vi "TLB Native Dynamic Events ver 0.18.vi"() -> ()   [LabVIEW 2018]
uses:
  Labview Training Phase 2/Enum Controls/States for Action Engine.ctl
  TLB Type Definitions/State Type Definitions, for 0.26g versions and later 2.ctl
  TLB Type Definitions/Intruction Type Definitions.ctl
  TLB Type Definitions/Encoder cluster.ctl
  TLB Type Definitions/PING CLUSTER.ctl
  <vilib>/Studica/Studica Toolkit/NavX/NavX.lvlib
  <vilib>/Studica/Studica Toolkit/Background/DIO Channel.ctl
  Underlying VI's/NavX VI/navX type def.ctl
  <vilib>/Studica/Studica Toolkit/Background/I2C Channel.ctl
  TLB Type Definitions/Vision cluster.ctl
  <vilib>/NI_Real-Time Target Support.lvlib
  TLB Type Definitions/Stepper cluster.ctl
  Experimental VI's/Archived VI's/MOTOR CONTROL NO PID Type Def.ctl
  Underlying VI's/I2C Master VI/I2C MASTER Type Def.ctl
  Underlying VI's/I2C Master VI/I2C_MASTER_WRITE_NEW Type Def.ctl
  <vilib>/userdefined/High Color/IMAQdx.ctl
  Underlying VI's/I2C Master VI/Arduino_Interfacing.ctl
  TLB Type Definitions/Yaw Cluster.ctl
  TLB Type Definitions/Time cluster.ctl
  TLB Type Definitions/Y Stepper cluster.ctl
  Underlying VI's/Modified webcam FGV/Webcam AE.ctl
  Underlying VI's/Elasped Timer/Elapsed timer control.ctl
  Underlying VI's/Motor Control VI with PID/MOTOR CONTROL WITH PID AE DATA MODE TYPE DEF.ctl
  Underlying VI's/Motor Control VI with PID/MOTOR CONTROL WITH PID AE DIRECTION TYPE DEF.ctl
  TLB Type Definitions/IR Sensor Type Def.ctl
  <vilib>/myRIO/Common/Instrument Driver Framework/myRIO v1.0/AI/typedefs/AI Channels Enum.ctl
  <vilib>/myRIO/Common/Instrument Driver Framework/myRIO v1.0/AI/typedefs/AI Channels List.ctl
  TLB Type Definitions/Motor Speed Cluster.ctl
  <vilib>/Utility/RT CPU Load.ctl
panel:
  out "x-y":dbl
  out "Left IR Sensor":dbl
  out "Obstacle detected":bool
  out "Speed & distance":T1
  out "Object Center Coordinates":cluster{"x":sgl, "y":sgl}
  out "Object detection cluster":T2
  out "Time up flag":bool
  out "Task selection":u8
  in  "Object recognition mode":enum16{"Ball", "Soap", "Gel", "Pipe", "None"}(ring)
  out "NavX Readings":T3
  out "Arduino Data":T4
  out "CPU loads":T5[](array[typedef]) {"ISR (%)" format="%#.2f"; "Idle (%)" format="%#.2f"; "Background (%)" format="%#.2f"; "Normal (%)" format="%#.2f"; "Above Normal (%)" format="%#.2f"; "High (%)" format="%#.2g"; "Timed Structures (%)" format="%#.2g"; "Time Critical (%)" format="%#.2g"; "Total (%)" format="%#.2g"}
  out "TASK ENABLE":bool
  out "Rising Edge":bool
  in  "Green LED":bool
  out "I2C Error":errorcluster
  out "State Logic":T6=enum."Startup"
  out "elements":T7[](array[typedef])
  in  "STOP TASK":bool
  in  "OK Button":bool
  in  "STOP":bool
  out "error out":errorcluster
  out "Action Queue Items":i32
  out "State Logic Queue Items":i32
  out "Action Queues items":string[](array[string])=["Hardware reset", "Software reset", ""]
  out "Action State":string
  # "System Health Status Update"
  # "VISION"
  # "TLB FRAMEWORK STATUS"
  # "Test Programme written by Calvin Loke    Dated: 28 Aug 2019\nTest Programme revised by Dr Alex See   Dated 30 Aug 2019\n\nRevision date: 20/03/2020\nProgramme version:   TLB Native Dynamic Events ver 0.14a"
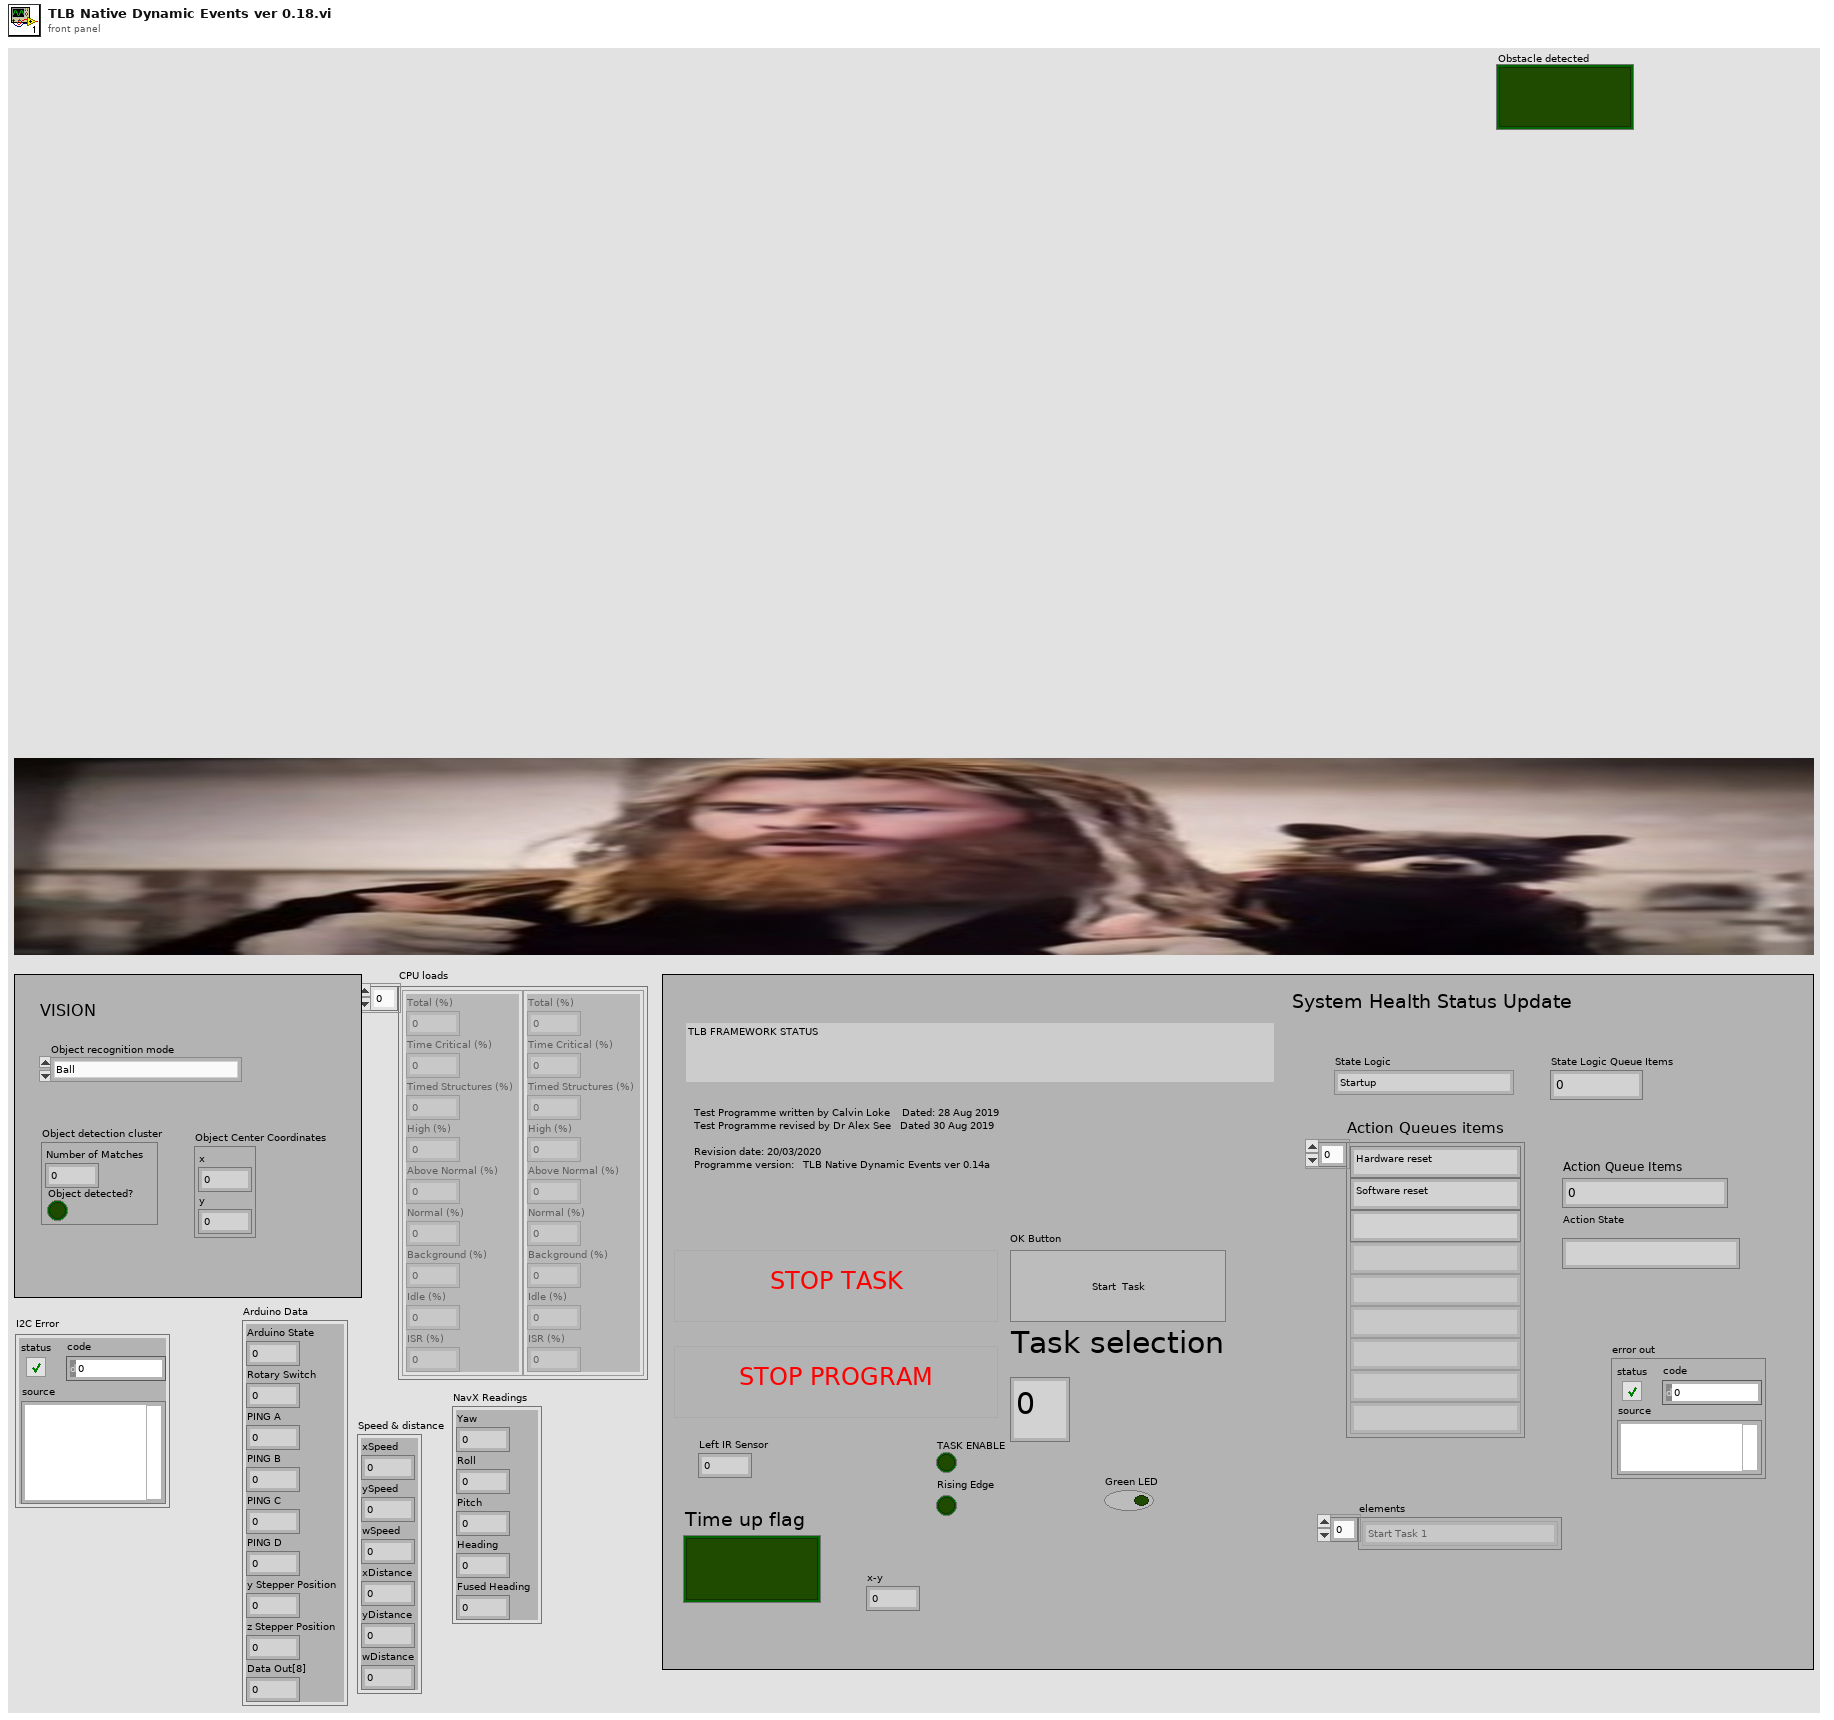
[diagram p1: front panel]
types:
  T1 = cluster{"xSpeed":dbl, "ySpeed":dbl, "wSpeed":dbl, "xDistance":dbl, "yDistance":dbl, "wDistance":dbl}
  T2 = cluster{"Number of Matches":i32, "Object detected?":bool}
  T3 = cluster{"Yaw":dbl, "Roll":dbl, "Pitch":dbl, "Heading":dbl, "Fused Heading":dbl}
  T4 = cluster{"Arduino State":u8, "Rotary Switch":u8, "PING A":u8, "PING B":u8, "PING C":u8, "PING D":u8, "y Stepper Position":u8, "z Stepper Position":u8, "Data Out[8]":u8}
  T5 = typedef "NI_Real-Time Target Support.lvlib/RT CPU Load.ctl" = cluster{"Total (%)":dbl, "Time Critical (%)":dbl, "Timed Structures (%)":dbl, "High (%)":dbl, "Above Normal (%)":dbl, "Normal (%)":dbl, "Background (%)":dbl, "Idle (%)":dbl, "ISR (%)":dbl}
  T6 = typedef "State Type Definitions, for 0.26g versions and later 2.ctl" = enum16{"None", "Startup", "Move to Angle", "True Stop", "Idle", "Shutdown", "Task 1A", "Task 1B", "Task 2:Raise Arm", "Task 2:Sensor Mode", "Task 2:Reverse Mode", "Task 3", "Task 4_A", "Task 4_B", "Task 4_C", "Task 4_D", "Task 5A", "Task 5B", "Task 5C", "Task 5D", "Task 5E: POSITION ARM", "Task 5F: ARM GRAB HEIGHT", "Task 5G: CLOSE CLAW", "Task 5H: RAISE ARM", "Task 6_A", "Task 6_B", "Task 7", "Task 8A: RAISE ARM", "Task 8B: MOVE TO BOX", "Task 8C: CAM BURST", "Task 8D: PROCESS IMAGE", "Task 8E: ROBOT ADJUST", "Task 8F: CAM BURST 2", "Task 8G: PROCESS IMAGE 2", "Task 8H: ARM ADJUST", "Task 8I: ARM GRAB HEIGHT", "Task 8J: CLOSE CLAW", "Task 8K: RAISE MY SWORD", "Task 9A: Raise Arm", "Task 9B: Rotate to Angle", "Task 9C: Detect Box", "Task 9D: MOVE FORWARD", "Task 9E: MOVE LEFT", "Task 9F: SCAN BOX", "Task 9G: MOVE RIGHT", "Task 9H: SCAN BOX 2", "Task 9I: ROTATE 90 CW", "Task 9J: FORWARD", "Task 9K: MOVE RIGHT", "Task 9L: SCAN BOX 3", "Task 9M: MOVE RIGHT", "Task 9N: SCAN BOX 4", "PENIS", "PENIS 2", "PENIS 3", "Task 9R: PROCESS COLOUR", "Task A1: Task 9 Open cam", "Task A2: Task 9 Move Arm", "Task A3: Task 9 Set Timer", "Task A4: Tasl 9 Capture images", "Task A5: Task 9 Close camera", "Task A6: Process Colour", "Task A7: Dispose Camera Buffer"}
  T7 = typedef "Intruction Type Definitions.ctl" = enum16{"None", "Start Task 1", "Start Task 2", "Start Task 3", "Start Task 4", "Start Task 5", "Start Task 6", "Start Task 7", "Start Task 8 - BALL", "Start Task 8 - Gel", "Start Task 8 - Pipe", "Start Task 8 - Soap", "Start Task 9", "Start Task A", "Start Task B", "Exit"}
  T8 = typedef "Motor Speed Cluster.ctl" = cluster{"ySpeed":dbl, "xSpeed":dbl, "wSpeed":dbl}
  T9 = typedef "IR Sensor Type Def.ctl" = cluster{"Left IR Sensor":dbl, "Arm IR Sensor":dbl, "Bottom IR Sensor":dbl}
  T10 = typedef "Y Stepper cluster.ctl" = cluster{"yStepper desired":u8}
  T11 = typedef "Time cluster.ctl" = cluster{"Time up flag":bool, "SET TIME TO CHECK":dbl}
  T12 = typedef "Yaw Cluster.ctl" = cluster{"Yaw":dbl, "Compass":dbl}
  T13 = typedef "Stepper cluster.ctl" = cluster{"y Stepper Position":u8, "z Stepper Position":u8}
  T14 = typedef "DIO Channel.ctl" = enum16{"Not Connected", "A/DIO1", "A/DIO2", "A/DIO3", "A/DIO4", "A/DIO5", "A/DIO6", "A/DIO7", "A/DIO13", "B/DIO1", "B/DIO2", "B/DIO3", "B/DIO4", "B/DIO5", "B/DIO6", "B/DIO7", "B/DIO13", "C/DIO0", "C/DIO1", "C/DIO2", "C/DIO3", "C/DIO4", "C/DIO5", "C/DIO6", "C/DIO7"}
  T15 = typedef "Vision cluster.ctl" = cluster{"Recognized Object":bool, "Object X coordinate":dbl, "Object Y coordinate":dbl}
  T16 = typedef "PING CLUSTER.ctl" = cluster{"PING_A":u8, "PING_B":u8, "PING_C":u8, "PING_D":u8}
  T17 = typedef "Encoder cluster.ctl" = cluster{"xDistance":dbl, "yDistance":dbl, "wDistance":dbl}
  T18 = cluster{"DIO Channel":T14, "FPGA VI Reference Out":refnum<k20>}
  T19 = typedef "navX type def.ctl" = enum16{"Get i2C reference", "Read Values", "Zero Yaw"}
  T20 = typedef "Arduino_Interfacing.ctl" = enum16{"Initialize", "Write to Arduino", "Read From Arduino"}
  T21 = typedef "I2C Channel.ctl" = enum16{"Not Connected", "A", "B"}
  T22 = typedef "States for Action Engine.ctl" = enum16{"Initialize", "Write", "Read"}
  T23 = cluster{"I2C Ref Out":cluster{"I2C Channel":T21, "FPGA VI Reference Out":refnum<k20>}, "Connected":bool, "Slave Address (7-bit)":u8, "Registry":u8[]}
  T24 = typedef "IMAQ Image.ctl" = refnum<image>
  T25 = typedef "Intruction Type Definitions.ctl" = enum16{"None", "Start Task 1", "Start Task 2", "Start Task 3", "Start Task 4", "Start Task 5", "Start Task 6", "Start Task 7", "Start Task 8", "Start Task 9", "Start Task A", "Start Task B", "Exit"}
  T26 = typedef "State Type Definitions.ctl" = enum16{"None", "Startup", "Move to Angle", "True Stop", "Idle", "Shutdown", "Task 1", "Task 2:Raise Arm", "Task 2:Sensor Mode", "Task 2:Reverse Mode", "Task 3", "Task 4_A", "Task 4_B", "Task 4_C", "Task 4_D", "Task 5A: ARM CAM HEIGHT", "Task 5B: MOVE TO BOX", "Task 5C: CAM BURST", "Task 5D: PROCESS IMAGE", "Task 5E: POSITION ARM", "Task 5F: ARM GRAB HEIGHT", "Task 5G: CLOSE CLAW", "Task 5H: RAISE ARM", "Task 6_A", "Task 6_B", "Task 7", "Task 8A: RAISE ARM", "Task 8B: MOVE TO BOX", "Task 8C: CAM BURST", "Task 8D: PROCESS IMAGE", "Task 8E: ROBOT ADJUST", "Task 8F: CAM BURST 2", "Task 8G: PROCESS IMAGE 2", "Task 8H: ARM ADJUST", "Task 8I: ARM GRAB HEIGHT", "Task 8J: CLOSE CLAW", "Task 8K: RAISE MY SWORD", "Task 9A: Raise Arm", "Task 9B: Rotate to Angle", "Task 9C: Rotation alignmnet", "Task B"}
  T27 = typedef "MOTOR CONTROL WITH PID AE DIRECTION TYPE DEF.ctl" = enum16{"y-axis movement", "x-axis movement", "rotation", "stop", "reset encoders"}
  T28 = typedef "MOTOR CONTROL WITH PID AE DATA MODE TYPE DEF.ctl" = enum16{"Init AE", "Write to AE", "Read from AE"}
  T29 = typedef "Elapsed timer control.ctl" = enum16{"Start", "Pause", "Initialize"}
  T30 = typedef "I2C_MASTER_WRITE_NEW Type Def.ctl" = enum16{"Ultrasonic sensors", "Stepper origin", "zStepper 13.3k", "zStepper 13k", "zStepper 12k", "zStepper 11k", "zStepper 10k", "zStepper 9k", "zStepper 8k", "zStepper 7k", "zStepper 6k", "zStepper 5k", "zStepper 4k", "zStepper 3k", "zStepper 2k", "zStepper 1k", "zStepper 900", "zStepper 800", "zStepper 700", "zStepper 600", "zStepper 500", "zStepper 400", "zStepper 300", "zStepper 200", "zStepper 100", "zStepper 0", "yStepper control", "Open Claw", "Close Claw", "Soft Reset"}
  T31 = typedef "Webcam AE.ctl" = enum16{"Initialize Camera", "Open Camera", "Continuous Acquisition", "Close Camera", "Retrieve Image", "Dispose Camera Image Buffer"}
  T32 = typedef "IMAQdx.ctl" = refnum<k21>
  T33 = typedef "Webcam AE.ctl" = enum16{"Initialize Camera", "Open Camera", "Continuous Acquisition", "Close Camera", "Retrieve Image", "Dispose Image Buffers"}
  T34 = typedef "MOTOR CONTROL NO PID Type Def.ctl" = enum16{"Init", "Front Back", "Left Right", "Rotate", "Stop", "Latch"}
  T35 = typedef "AI Channels List.ctl" = T36[]
  T36 = typedef "AI Channels Enum.ctl" = enum16{"Not Connected", "AudioIn/Left", "AudioIn/Right", "C/AI0", "C/AI1", "A/AI0", "A/AI1", "A/AI2", "A/AI3", "A/AI4", "A/AI5", "A/AI6", "A/AI7", "B/AI0", "B/AI1", "B/AI2", "B/AI3", "B/AI4", "B/AI5", "B/AI6", "B/AI7", "AI/AI0", "AI/AI1", "AI/AI2", "AI/AI3", "A/AI0 (DIFF)", "A/AI1 (DIFF)", "A/AI2 (DIFF)", "A/AI3 (DIFF)", "B/AI0 (DIFF)", "B/AI1 (DIFF)", "B/AI2 (DIFF)", "B/AI3 (DIFF)"}
  T37 = typedef "I2C MASTER Type Def.ctl" = enum16{"Last State", "Mode 0", "Mode 1", "Mode 2", "Mode 3", "Mode 4", "Mode 5", "Mode 6", "Mode 7", "Mode 8", "Mode 9", "Mode 10"}
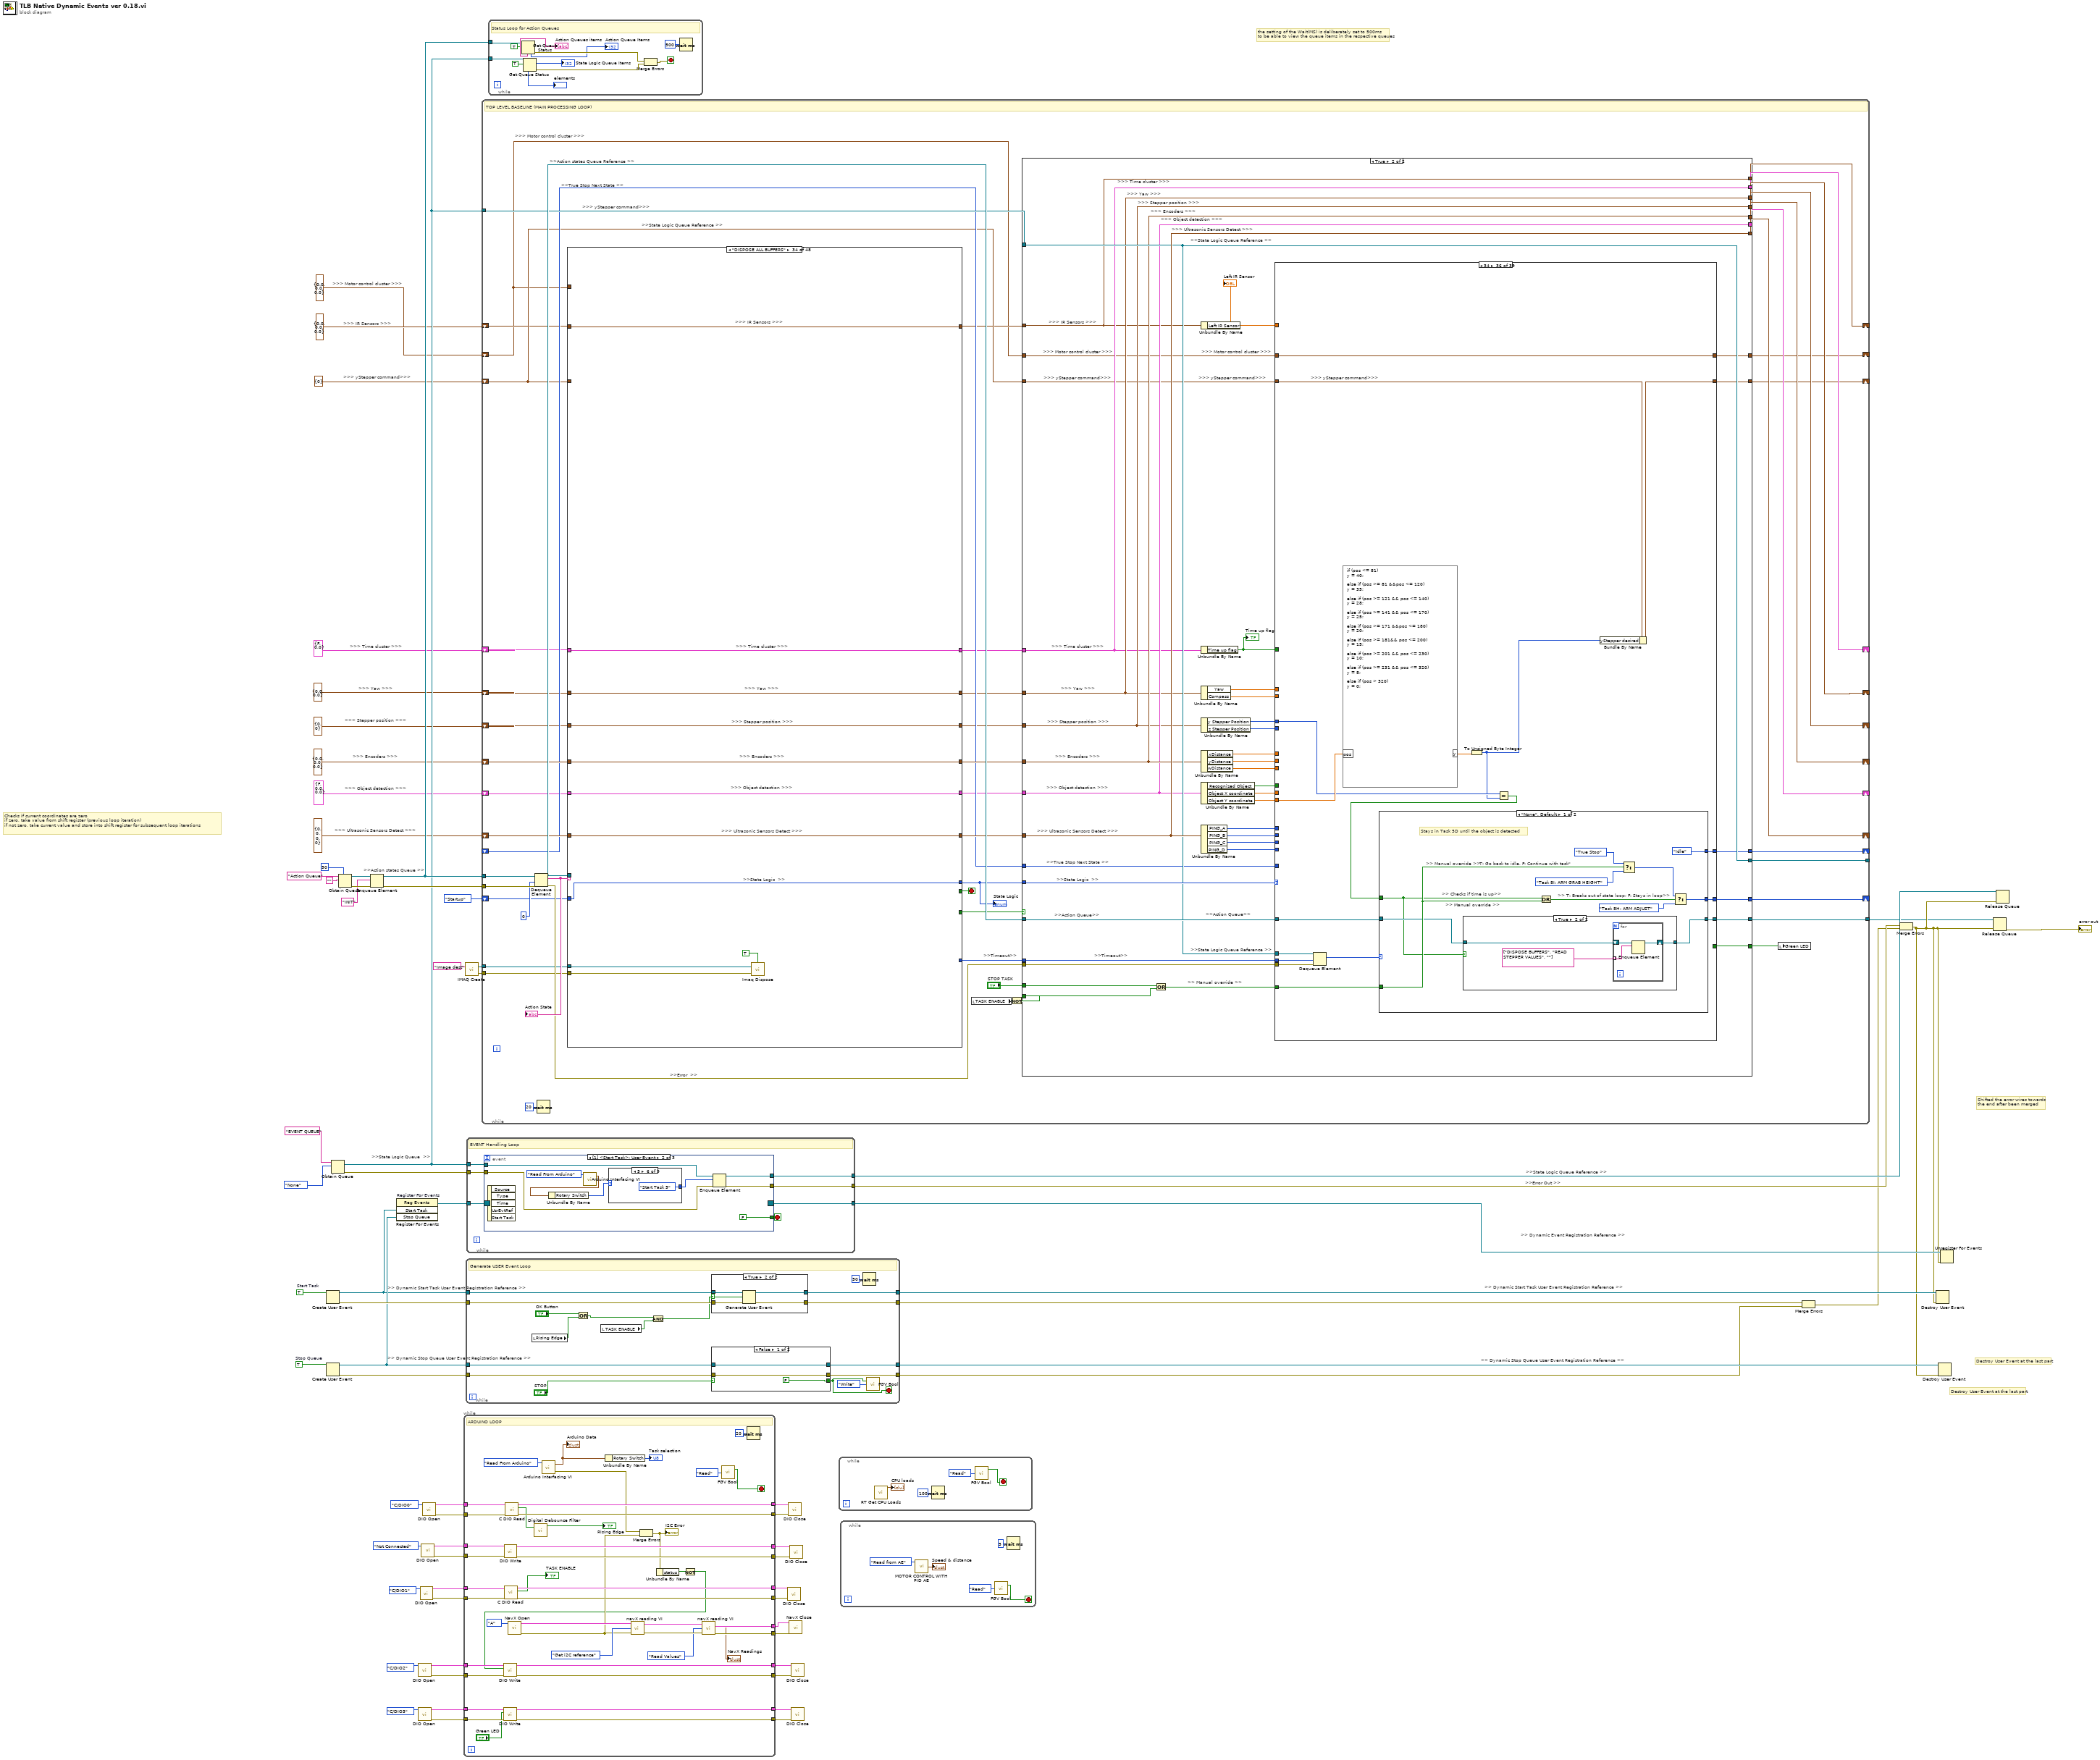
[diagram p0: block diagram]
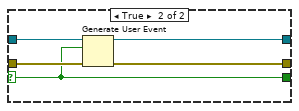
[diagram p2: hidden frame]
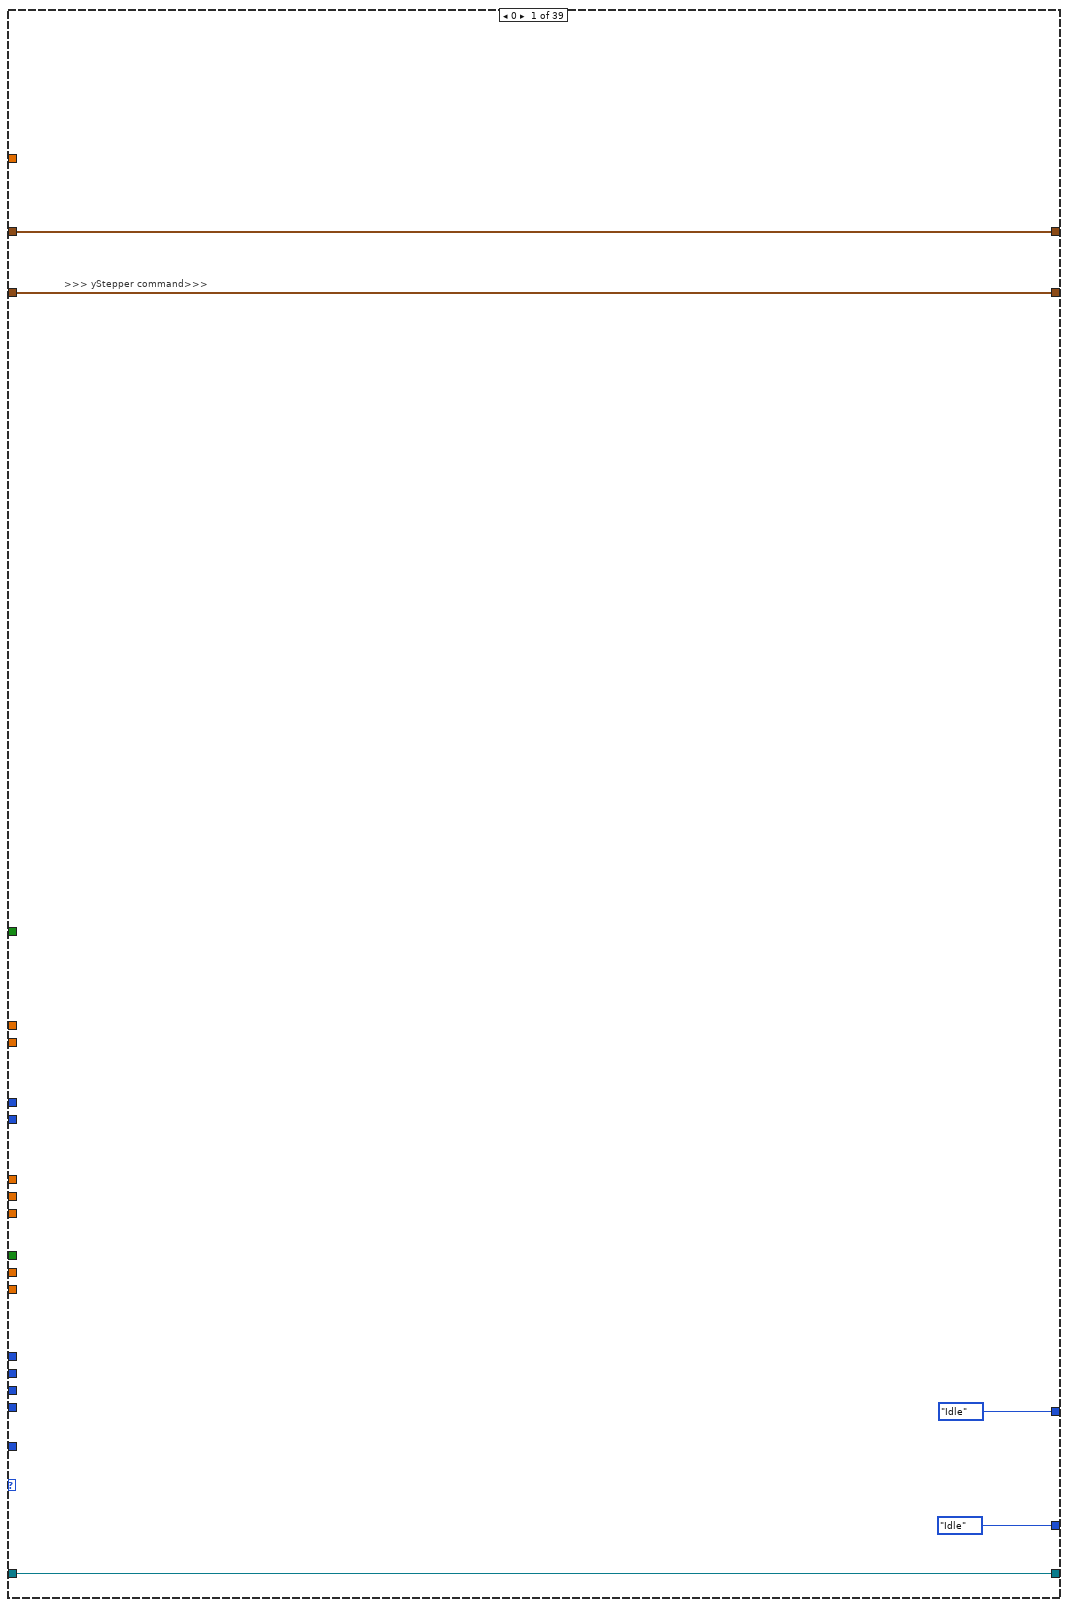
[diagram p5: hidden frame]
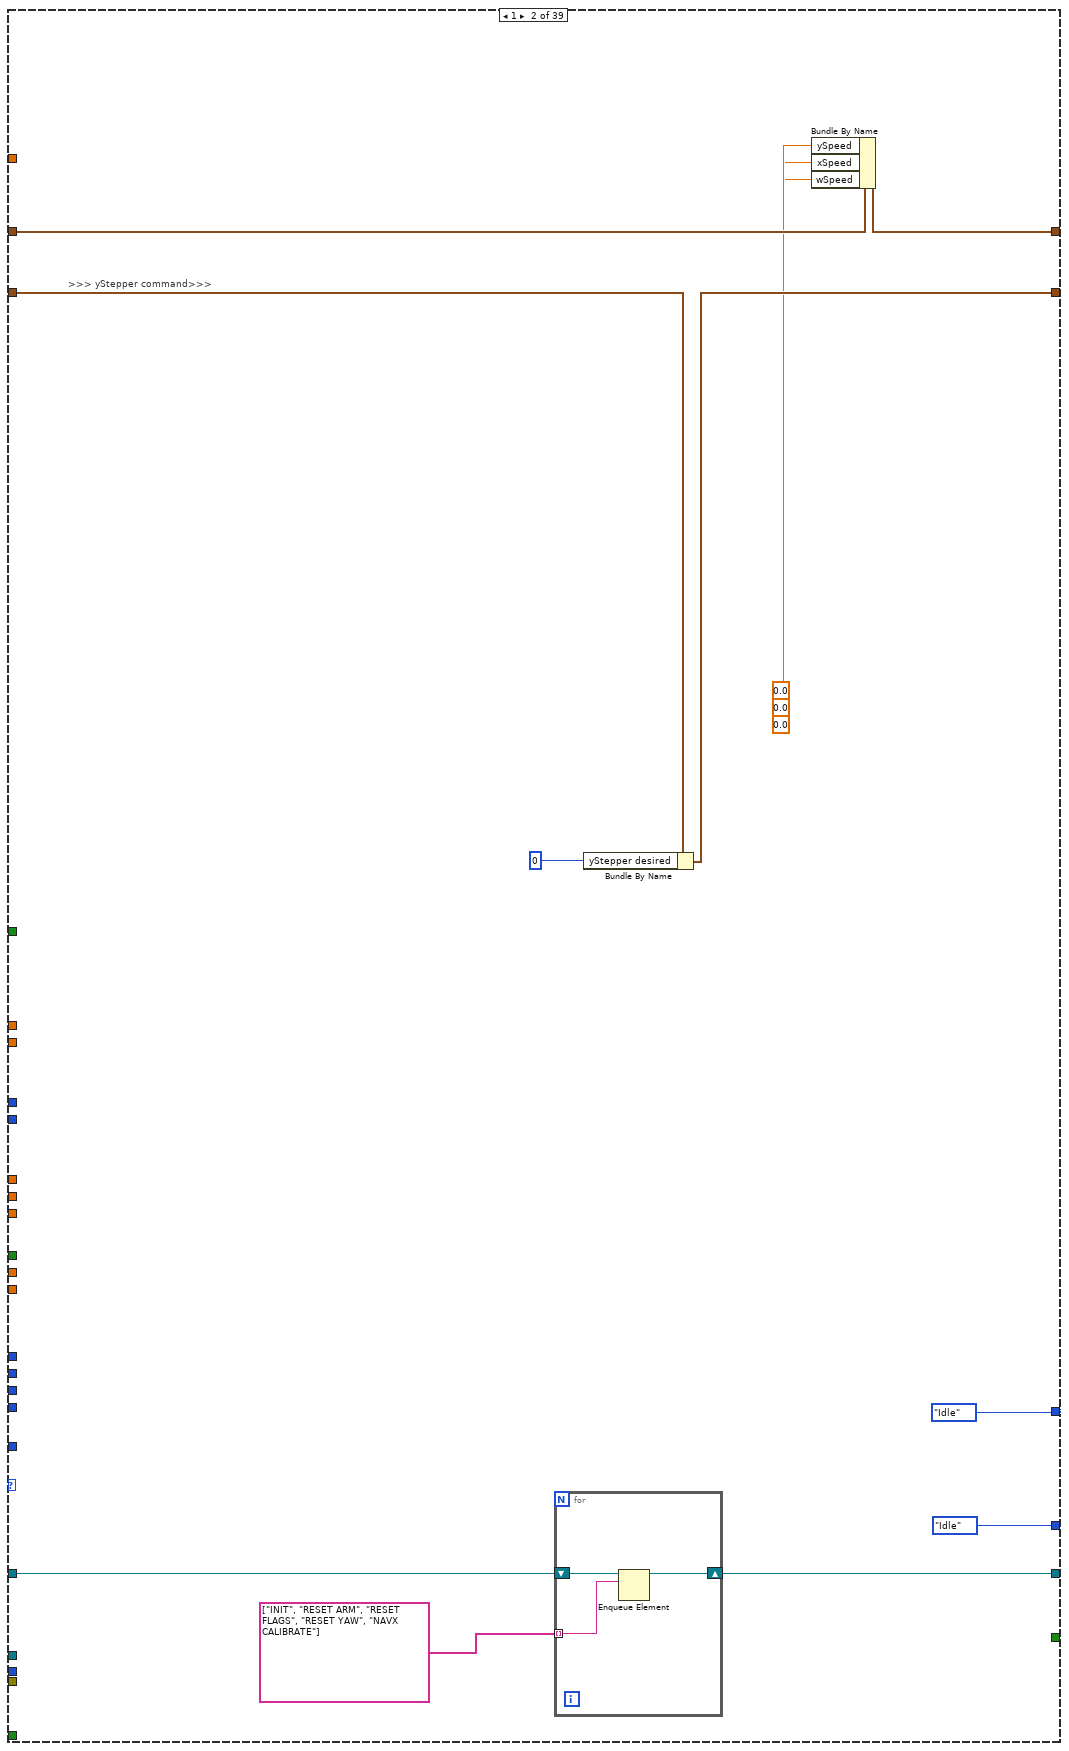
[diagram p6: hidden frame]
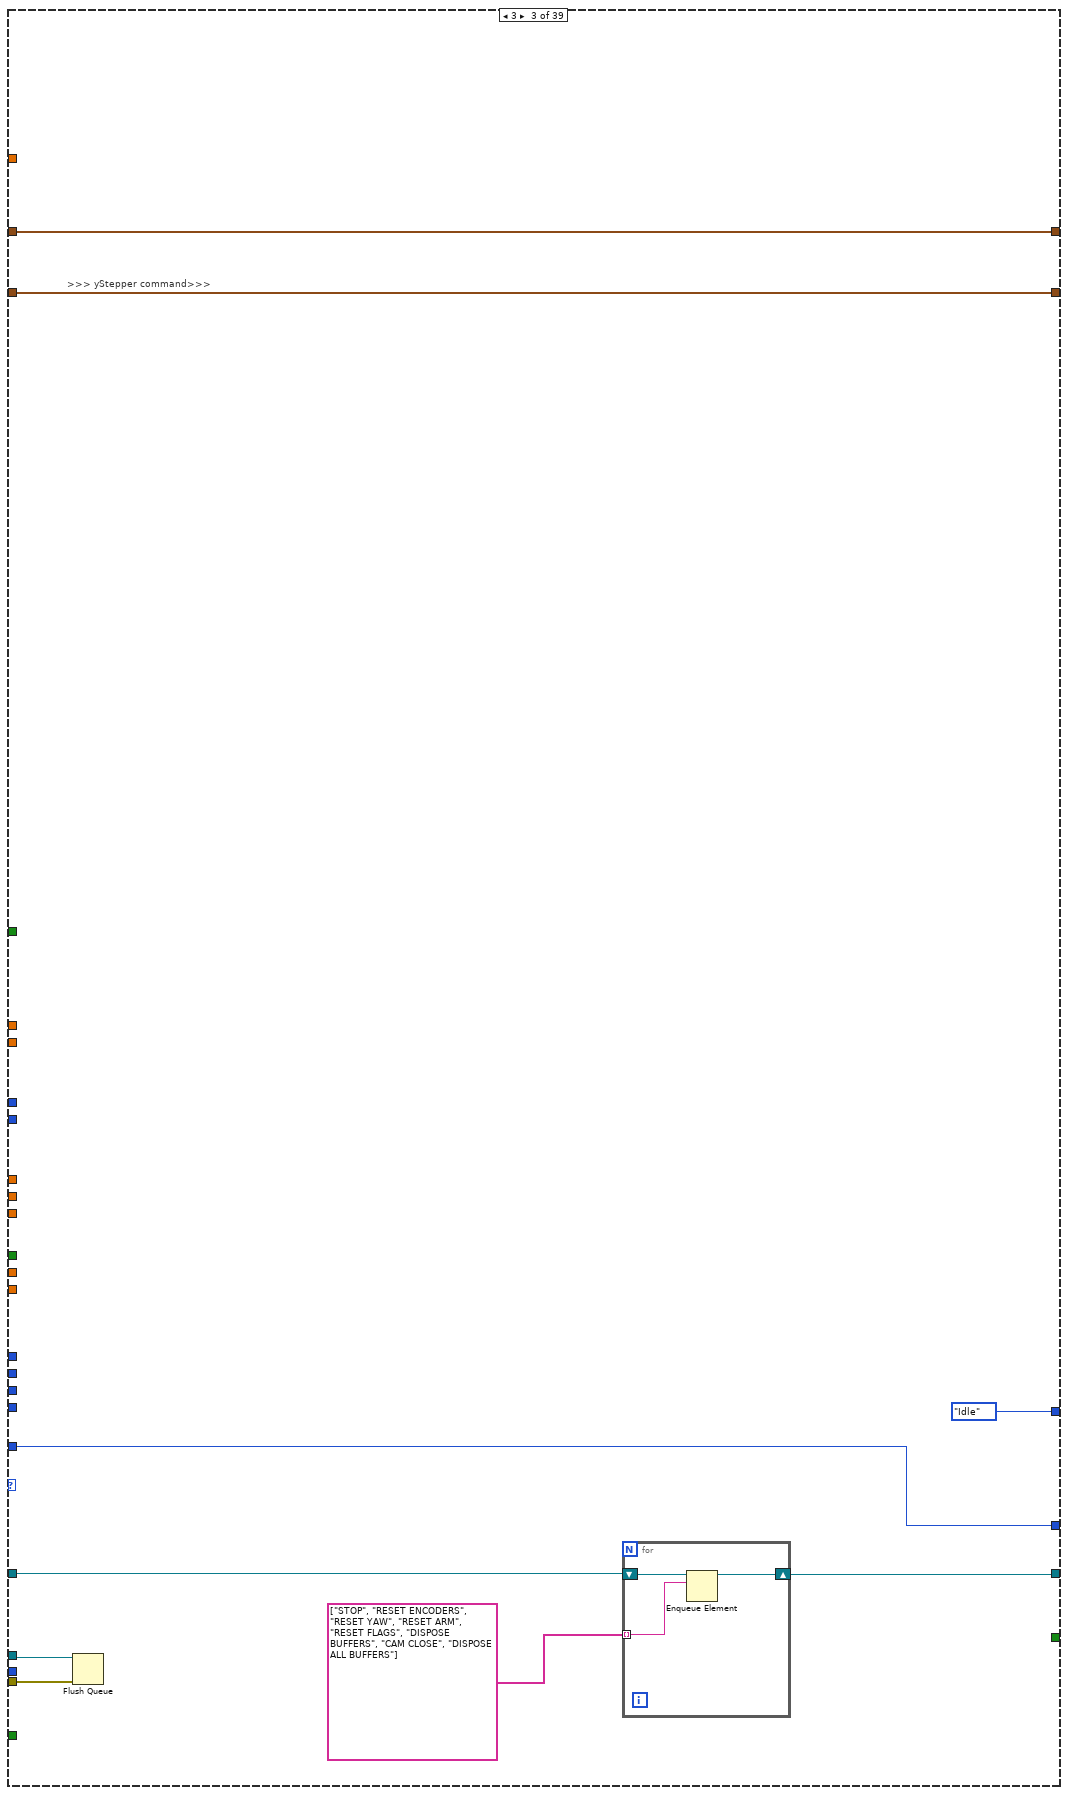
[diagram p7: hidden frame]
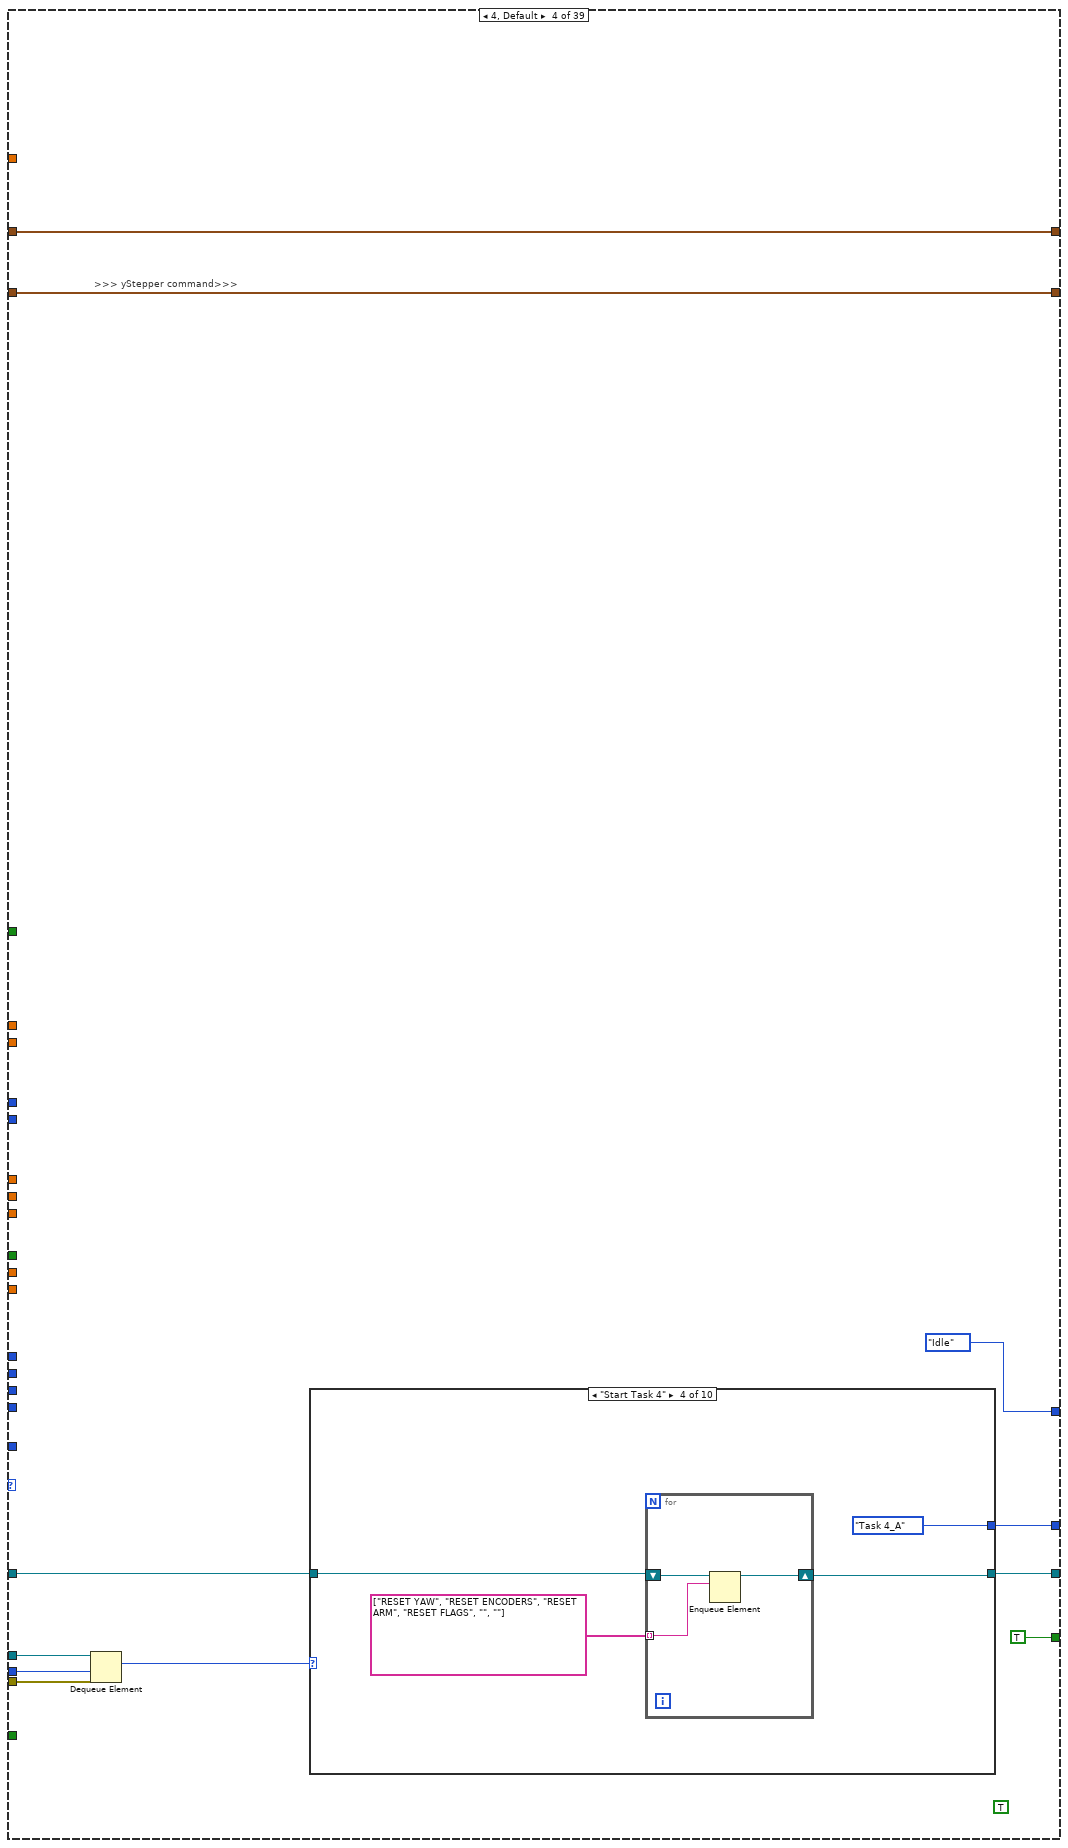
[diagram p8: hidden frame]
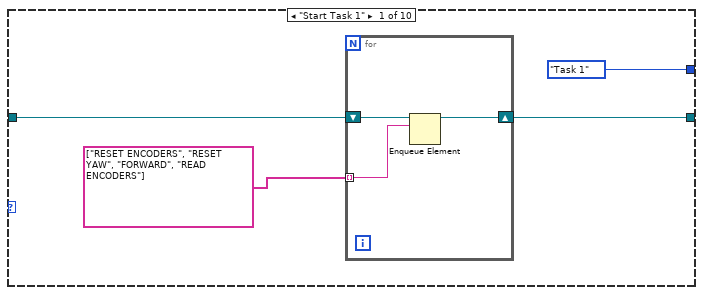
[diagram p9: hidden frame]
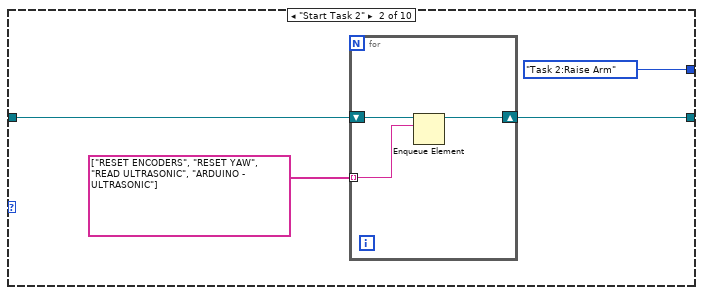
[diagram p10: hidden frame]
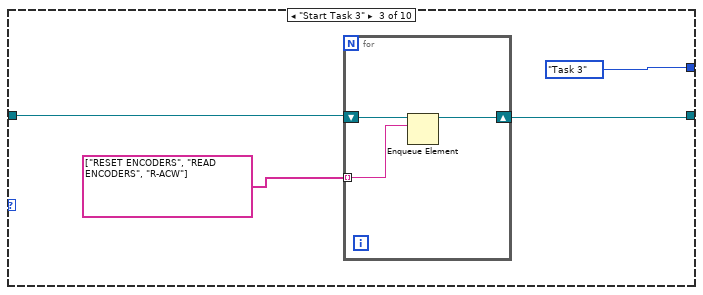
[diagram p11: hidden frame]
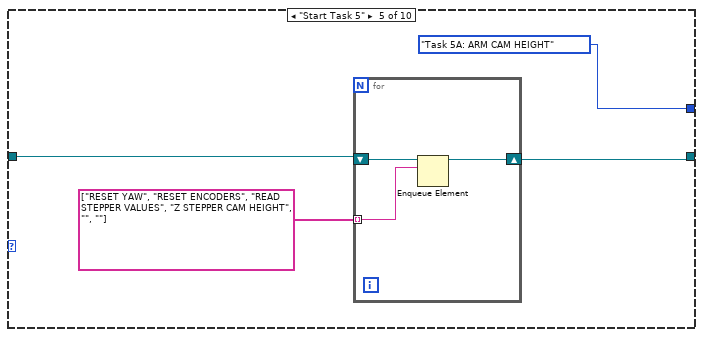
[diagram p12: hidden frame]
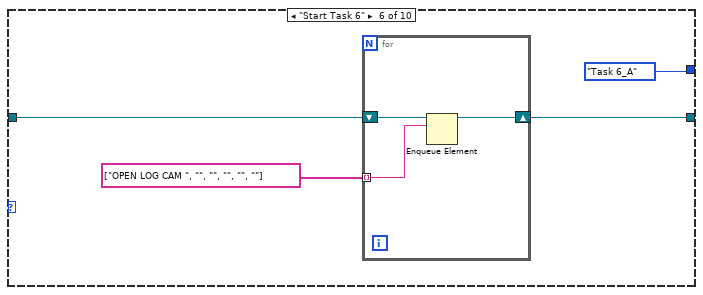
[diagram p13: hidden frame]
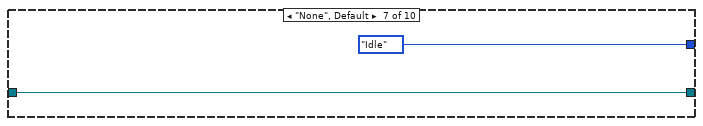
[diagram p14: hidden frame]
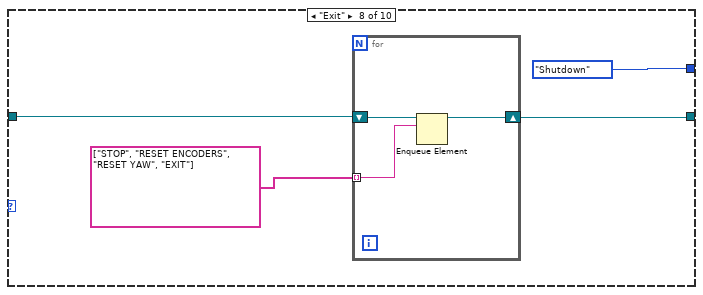
[diagram p15: hidden frame]
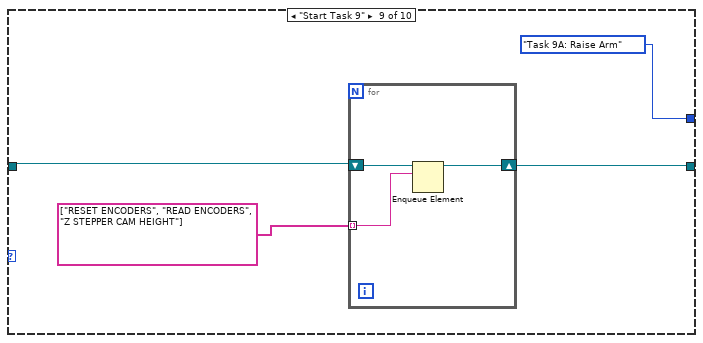
[diagram p16: hidden frame]
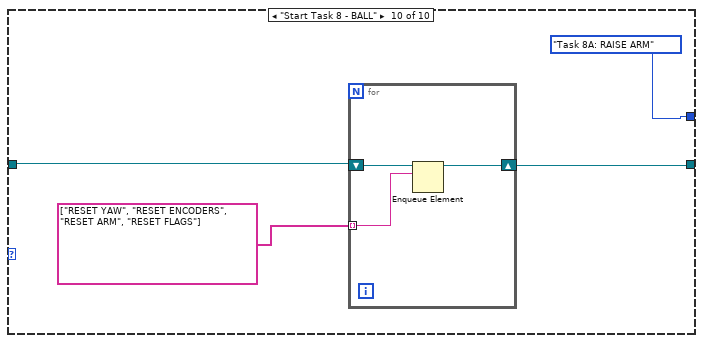
[diagram p17: hidden frame]
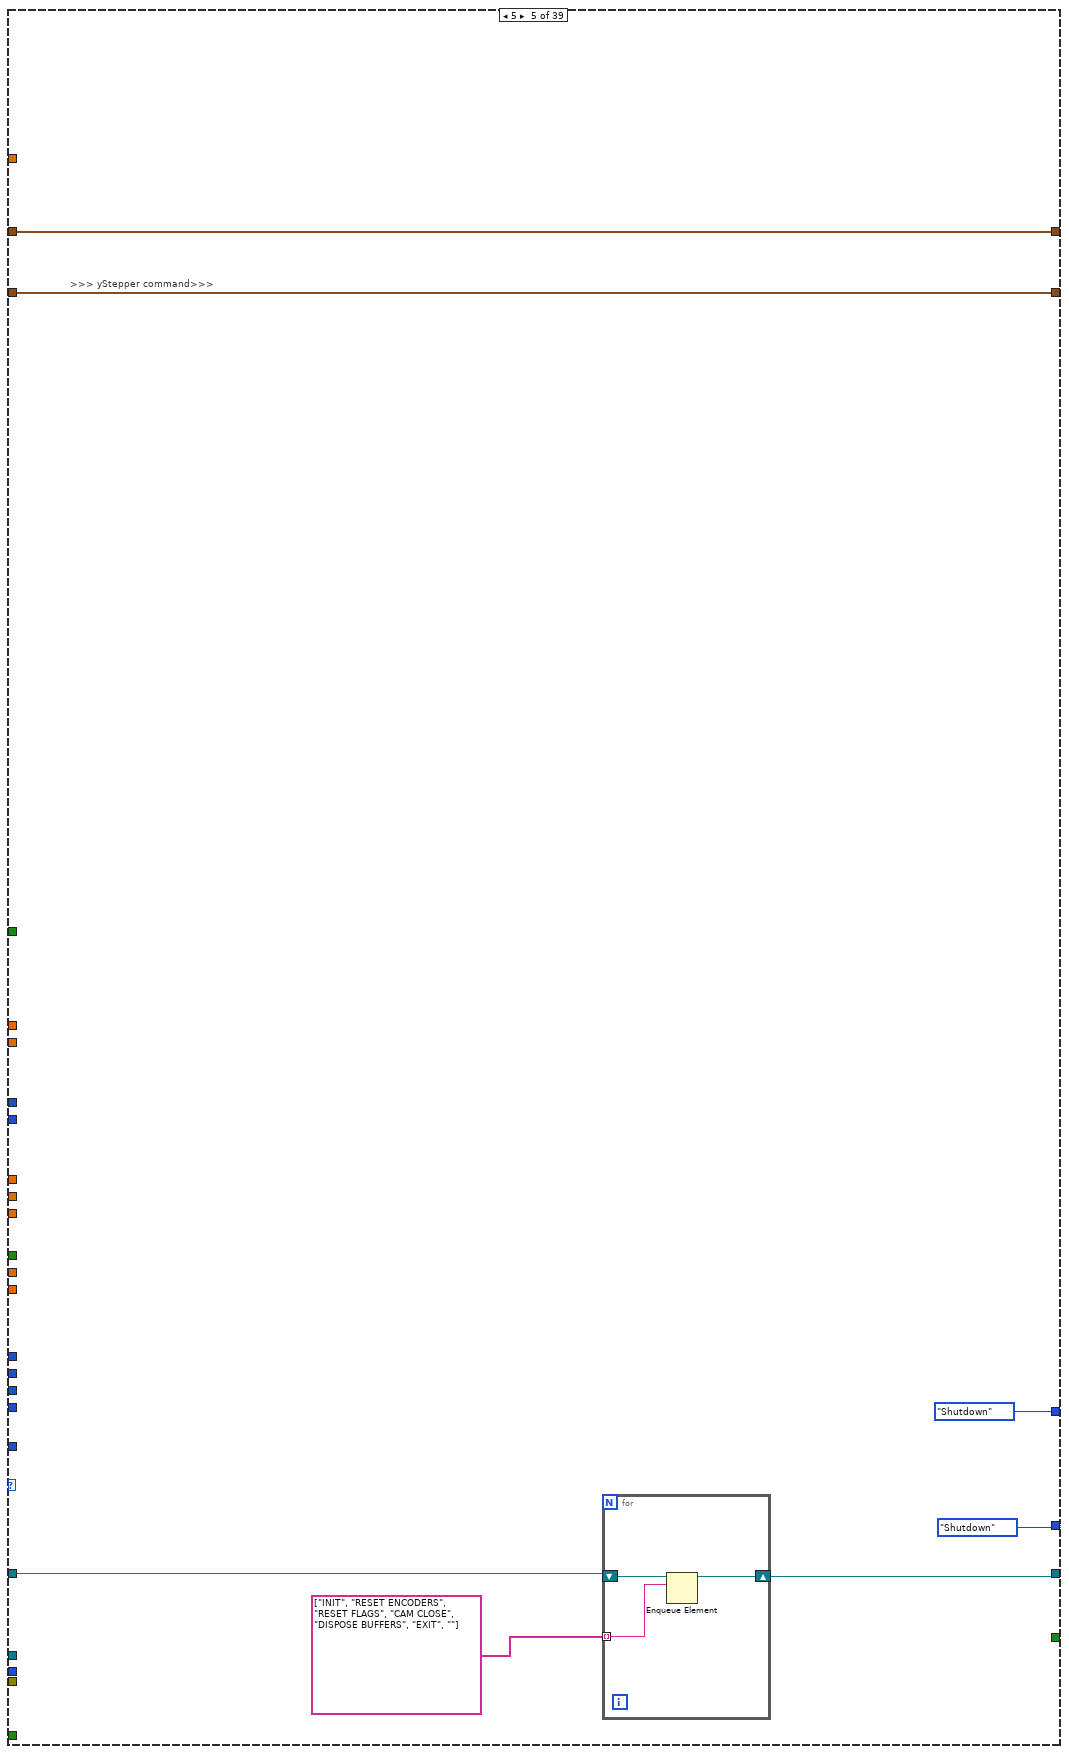
[diagram p18: hidden frame]
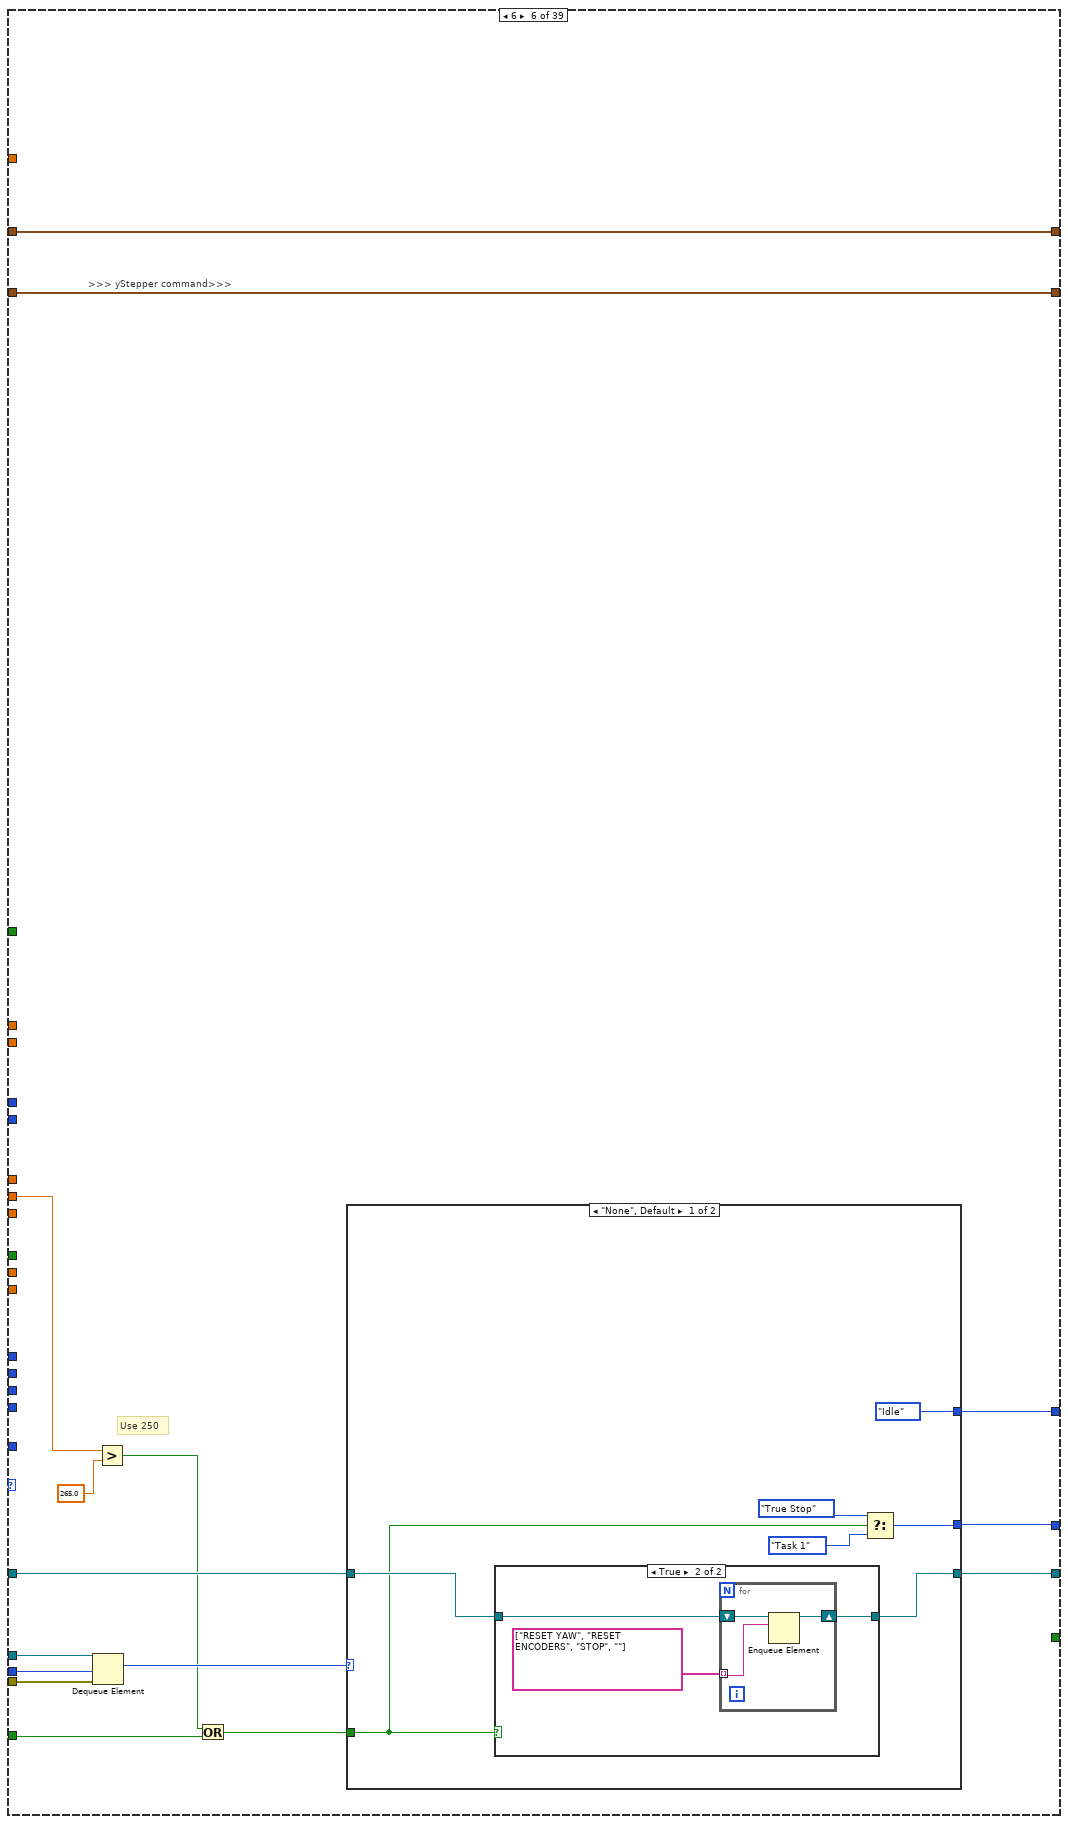
[diagram p19: hidden frame]
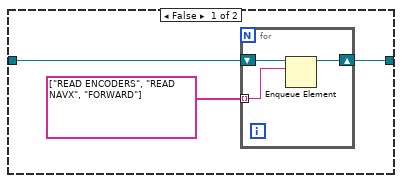
[diagram p20: hidden frame]
diagram:
  w70 = TRUE  # Stop Queue
  w69 = TRUE  # Start Task
  # ">>> Motor control cluster >>>"
  # ">>> IR Sensors >>>"
  # "Checks if current coordinates are zero\nif zero, take value from shift register (previous loop iteration)\nif not zero, take current value and store into shift register for subsequent loop iterations"
  # ">>> yStepper command>>>"
  # ">>> Time cluster >>>"
  # ">>> Yaw >>>"
  # ">>> Stepper position >>>"
  # ">>> Encoders >>>"
  # ">>> Object detection >>>"
  # ">>> Ultrasonic Sensors Detect >>>"
  # "the setting of the Wait(MS) is deliberately set to 500ms\nto be able to view the queue items in the respective queues"
  # ">>Error Out >>"
  # ">> Dynamic Stop Queue User Event Registration Reference >>"
  # ">> Dynamic Start Task User Event Registration Reference >>"
  # ">> Dynamic Stop Queue User Event Registration Reference >>"
  # ">> Dynamic Start Task User Event Registration Reference >>"
  # ">> Dynamic Event Registration Reference >>"
  # ">>Action states Queue >>"
  # ">>State Logic Queue  >>"
  # ">>State Logic Queue Reference >>"
  # "Destroy User Event at the last part"
  # "Destroy User Event at the last part"
  # "Shifted the error wires towards\nthe end after been merged"
  n1 = Create User Event(user event datatype=w69) -> (user event=w61:refnum<user-event>, error out=w66:errorcluster)  [unwired: 1 in]
  n2 = Create User Event(user event datatype=w70) -> (user event=w62:refnum<user-event>, error out=w65:errorcluster)  [unwired: 1 in]
  n3 = Obtain Queue(name (unnamed)="EVENT QUEUE", element data type=Intruction_Type_Definitions."None" ("Enum")) -> (queue out=w47:refnum<queue>, error out=w53:errorcluster)  [unwired: 3 in, 1 out]
  n4 = Obtain Queue(max queue size (-1, unlimited)=50, name (unnamed)="Action Queue", element data type="") -> (queue out=w56:refnum<queue>, error out=w52:errorcluster)  [unwired: 2 in, 1 out]
  n5 = Enqueue Element(queue=w56, element="INIT", error in (no error)=w52) -> (queue out=w48:refnum<queue>, error out=w51:errorcluster)  [unwired: 1 in, 1 out]
  n6 = register-events "Register For Events"(w61, w62) -> (reference out=w60:refnum<event-registration>)  [unwired: 2 in, 1 out]
  n7 = call <vilib>:"DIO Open.vi"("DIO Channel"=DIO_Channel."C/DIO2") -> ("error out"=w17:errorcluster, "DIO Info Out"=w18:T18)  [unwired: 9 in]
  n8 = call <vilib>:"DIO Open.vi"("DIO Channel"=DIO_Channel."C/DIO3") -> ("error out"=w12:errorcluster, "DIO Info Out"=w13:T18)  [unwired: 9 in]
  n9 = call <vilib>:"DIO Open.vi"("DIO Channel"=DIO_Channel."C/DIO1") -> ("error out"=w25:errorcluster, "DIO Info Out"=w26:T18)  [unwired: 9 in]
  n10 = call <vilib>:"DIO Open.vi"("DIO Channel"=DIO_Channel."Not Connected") -> ("error out"=w30:errorcluster, "DIO Info Out"=w32:T18)  [unwired: 9 in]
  n11 = call <vilib>:"DIO Open.vi"("DIO Channel"=DIO_Channel."C/DIO0") -> ("error out"=w35:errorcluster, "DIO Info Out"=w38:T18)  [unwired: 9 in]
  n12 = while {
    tunnel: w38 -> [w111]
    tunnel: [w110] -> w36
    tunnel: w35 -> [w109]
    tunnel: [w108] -> w34
    tunnel: w32 -> [w105]
    tunnel: [w104] -> w31
    tunnel: w30 -> [w103]
    tunnel: [w102] -> w29
    tunnel: [w101] -> w27
    tunnel: w26 -> [w100]
    tunnel: w25 -> [w99]
    tunnel: [w98] -> w24
    tunnel: w18 -> [w92]
    tunnel: w17 -> [w91]
    tunnel: [w90] -> w16
    tunnel: [w89] -> w15
    tunnel: w13 -> [w88]
    tunnel: w12 -> [w87]
    tunnel: [w86] -> w11
    tunnel: [w85] -> w10
    tunnel: [w79] -> w7
    tunnel: [w78] -> w8
    stop <- w113 stop-if-true
    # "ARDUINO LOOP"
    n13 = call <vilib>:"DIO Write.vi"("error in (no error)"=w87, "Input"="Green LED", "DIO Info In"=w88) -> ("error out"=w85:errorcluster, "DIO Info Out"=w86:T18)  [unwired: 7 in]
    n14 = call <vilib>:"DIO Write.vi"("error in (no error)"=w103, "DIO Info In"=w105) -> ("error out"=w102:errorcluster, "DIO Info Out"=w104:T18)  [unwired: 8 in]
    n15 = call <vilib>:"C DIO Read.vi"("error in (no error)"=w99, "DIO Info In in"=w100) -> ("error out"=w98:errorcluster, "IN"=→"TASK ENABLE":bool, "DIO Info In out"=w101:T18)  [unwired: 7 in]
    n16 = call <vilib>:"C DIO Read.vi"("error in (no error)"=w109, "DIO Info In in"=w111) -> ("error out"=w108:errorcluster, "IN"=w107:bool, "DIO Info In out"=w110:T18)  [unwired: 7 in]
    n17 = call <vilib>:"NavX Open.vi"("I2C Channel"=I2C_Channel."A") -> ("error out"=w94:errorcluster, "NavX Info"=w96:T23)  [unwired: 9 in]
    n18 = call "Digital Debounce Filter.vi"("Boolean input"=w107) -> ("Rising Edge"=→"Rising Edge":bool)  [unwired: 1 in, 2 out]
    n19 = call "Arduino Interfacing VI.vi"("AE Mode"=Arduino_Interfacing."Read From Arduino") -> ("error out"=w82:errorcluster, "Arduino Data"=w75:T4)  [unwired: 3 in]
    "Arduino Data" <- w75
    n20 = Unbundle By Name(w75) -> ("Rotary Switch"=→"Task selection":u8)
    n21 = call "navX reading VI.vi"("NavX Info In"=w96, "Mode"=navX_type_def."Get i2C reference", "error in (no error)"=w94) -> ("NavX Info Out"=w81:T23, "Error Out"=w80:errorcluster)  [unwired: 2 out]
    n22 = Merge Errors(w82, w94) -> (w73:errorcluster)
    "I2C Error" <- w73
    n23 = Unbundle By Name(w73) -> ("status"=w72:bool)
    n24 = Not(x=w72) -> (.not. x?=w71:bool)
    n25 = call <vilib>:"DIO Write.vi"("error in (no error)"=w91, "Input"=w71, "DIO Info In"=w92) -> ("error out"=w89:errorcluster, "DIO Info Out"=w90:T18)  [unwired: 7 in]
    n26 = call "navX reading VI.vi"("NavX Info In"=w81, "Mode"=navX_type_def."Read Values", "error in (no error)"=w80) -> ("NavX Info Out"=w79:T23, "NavX Readings"=→"NavX Readings":T3, "Error Out"=w78:errorcluster)  [unwired: 1 out]
    n27 = call "FGV Bool.vi"("Init/Read/Write State"=States_for_Action_Engine."Read") -> ("Output node"=w113:bool)  [unwired: 2 in, 1 out]
    n28 = Wait (ms)(milliseconds to wait=u32 20) -> ()  [unwired: 1 out]
  }
  n29 = call "IMAQ Create"("Image Name"="Image dest") -> ("New Image"=w22:T24, "error out"=w21:errorcluster)  [unwired: 4 in]
  n30 = while {
    tunnel: w61 -> [w131]
    tunnel: w62 -> [w130]
    tunnel: [w129] -> w68
    tunnel: [w128] -> w67
    tunnel: w66 -> [w127]
    tunnel: [w126] -> w64
    tunnel: w65 -> [w125]
    tunnel: [w124] -> w63
    stop <- w122 stop-if-true
    # "Generate USER Event Loop"
    n31 = local read "Rising Edge"() -> (w119:bool)
    n32 = Or(x="OK Button", y=w119) -> (x .or. y?=w118:bool)
    n33 = local read "TASK ENABLE"() -> (w117:bool)
    n34 = And(x=w118, y=w117) -> (x .and. y?=w116:bool)
    n35 = case shown="True" w116 {
      selector: w116 -> [_ w142]
      tunnel: w131 -> [w141 w146]
      tunnel: [w141 w145] -> w128
      tunnel: w127 -> [w140 w144]
      tunnel: [w140 w143] -> w126
      frame False {
      }
      frame True {
        n36 = Generate User Event(user event=w146, event data cluster=w142, error in=w144) -> (user event out=w145:refnum<user-event>, error out=w143:errorcluster)  [unwired: 1 in]
      }
    }
    n37 = case shown="False" "STOP" {
      selector: "STOP" -> [_ w135]
      tunnel: w130 -> [w134 w139]
      tunnel: [w134 w138] -> w129
      tunnel: w125 -> [w133 w137]
      tunnel: [w133 w136] -> w124
      tunnel: [FALSE w135] -> w122
      frame False {
      }
      frame True {
        n38 = Generate User Event(user event=w139, event data cluster=w135, error in=w137) -> (user event out=w138:refnum<user-event>, error out=w136:errorcluster)  [unwired: 1 in]
      }
    }
    n39 = Wait (ms)(milliseconds to wait=u32 50) -> ()  [unwired: 1 out]
    n40 = call "FGV Bool.vi"("Init/Read/Write State"=States_for_Action_Engine."Write", "Input Node"=w122) -> ()  [unwired: 1 in, 2 out]
  }
  n41 = while {
    tunnel: w60 -> [w153]
    tunnel: [w152] -> w59
    tunnel: w47 -> [w150]
    tunnel: [w149] -> w58
    tunnel: w53 -> [w148]
    tunnel: [w147] -> w50
    stop <- w151 stop-if-true
    # "EVENT Handling Loop"
    n42 = event shown="[1] <Start Task>: User Event" {
      selector: w153 -> [_ _ _]
      dyn-events: [_ _ _] -> w152
      timeout: _ -> [_ _ _]
      tunnel: [FALSE FALSE w183] -> w151
      tunnel: w150 -> [w158 w167 w181]
      tunnel: [w157 w166 w182] -> w149
      tunnel: w148 -> [w156 w165 w180]
      tunnel: [w155 w164 w179] -> w147
      event Timeout {
        n43 = event-data() -> ()  [unwired: 1 in, 3 out]
        n44 = Enqueue Element(queue=w158, element=Intruction_Type_Definitions."None" ("Enum"), error in (no error)=w156) -> (queue out=w157:refnum<queue>, error out=w155:errorcluster)  [unwired: 1 in, 1 out]
      }
      event User Event {
        n45 = event-data() -> ()  [unwired: 1 in, 5 out]
        n46 = call "Arduino Interfacing VI.vi"("AE Mode"=Arduino_Interfacing."Read From Arduino") -> ("Arduino Data"=w161:T4)  [unwired: 3 in, 1 out]
        n47 = Unbundle By Name(w161) -> ("Rotary Switch"=w160:u8)
        n48 = case shown="5" w160 {
          tunnel: [Intruction_Type_Definitions."None" ("Enum") Intruction_Type_Definitions."Start Task 1" ("Enum") Intruction_Type_Definitions."Start Task 2" ("Enum") Intruction_Type_Definitions."Start Task 3" ("Enum") Intruction_Type_Definitions."Start Task 4" ("Enum") Intruction_Type_Definitions."Start Task 5" ("Enum") Intruction_Type_Definitions."Start Task 6" ("Enum") Intruction_Type_Definitions."Start Task 8" ("Enum") Intruction_Type_Definitions."Start Task 9" ("Enum")] -> w163
          frame 0, Default {
          }
          frame 1 {
          }
          frame 2 {
          }
          frame 3 {
          }
          frame 4 {
          }
          frame 5 {
          }
          frame 6 {
          }
          frame 8 {
          }
          frame 9 {
          }
        }
        n49 = Enqueue Element(queue=w167, element=w163, error in (no error)=w165) -> (queue out=w166:refnum<queue>, error out=w164:errorcluster)  [unwired: 1 in, 1 out]
      }
      event User Event {
        n50 = event-data() -> ("Stop Queue"=w183:bool)  [unwired: 1 in, 4 out]
        n51 = Enqueue Element At Opposite End(queue=w181, element=Intruction_Type_Definitions."Exit" ("Enum"), error in (no error)=w180) -> (queue out=w182:refnum<queue>, error out=w179:errorcluster)  [unwired: 1 in, 1 out]
      }
    }
  }
  n52 = while {
    tunnel: w47 -> [w220]
    tunnel: w48 -> [w232]
    tunnel: w51 -> [w230]
    tunnel: [w229] -> _
    tunnel: [w228] -> w41
    shift-right: [w221] -> _
    shift-left: T16 {"PING_A"=0, "PING_B"=0, "PING_C"=0, "PING_D"=0} -> [w223]
    shift-right: [w214] -> _
    shift-left: State_Type_Definitions,_for_0.26g_versions_and_later_2."Startup" ("Enum") -> [w217]
    shift-right: [w210] -> _
    shift-left: T17 {"xDistance"=0.0, "yDistance"=0.0, "wDistance"=0.0} -> [w212]
    shift-right: [w207] -> _
    shift-left: _ -> [w206]
    tunnel: w22 -> [w205]
    tunnel: w21 -> [w204]
    shift-right: [w201] -> _
    shift-left: T15 {"Recognized Object"=FALSE, "Object X coordinate"=0.0, "Object Y coordinate"=0.0} -> [w203]
    shift-right: [w198] -> _
    shift-left: T13 {"y Stepper Position"=0, "z Stepper Position"=0} -> [w200]
    shift-right: [w195] -> _
    shift-left: T12 {"Yaw"=0.0, "Compass"=0.0} -> [w197]
    shift-right: [w192] -> _
    shift-left: T11 {"Time up flag"=FALSE, "SET TIME TO CHECK"=0.0} -> [w194]
    shift-right: [w190] -> _
    shift-left: T10 {"yStepper desired"=0} -> [w191]
    shift-right: [w186] -> _
    shift-left: T9 {"Left IR Sensor"=0.0, "Arm IR Sensor"=0.0, "Bottom IR Sensor"=0.0} -> [w188]
    shift-right: [w184] -> _
    shift-left: T8 {"ySpeed"=0.0, "xSpeed"=0.0, "wSpeed"=0.0} -> [w185]
    stop <- w219 stop-if-true
    # ">>> Motor control cluster >>>"
    # ">>> yStepper command>>>"
    # ">>True Stop Next State >>"
    # ">>Error  >>"
    # ">>Timeout>>"
    # ">>Action states Queue Reference >>"
    # ">>State Logic Queue Reference >>"
    # "TOP LEVEL BASELINE (MAIN PROCESSING LOOP)"
    n53 = Dequeue Element(queue=w232, timeout in ms (-1)=0, error in (no error)=w230) -> (queue out=w224:refnum<queue>, element=w231:string, error out=w225:errorcluster)  [unwired: 1 out]
    "Action State" <- w231
    n54 = Wait (ms)(milliseconds to wait=u32 20) -> ()  [unwired: 1 out]
    n55 = case shown="\"DISPOSE ALL BUFFERS\"" w231 {
      tunnel: [_ _ _ _ _ _ _ _ _ _ _ _ _ _ _ _ _ _ _ 0 w2149 _ _ _ _ _ _ _ _ _ _ _ _ _ _ _ _ _ _ _ _ _ _ _ _ _ _ _] -> w227
      tunnel: w224 -> [_ _ _ _ _ _ _ _ _ _ _ _ _ _ _ _ _ _ _ _ _ _ _ _ _ _ _ _ _ _ _ _ _ _ _ _ _ _ _ _ _ _ _ _ _ _ _ _]
      tunnel: w223 -> [w1907 w1916 w1928 w1939 w1956 w1967 w1978 w1990 w2003 w2015 w2026 w2033 w2048 w2062 w2074 w2082 w2094 w2119 w2129 w2140 w2150 w2159 w2169 w2199 w2210 w2218 w2227 w2240 w2253 w2263 w2272 w2289 w2298 w2313 w2320 w2330 w2340 w2350 w2357 w2369 w2385 w2391 w2403 w2415 w2427 w2439 w2451 w2462]
      tunnel: [w1907 w1916 w1928 w1939 w1956 w1967 w1978 w1990 w2003 w2015 w2026 w2033 w2048 w2063 w2074 w2082 w2094 w2120 w2129 w2140 w2150 w2159 w2169 w2198 w2210 w2218 w2227 w2240 w2253 w2263 w2272 w2289 w2298 w2313 w2320 w2330 w2340 w2350 w2357 w2369 w2385 w2391 w2403 w2415 w2427 w2439 w2451 w2462] -> w222
      tunnel: [TRUE TRUE _ _ _ _ _ _ _ _ _ _ _ _ _ _ _ _ _ _ _ _ _ _ _ _ _ _ _ _ _ _ _ _ _ _ _ _ _ _ _ _ _ _ _ _ _ _] -> w219
      tunnel: w217 -> [w1905 w1914 w1927 w1938 w1955 w1966 w1977 w1989 w2002 w2014 w2025 w2032 w2047 w2061 w2073 w2080 w2093 w2118 w2128 w2137 w2147 w2158 w2168 w2197 w2209 w2217 w2226 w2239 w2252 w2262 w2271 w2288 w2297 w2304 w2319 w2329 w2339 w2349 w2356 w2368 w2384 w2390 w2402 w2414 w2426 w2438 w2450 w2461]
      tunnel: [_ _ _ _ _ _ _ _ _ _ _ _ _ _ _ _ _ _ _ _ TRUE _ _ _ _ _ _ _ _ _ _ _ _ _ _ _ _ _ _ _ _ _ _ _ _ _ _ _] -> w216
      tunnel: [w1905 w1914 w1927 w1938 w1955 w1966 w1977 w1989 w2002 w2014 w2025 w2032 w2047 w2061 w2073 w2080 w2093 w2118 w2128 w2137 w2147 w2158 w2168 w2197 w2209 w2217 w2226 w2239 w2252 w2262 w2271 w2288 w2297 w2304 w2319 w2329 w2339 w2349 w2356 w2368 w2384 w2390 w2402 w2414 w2426 w2438 w2450 w2461] -> w215
      tunnel: w212 -> [w1904 w1913 w1926 w1941 w1954 w1965 w1976 w1988 w2001 w2013 w2024 w2034 w2046 w2060 w2075 w2084 w2095 w2117 w2130 w2136 w2146 w2160 w2170 w2187 w2208 w2220 w2228 w2241 w2254 w2264 w2273 w2290 w2300 w2311 w2322 w2332 w2342 w2352 w2359 w2371 w2387 w2393 w2405 w2417 w2429 w2441 w2453 w2464]
      tunnel: [w1904 w1913 w1926 w1941 w1954 w1965 w1976 w1988 w2001 w2013 w2024 w2034 w2045 w2060 w2075 w2084 w2095 w2116 w2130 w2136 w2146 w2160 w2170 w2186 w2208 w2220 w2228 w2241 w2254 w2264 w2273 w2290 w2300 w2311 w2322 w2332 w2342 w2352 w2359 w2371 w2387 w2393 w2405 w2417 w2429 w2441 w2453 w2464] -> w211
      tunnel: w205 -> [w1899 _ _ _ _ _ _ _ _ _ _ _ _ _ _ _ _ _ _ _ _ _ _ _ _ _ _ _ _ _ _ w2284 _ w2307 _ _ _ _ _ _ _ _ _ _ _ _ _ _]
      tunnel: w204 -> [_ _ _ _ _ _ _ _ _ _ _ _ _ _ _ _ _ _ _ _ _ _ _ _ _ _ _ _ _ w2256 _ w2286 w2296 w2306 _ _ _ _ _ _ _ _ _ _ _ _ _ _]
      tunnel: w203 -> [w1903 w1912 w1925 w1940 w1953 w1964 w1975 w1987 w2000 w2012 w2022 w2031 w2044 w2059 w2068 w2083 w2092 w2108 w2127 w2135 w2145 w2157 w2167 w2192 w2206 w2219 w2225 w2238 w2251 w2258 w2270 w2281 w2299 w2312 w2321 w2331 w2341 w2351 w2358 w2370 w2386 w2392 w2404 w2416 w2428 w2440 w2452 w2463]
      tunnel: [w1903 w1912 w1925 w1940 w1953 w1964 w1975 w1987 w2000 w2012 w2022 w2031 w2044 w2059 w2068 w2083 w2092 w2107 w2127 w2135 w2145 w2157 w2167 w2191 w2206 w2219 w2225 w2238 w2251 w2258 w2270 w2280 w2299 w2312 w2321 w2331 w2341 w2351 w2358 w2370 w2386 w2392 w2404 w2416 w2428 w2440 w2452 w2463] -> w202
      tunnel: w200 -> [w1902 w1911 w1924 w1942 w1952 w1963 w1974 w1986 w1999 w2011 w2021 w2030 w2043 w2058 w2076 w2085 w2091 w2113 w2126 w2134 w2144 w2156 w2166 w2182 w2205 w2216 w2224 w2237 w2250 w2261 w2269 w2291 w2301 w2310 w2318 w2328 w2338 w2348 w2360 w2372 w2383 w2394 w2406 w2418 w2430 w2442 w2454 w2465]
      tunnel: [w1902 w1911 w1924 w1942 w1952 w1963 w1974 w1986 w1999 w2011 w2021 w2030 w2043 w2058 w2076 w2085 w2091 w2112 w2126 w2134 w2144 w2156 w2166 w2181 w2205 w2216 w2224 w2237 w2250 w2261 w2269 w2291 w2301 w2310 w2318 w2328 w2338 w2348 w2360 w2372 w2382 w2394 w2406 w2418 w2430 w2442 w2454 w2465] -> w199
      tunnel: w197 -> [w1901 w1910 w1922 w1943 w1950 w1961 w1973 w1984 w1997 w2009 w2020 w2029 w2042 w2051 w2071 w2086 w2090 w2103 w2125 w2133 w2143 w2155 w2165 w2178 w2204 w2213 w2223 w2236 w2249 w2260 w2268 w2292 w2302 w2309 w2317 w2325 w2335 w2345 w2361 w2373 w2377 w2395 w2407 w2419 w2431 w2443 w2455 w2466]
      tunnel: [w1901 w1910 w1922 w1943 w1950 w1961 w1973 w1984 w1997 w2009 w2020 w2029 w2042 w2051 w2070 w2086 w2090 w2102 w2125 w2133 w2143 w2155 w2165 w2177 w2204 w2213 w2223 w2236 w2249 w2260 w2268 w2292 w2302 w2309 w2317 w2325 w2335 w2345 w2361 w2373 w2377 w2395 w2407 w2419 w2431 w2443 w2455 w2466] -> w196
      tunnel: w194 -> [w1898 w1909 w1923 w1944 w1951 w1962 w1972 w1985 w1998 w2010 w2019 w2028 w2041 w2050 w2067 w2087 w2089 w2099 w2122 w2132 w2142 w2154 w2164 w2175 w2202 w2212 w2222 w2235 w2248 w2259 w2267 w2293 w2303 w2308 w2316 w2324 w2334 w2344 w2362 w2374 w2376 w2389 w2401 w2413 w2425 w2437 w2449 w2460]
      tunnel: [w1898 w1909 w1923 w1944 w1951 w1962 w1972 w1985 w1998 w2010 w2019 w2028 w2041 w2050 w2067 w2087 w2089 w2099 w2122 w2132 w2142 w2154 w2164 w2174 w2202 w2212 w2222 w2235 w2248 w2259 w2267 w2293 w2303 w2308 w2316 w2324 w2334 w2344 w2362 w2374 w2376 w2389 w2399 w2411 w2423 w2435 w2447 w2459] -> w193
      tunnel: w191 -> [_ _ _ _ _ _ _ _ _ _ _ _ _ _ _ _ _ _ _ _ _ _ _ _ _ _ _ _ _ _ _ _ _ _ _ _ _ _ _ w2365 _ _ _ _ _ _ _ _]
      tunnel: [w1897 w1908 w1917 w1934 w1945 w1957 w1968 w1979 w1993 w2004 w2016 w2027 w2035 w2049 w2064 w2078 w2088 w2096 w2121 w2131 w2141 w2153 w2161 w2171 w2201 w2211 w2221 w2229 w2242 w2255 w2265 w2274 w2294 w2314 w2315 w2323 w2333 w2343 w2353 w2363 w2375 w2388 w2396 w2408 w2420 w2432 w2444 w2456] -> w187
      tunnel: w188 -> [w1897 w1908 w1917 w1934 w1945 w1957 w1968 w1979 w1993 w2004 w2016 w2027 w2035 w2049 w2064 w2079 w2088 w2096 w2121 w2131 w2141 w2153 w2161 w2171 w2201 w2211 w2221 w2229 w2242 w2255 w2265 w2274 w2294 w2314 w2315 w2323 w2333 w2343 w2353 w2363 w2375 w2388 w2396 w2408 w2420 w2432 w2444 w2456]
      tunnel: w185 -> [_ _ _ _ _ _ _ _ w1992 _ _ _ _ _ _ _ _ _ _ _ _ _ _ _ _ _ _ _ _ _ _ _ _ _ _ _ _ _ _ _ _ _ _ _ _ _ _ _]
      frame "Exit" {
        # ">>State Logic  >>"
        # ">>> Time cluster >>>"
        # ">>> Yaw >>>"
        # ">>> Stepper position >>>"
        # ">>> Encoders >>>"
        # ">>> Object detection >>>"
        # ">>> Ultrasonic Sensors Detect >>>"
        n56 = call "Imaq Dispose"("All Images? (No)"=TRUE, "Image"=w1899) -> ()  [unwired: 4 in, 1 out]
      }
      frame "----Movement States----" {
        # ">>State Logic  >>"
        # ">>> Time cluster >>>"
        # ">>> Yaw >>>"
        # ">>> Stepper position >>>"
        # ">>> Encoders >>>"
        # ">>> Object detection >>>"
        # ">>> Ultrasonic Sensors Detect >>>"
      }
      frame "FORWARD" {
        # ">>State Logic  >>"
        # ">>> Time cluster >>>"
        # ">>> Yaw >>>"
        # ">>> Stepper position >>>"
        # ">>> Encoders >>>"
        # ">>> Object detection >>>"
        # ">>> Ultrasonic Sensors Detect >>>"
        n57 = Unbundle By Name(w1922) -> ("Yaw"=w1918:dbl)
        n58 = call "MOTOR CONTROL WITH PID AE.vi"("Yaw"=w1918, "Speed"=50.0, "Direction"=MOTOR_CONTROL_WITH_PID_AE_DIRECTION_TYPE_DEF."y-axis movement", "AE Mode"=MOTOR_CONTROL_WITH_PID_AE_DATA_MODE_TYPE_DEF."Write to AE") -> ()  [unwired: 1 out]
      }
      frame "FORWARD - IR ASSIST" {
        # ">>State Logic  >>"
        # ">>> Time cluster >>>"
        # ">>> Yaw >>>"
        # ">>> Stepper position >>>"
        # ">>> Encoders >>>"
        # ">>> Object detection >>>"
        # ">>> Ultrasonic Sensors Detect >>>"
        n59 = Unbundle By Name(w1934) -> ("Left IR Sensor"=w1933:dbl)
        n60 = Subtract(x=w1933, y=15.0) -> (x-y=w1931:dbl)
        n61 = Multiply(x=w1931, y=0.5) -> (x*y=w1929:dbl)
        n62 = call "MOTOR CONTROL WITH PID AE.vi"("Yaw"=w1929, "Speed"=30.0, "Direction"=MOTOR_CONTROL_WITH_PID_AE_DIRECTION_TYPE_DEF."y-axis movement", "AE Mode"=MOTOR_CONTROL_WITH_PID_AE_DATA_MODE_TYPE_DEF."Write to AE") -> ()  [unwired: 1 out]
      }
      frame "LEFT" {
        # ">>State Logic  >>"
        # ">>> Time cluster >>>"
        # ">>> Yaw >>>"
        # ">>> Stepper position >>>"
        # ">>> Encoders >>>"
        # ">>> Object detection >>>"
        # ">>> Ultrasonic Sensors Detect >>>"
        n63 = Unbundle By Name(w1950) -> ("Yaw"=w1947:dbl)
        n64 = call "MOTOR CONTROL WITH PID AE.vi"("Yaw"=w1947, "Speed"=-25.0, "Direction"=MOTOR_CONTROL_WITH_PID_AE_DIRECTION_TYPE_DEF."x-axis movement", "AE Mode"=MOTOR_CONTROL_WITH_PID_AE_DATA_MODE_TYPE_DEF."Write to AE") -> ()  [unwired: 1 out]
      }
      frame "R-ACW" {
        # ">>> IR Sensors >>>"
        # ">>> Time cluster >>>"
        # ">>> Yaw >>>"
        # ">>> Stepper position >>>"
        # ">>> Encoders >>>"
        # ">>> Object detection >>>"
        # ">>> Ultrasonic Sensors Detect >>>"
        n65 = call "MOTOR CONTROL WITH PID AE.vi"("Speed"=-10.0, "Direction"=MOTOR_CONTROL_WITH_PID_AE_DIRECTION_TYPE_DEF."rotation", "AE Mode"=MOTOR_CONTROL_WITH_PID_AE_DATA_MODE_TYPE_DEF."Write to AE") -> ()  [unwired: 1 in, 1 out]
      }
      frame "R-CW" {
        (unwired) -0.2 ("Speed")
        # ">>> Time cluster >>>"
        # ">>> Yaw >>>"
        # ">>> Stepper position >>>"
        # ">>> Encoders >>>"
        # ">>> Object detection >>>"
        # ">>> Ultrasonic Sensors Detect >>>"
        n66 = call "MOTOR CONTROL WITH PID AE.vi"("Speed"=10.0, "Direction"=MOTOR_CONTROL_WITH_PID_AE_DIRECTION_TYPE_DEF."rotation", "AE Mode"=MOTOR_CONTROL_WITH_PID_AE_DATA_MODE_TYPE_DEF."Write to AE") -> ()  [unwired: 1 in, 1 out]
      }
      frame "RIGHT" {
        # ">>> Time cluster >>>"
        # ">>> Yaw >>>"
        # ">>> Stepper position >>>"
        # ">>> Encoders >>>"
        # ">>> Object detection >>>"
        # ">>> Ultrasonic Sensors Detect >>>"
        n67 = Unbundle By Name(w1984) -> ("Yaw"=w1980:dbl)
        n68 = call "MOTOR CONTROL WITH PID AE.vi"("Yaw"=w1980, "Speed"=50.0, "Direction"=MOTOR_CONTROL_WITH_PID_AE_DIRECTION_TYPE_DEF."x-axis movement", "AE Mode"=MOTOR_CONTROL_WITH_PID_AE_DATA_MODE_TYPE_DEF."Write to AE") -> ()  [unwired: 1 out]
      }
      frame "X AXIS - SLOW" {
        # ">>> IR Sensors >>>"
        # ">>> Time cluster >>>"
        # ">>> Yaw >>>"
        # ">>> Stepper position >>>"
        # ">>> Encoders >>>"
        # ">>> Object detection >>>"
        # ">>> Ultrasonic Sensors Detect >>>"
        n69 = Unbundle By Name(w1992) -> ("xSpeed"=w1991:dbl)
        n70 = Unbundle By Name(w1997) -> ("Yaw"=w1994:dbl)
        n71 = call "MOTOR CONTROL WITH PID AE.vi"("Yaw"=w1994, "Speed"=w1991, "Direction"=MOTOR_CONTROL_WITH_PID_AE_DIRECTION_TYPE_DEF."x-axis movement", "AE Mode"=MOTOR_CONTROL_WITH_PID_AE_DATA_MODE_TYPE_DEF."Write to AE") -> ()  [unwired: 1 out]
      }
      frame "REVERSE" {
        # ">>> Time cluster >>>"
        # ">>> Yaw >>>"
        # ">>> Stepper position >>>"
        # ">>> Encoders >>>"
        # ">>> Object detection >>>"
        # ">>> Ultrasonic Sensors Detect >>>"
        n72 = Unbundle By Name(w2009) -> ("Yaw"=w2005:dbl)
        n73 = call "MOTOR CONTROL WITH PID AE.vi"("Yaw"=w2005, "Speed"=-50.0, "Direction"=MOTOR_CONTROL_WITH_PID_AE_DIRECTION_TYPE_DEF."y-axis movement", "AE Mode"=MOTOR_CONTROL_WITH_PID_AE_DATA_MODE_TYPE_DEF."Write to AE") -> ()  [unwired: 1 out]
      }
      frame "STOP" {
        n74 = Wait (ms)(milliseconds to wait=u32 100) -> ()  [unwired: 1 out]
        n75 = call "MOTOR CONTROL WITH PID AE.vi"("Direction"=MOTOR_CONTROL_WITH_PID_AE_DIRECTION_TYPE_DEF."stop", "AE Mode"=MOTOR_CONTROL_WITH_PID_AE_DATA_MODE_TYPE_DEF."Write to AE") -> ()  [unwired: 2 in, 1 out]
      }
      frame "----SENSOR READING---- " {
      }
      frame "READ ENCODERS" {
        # ">>> Time cluster >>>"
        # ">>> Yaw >>>"
        # ">>> Stepper position >>>"
        # ">>> Object detection >>>"
        # ">>> Current encoder distance >>>"
        # ">>> Ultrasonic Sensors Detect >>>"
        n76 = call "MOTOR CONTROL WITH PID AE.vi"("AE Mode"=MOTOR_CONTROL_WITH_PID_AE_DATA_MODE_TYPE_DEF."Read from AE") -> ("Speed & distance"=w2039:T1)  [unwired: 3 in]
        n77 = Unbundle By Name(w2039) -> ("xDistance"=w2038:dbl, "yDistance"=w2037:dbl, "wDistance"=w2036:dbl)
        n78 = Bundle By Name(cluster=w2046, "xDistance"=w2038, "yDistance"=w2037, "wDistance"=w2036) -> (w2045:T17)
      }
      frame "READ ULTRASONIC" {
        (unwired) navX_type_def."Read Values" ("Mode")
        (unwired) MOTOR_CONTROL_NO_PID_Type_Def."Latch" ("Direction")
        # ">>State Logic  >>"
        # ">>> Time cluster >>>"
        # ">>> Ultrasonic Sensors Detect >>>"
        # ">>> Object detection >>>"
        # ">>> Encoders >>>"
        # ">>> Stepper position >>>"
        # ">>> Yaw >>>"
        n79 = call "Arduino Interfacing VI.vi"("AE Mode"=Arduino_Interfacing."Read From Arduino") -> ("Arduino Data"=w2056:T4)  [unwired: 3 in, 1 out]
        n80 = Unbundle By Name(w2056) -> ("PING A"=w2055:u8, "PING B"=w2054:u8, "PING C"=w2053:u8, "PING D"=w2052:u8)
        n81 = Bundle By Name(cluster=w2062, "PING_A"=w2055, "PING_B"=w2054, "PING_C"=w2053, "PING_D"=w2052) -> (w2063:T16)
      }
      frame "READ NAVX" {
        # ">>> Time cluster >>>"
        # ">>> Yaw >>>"
        # ">>> Ultrasonic Sensors Detect >>>"
        # ">>> Object detection >>>"
        # ">>> Encoders >>>"
        # ">>> Stepper position >>>"
        n82 = call "navX reading VI.vi"("Mode"=navX_type_def."Read Values") -> ("NavX Readings"=w2066:T3)  [unwired: 2 in, 3 out]
        n83 = Unbundle By Name(w2066) -> ("Heading"=w2065:dbl)
        n84 = Unbundle By Name(w2066) -> ("Yaw"=w2069:dbl)
        n85 = Bundle By Name(cluster=w2071, "Yaw"=w2069, "Compass"=w2065) -> (w2070:T12)
      }
      frame "READ IR" {
        w2081 = T35 [enum."A/AI0"] items=["Not Connected", "AudioIn/Left", "AudioIn/Right", "C/AI0", "C/AI1", "A/AI0", "A/AI1", "A/AI2", "A/AI3", "A/AI4", "A/AI5", "A/AI6", "A/AI7", "B/AI0", "B/AI1", "B/AI2", "B/AI3", "B/AI4", "B/AI5", "B/AI6", "B/AI7", "AI/AI0", "AI/AI1", "AI/AI2", "AI/AI3", "A/AI0 (DIFF)", "A/AI1 (DIFF)", "A/AI2 (DIFF)", "A/AI3 (DIFF)", "B/AI0 (DIFF)", "B/AI1 (DIFF)", "B/AI2 (DIFF)", "B/AI3 (DIFF)"] ("AI Channel")
        # ">>State Logic  >>"
        # ">>> Time cluster >>>"
        # ">>> Ultrasonic Sensors Detect >>>"
        # ">>> Object detection >>>"
        # ">>> Encoders >>>"
        # ">>> Stepper position >>>"
        # ">>> Yaw >>>"
        n86 = call <vilib>:"Sharp IR.vi"("AI Channel"=w2081) -> ("Sharp IR Distance"=w2077:dbl)  [unwired: 8 in, 2 out]
        n87 = Bundle By Name(cluster=w2079, "Left IR Sensor"=w2077) -> (w2078:T9)
      }
      frame "----SYSTEM MODES----" {
        (unwired) I2C_MASTER_Type_Def."Last State" ("Arduino Mode")
        # ">>> Object detection >>>"
        # ">>> Yaw >>>"
        # ">>> Ultrasonic Sensors Detect >>>"
        # ">>> Encoders >>>"
        # ">>> Stepper position >>>"
      }
      frame "INIT" {
        w2114 = u8 0
        w2115 = 0.0
        # ">>> Time cluster >>>"
        # ">>> Object detection >>>"
        # ">>> Yaw >>>"
        # ">>> Ultrasonic Sensors Detect >>>"
        # ">>> Encoders >>>"
        # ">>> Stepper position >>>"
        # ">>State Logic  >>"
        n88 = call "Arduino Interfacing VI.vi"("AE Mode"=Arduino_Interfacing."Initialize") -> ()  [unwired: 3 in, 2 out]
        n89 = call "FGV Bool.vi"("Init/Read/Write State"=States_for_Action_Engine."Initialize") -> ()  [unwired: 2 in, 2 out]
        n90 = call "Elasped Timer.vi"("Action"=Elapsed_timer_control."Initialize") -> ()  [unwired: 7 in, 4 out]
        n91 = call "MOTOR CONTROL WITH PID AE.vi"("AE Mode"=MOTOR_CONTROL_WITH_PID_AE_DATA_MODE_TYPE_DEF."Init AE") -> ()  [unwired: 3 in, 1 out]
        n92 = Bundle By Name(cluster=w2108, "Recognized Object"=FALSE, "Object X coordinate"=0.0, "Object Y coordinate"=0.0) -> (w2107:T15)
        n93 = Bundle By Name(cluster=w2113, "y Stepper Position"=u8 0, "z Stepper Position"=u8 0) -> (w2112:T13)
        n94 = Bundle By Name(cluster=w2117, "xDistance"=w2115, "yDistance"=w2115, "wDistance"=w2115) -> (w2116:T17)
        n95 = Bundle By Name(cluster=w2119, "PING_A"=w2114, "PING_B"=w2114, "PING_C"=w2114, "PING_D"=w2114) -> (w2120:T16)
        n96 = Bundle By Name(cluster=w2103, "Yaw"=0.0) -> (w2102:T12)
      }
      frame "ARDUINO - ULTRASONIC" {
        # ">>> Object detection >>>"
        # ">>> Yaw >>>"
        # ">>> Ultrasonic Sensors Detect >>>"
        # ">>> Encoders >>>"
        # ">>> Stepper position >>>"
        # ">>State Logic  >>"
        n97 = call "Arduino Interfacing VI.vi"("Data to Write"=I2C_MASTER_WRITE_NEW_Type_Def."Ultrasonic sensors", "AE Mode"=Arduino_Interfacing."Write to Arduino") -> ()  [unwired: 2 in, 2 out]
      }
      frame "NAVX CALIBRATE" {
        # ">>> Object detection >>>"
        # ">>> Yaw >>>"
        # ">>> Ultrasonic Sensors Detect >>>"
        # ">>> Encoders >>>"
        # ">>> Stepper position >>>"
        # ">>State Logic  >>"
        # "Adds a 15 second delay to the startup process \nfor the NavX to calibrate"
        n98 = Wait (ms)(milliseconds to wait=u32 1000) -> ()  [unwired: 1 out]
      }
      frame "NO ACTION", Default {
        (unwired) u8 0 ("y Stepper value")
        (unwired) TRUE ("Latch")
        (unwired) navX_type_def."Read Values" ("Mode")
        (unwired) MOTOR_CONTROL_NO_PID_Type_Def."Latch" ("Direction")
        # ">>> Object detection >>>"
        # ">>> Yaw >>>"
        # ">>> Ultrasonic Sensors Detect >>>"
        # ">>> Encoders >>>"
        # ">>> Stepper position >>>"
        # ">>State Logic  >>"
        n99 = case shown="4" w2147 {
          tunnel: [0 100] -> w2149
          frame 1, Default {
          }
          frame 4 {
          }
        }
      }
      frame "----RESET CASES----" {
        (unwired) I2C_MASTER_Type_Def."Last State" ("Arduino Mode")
        # ">>> Object detection >>>"
        # ">>> Yaw >>>"
        # ">>> Ultrasonic Sensors Detect >>>"
        # ">>> Encoders >>>"
        # ">>> Stepper position >>>"
        # ">>State Logic  >>"
      }
      frame "RESET ENCODERS" {
        # ">>> Object detection >>>"
        # ">>> Yaw >>>"
        # ">>> Ultrasonic Sensors Detect >>>"
        # ">>> Encoders >>>"
        # ">>> Stepper position >>>"
        # ">>State Logic  >>"
        n100 = call "MOTOR CONTROL WITH PID AE.vi"("Direction"=MOTOR_CONTROL_WITH_PID_AE_DIRECTION_TYPE_DEF."reset encoders", "AE Mode"=MOTOR_CONTROL_WITH_PID_AE_DATA_MODE_TYPE_DEF."Write to AE") -> ()  [unwired: 2 in, 1 out]
      }
      frame "RESET FLAGS" {
        (unwired) I2C_MASTER_Type_Def."Last State" ("Arduino Mode")
        # "Resets any software variables\nand/or non-critical states"
        n101 = Wait (ms)(milliseconds to wait=u32 20) -> ()  [unwired: 1 out]
        n102 = Bundle By Name(cluster=w2175, "Time up flag"=FALSE, "SET TIME TO CHECK"=0.0) -> (w2174:T11)
        n103 = Bundle By Name(cluster=w2192, "Recognized Object"=FALSE, "Object X coordinate"=0.0, "Object Y coordinate"=0.0) -> (w2191:T15)
        n104 = Bundle By Name(cluster=w2182, "y Stepper Position"=u8 0, "z Stepper Position"=u8 0) -> (w2181:T13)
        n105 = Bundle By Name(cluster=w2187, "xDistance"=0.0, "yDistance"=0.0, "wDistance"=0.0) -> (w2186:T17)
        n106 = Bundle By Name(cluster=w2199, "PING_A"=u8 0, "PING_B"=u8 0, "PING_C"=u8 0, "PING_D"=u8 0) -> (w2198:T16)
        n107 = Bundle By Name(cluster=w2178, "Yaw"=0.0) -> (w2177:T12)
      }
      frame "RESET YAW" {
        n108 = Wait (ms)(milliseconds to wait=u32 100) -> ()  [unwired: 1 out]
        n109 = call "navX reading VI.vi"("Mode"=navX_type_def."Zero Yaw") -> ()  [unwired: 2 in, 4 out]
      }
      frame "RESET ARM" {
        n110 = call "Arduino Interfacing VI.vi"("Data to Write"=I2C_MASTER_WRITE_NEW_Type_Def."Soft Reset", "AE Mode"=Arduino_Interfacing."Write to Arduino") -> ()  [unwired: 2 in, 2 out]
      }
      frame "--------CAM STATES-------" {
      }
      frame "OPEN LOG CAM" {
        n111 = call "Webcam AE.vi"("Session In"=T32 "cam0", "Camera states"=Webcam_AE."Initialize Camera") -> ("error out"=w2232:errorcluster, "Session Out"=w2231:T32)  [unwired: 1 in, 1 out]
        n112 = call "Webcam AE.vi"("error in (no error)"=w2232, "Session In"=w2231, "Camera states"=Webcam_AE."Open Camera") -> ()  [unwired: 3 out]
      }
      frame "OPEN LIFE CAM" {
        n113 = call "Webcam AE.vi"("Session In"=T32 "cam1", "Camera states"=Webcam_AE."Initialize Camera") -> ("error out"=w2245:errorcluster, "Session Out"=w2244:T32)  [unwired: 1 in, 1 out]
        n114 = call "Webcam AE.vi"("error in (no error)"=w2245, "Session In"=w2244, "Camera states"=Webcam_AE."Open Camera") -> ()  [unwired: 3 out]
      }
      frame "CAM ACQ" {
        # ">>State Logic  >>"
        # ">>> Time cluster >>>"
        # ">>> Yaw >>>"
        # ">>> Stepper position >>>"
        # ">>> Encoders >>>"
        # ">>> Object detection >>>"
        # ">>> Ultrasonic Sensors Detect >>>"
        n115 = call "Webcam AE.vi"("error in (no error)"=w2256, "Camera states"=Webcam_AE."Continuous Acquisition") -> ()  [unwired: 1 in, 3 out]
      }
      frame "CAM CLOSE" {
        # ">>State Logic  >>"
        # ">>> Time cluster >>>"
        # ">>> Yaw >>>"
        # ">>> Stepper position >>>"
        # ">>> Encoders >>>"
        # ">>> Object detection >>>"
        # ">>> Ultrasonic Sensors Detect >>>"
        n116 = call "Webcam AE.vi"("Camera states"=Webcam_AE."Close Camera") -> ()  [unwired: 2 in, 3 out]
      }
      frame "PROCESS IMAGE" {
        # ">>State Logic  >>"
        # ">>> Time cluster >>>"
        # ">>> Yaw >>>"
        # ">>> Stepper position >>>"
        # ">>> Encoders >>>"
        # ">>> Object detection >>>"
        # ">>> Ultrasonic Sensors Detect >>>"
        n117 = call "Webcam AE.vi"("error in (no error)"=w2286, "Camera states"=Webcam_AE."Retrieve Image") -> ("error out"=w2282:errorcluster, "Image Out"=w2285:T24)  [unwired: 1 in, 1 out]
        n118 = call "Object Detection SubVI.vi"("Error In"=w2282, "Mode"="Object recognition mode", "Image Dest"=w2284, "Image in"=w2285) -> ("Object Center Coordinates"=w2279:cluster{"x":sgl, "y":sgl}, "Object detection cluster"=w2275:T2)  [unwired: 2 out]
        "Object detection cluster" <- w2275
        "Object Center Coordinates" <- w2279
        n119 = Unbundle By Name(w2275) -> ("Object detected?"=w2276:bool)
        n120 = Unbundle By Name(w2279) -> ("x"=w2278:sgl, "y"=w2277:sgl)
        n121 = Bundle By Name(cluster=w2281, "Recognized Object"=w2276, "Object X coordinate"=w2278, "Object Y coordinate"=w2277) -> (w2280:T15)
      }
      frame "DISPOSE BUFFERS" {
        # ">>State Logic  >>"
        # ">>> Time cluster >>>"
        # ">>> Yaw >>>"
        # ">>> Stepper position >>>"
        # ">>> Encoders >>>"
        # ">>> Object detection >>>"
        # ">>> Ultrasonic Sensors Detect >>>"
        n122 = call "Webcam AE.vi"("error in (no error)"=w2296, "Camera states"=Webcam_AE."Dispose Image Buffers") -> ()  [unwired: 1 in, 3 out]
      }
      frame "DISPOSE ALL BUFFERS" {
        # ">>State Logic  >>"
        # ">>> IR Sensors >>>"
        # ">>> Time cluster >>>"
        # ">>> Object detection >>>"
        # ">>> Yaw >>>"
        # ">>> Ultrasonic Sensors Detect >>>"
        # ">>> Encoders >>>"
        # ">>> Stepper position >>>"
        n123 = call "Imaq Dispose"("All Images? (No)"=TRUE, "Image"=w2307, "error in (no error)"=w2306) -> ()  [unwired: 3 in, 1 out]
      }
      frame "-----ARM ACTIONS-----" {
      }
      frame "CLOSE CLAW" {
        n124 = call "Arduino Interfacing VI.vi"("Data to Write"=I2C_MASTER_WRITE_NEW_Type_Def."Close Claw", "AE Mode"=Arduino_Interfacing."Write to Arduino") -> ()  [unwired: 2 in, 2 out]
      }
      frame "OPEN CLAW" {
        n125 = call "Arduino Interfacing VI.vi"("Data to Write"=I2C_MASTER_WRITE_NEW_Type_Def."Open Claw", "AE Mode"=Arduino_Interfacing."Write to Arduino") -> ()  [unwired: 2 in, 2 out]
      }
      frame "Z STEPPER CAM HEIGHT" {
        n126 = call "Arduino Interfacing VI.vi"("Data to Write"=I2C_MASTER_WRITE_NEW_Type_Def."zStepper 6k", "AE Mode"=Arduino_Interfacing."Write to Arduino") -> ()  [unwired: 2 in, 2 out]
      }
      frame "Z STEPPER GRAB HEIGHT" {
        # ">>State Logic  >>"
        # ">>> Time cluster >>>"
        # ">>> Yaw >>>"
        # ">>> Stepper position >>>"
        # ">>> Encoders >>>"
        # ">>> Object detection >>>"
        # ">>> Ultrasonic Sensors Detect >>>"
        n127 = call "Arduino Interfacing VI.vi"("Data to Write"=I2C_MASTER_WRITE_NEW_Type_Def."zStepper 100", "AE Mode"=Arduino_Interfacing."Write to Arduino") -> ()  [unwired: 2 in, 2 out]
      }
      frame "Y STEPPER CONTROL" {
        # ">>State Logic  >>"
        # ">>> yStepper command>>>"
        # ">>> Time cluster >>>"
        # ">>> Yaw >>>"
        # ">>> Stepper position >>>"
        # ">>> Encoders >>>"
        # ">>> Object detection >>>"
        # ">>> Ultrasonic Sensors Detect >>>"
        n128 = Unbundle By Name(w2365) -> ("yStepper desired"=w2364:u8)
        n129 = call "Arduino Interfacing VI.vi"("y Stepper value"=w2364, "Data to Write"=I2C_MASTER_WRITE_NEW_Type_Def."yStepper control", "AE Mode"=Arduino_Interfacing."Write to Arduino") -> ()  [unwired: 1 in, 2 out]
      }
      frame "READ STEPPER VALUES" {
        # ">>State Logic  >>"
        # ">>> Time cluster >>>"
        # ">>> Yaw >>>"
        # ">>> Stepper position >>>"
        # ">>> Encoders >>>"
        # ">>> Object detection >>>"
        # ">>> Ultrasonic Sensors Detect >>>"
        n130 = call "Arduino Interfacing VI.vi"("AE Mode"=Arduino_Interfacing."Read From Arduino") -> ("Arduino Data"=w2380:T4)  [unwired: 3 in, 1 out]
        n131 = Unbundle By Name(w2380) -> ("y Stepper Position"=w2379:u8, "z Stepper Position"=w2378:u8)
        n132 = Bundle By Name(cluster=w2383, "y Stepper Position"=w2379, "z Stepper Position"=w2378) -> (w2382:T13)
      }
      frame " -----TIMING-----" {
        # ">>State Logic  >>"
        # ">>> Time cluster >>>"
        # ">>> Yaw >>>"
        # ">>> Stepper position >>>"
        # ">>> Encoders >>>"
        # ">>> Object detection >>>"
        # ">>> Ultrasonic Sensors Detect >>>"
      }
      frame "SET TIMER 1" {
        # ">>State Logic  >>"
        # ">>> Time cluster >>>"
        # ">>> Yaw >>>"
        # ">>> Stepper position >>>"
        # ">>> Encoders >>>"
        # ">>> Object detection >>>"
        # ">>> Ultrasonic Sensors Detect >>>"
        n133 = call "Elasped Timer.vi"("Time Setting"=1.0, "Action"=Elapsed_timer_control."Initialize") -> ()  [unwired: 6 in, 4 out]
        n134 = Bundle By Name(cluster=w2401, "Time up flag"=FALSE) -> (w2399:T11)
      }
      frame "SET TIMER 2" {
        # ">>State Logic  >>"
        # ">>> Time cluster >>>"
        # ">>> Yaw >>>"
        # ">>> Stepper position >>>"
        # ">>> Encoders >>>"
        # ">>> Object detection >>>"
        # ">>> Ultrasonic Sensors Detect >>>"
        n135 = call "Elasped Timer.vi"("Time Setting"=2.0, "Action"=Elapsed_timer_control."Initialize") -> ()  [unwired: 6 in, 4 out]
        n136 = Bundle By Name(cluster=w2413, "Time up flag"=FALSE) -> (w2411:T11)
      }
      frame "SET TIMER 3" {
        # ">>State Logic  >>"
        # ">>> Time cluster >>>"
        # ">>> Yaw >>>"
        # ">>> Stepper position >>>"
        # ">>> Encoders >>>"
        # ">>> Object detection >>>"
        # ">>> Ultrasonic Sensors Detect >>>"
        n137 = call "Elasped Timer.vi"("Time Setting"=3.0, "Action"=Elapsed_timer_control."Initialize") -> ()  [unwired: 6 in, 4 out]
        n138 = Bundle By Name(cluster=w2425, "Time up flag"=FALSE) -> (w2423:T11)
      }
      frame "SET TIMER 4" {
        # ">>State Logic  >>"
        # ">>> Time cluster >>>"
        # ">>> Yaw >>>"
        # ">>> Stepper position >>>"
        # ">>> Encoders >>>"
        # ">>> Object detection >>>"
        # ">>> Ultrasonic Sensors Detect >>>"
        n139 = call "Elasped Timer.vi"("Time Setting"=4.0, "Action"=Elapsed_timer_control."Initialize") -> ()  [unwired: 6 in, 4 out]
        n140 = Bundle By Name(cluster=w2437, "Time up flag"=FALSE) -> (w2435:T11)
      }
      frame "SET TIMER 5" {
        # ">>State Logic  >>"
        # ">>> Time cluster >>>"
        # ">>> Yaw >>>"
        # ">>> Stepper position >>>"
        # ">>> Encoders >>>"
        # ">>> Object detection >>>"
        # ">>> Ultrasonic Sensors Detect >>>"
        n141 = call "Elasped Timer.vi"("Time Setting"=5.0, "Action"=Elapsed_timer_control."Initialize") -> ()  [unwired: 6 in, 4 out]
        n142 = Bundle By Name(cluster=w2449, "Time up flag"=FALSE) -> (w2447:T11)
      }
      frame "START TIMER" {
        # ">>State Logic  >>"
        # ">>> Time cluster >>>"
        # ">>> Yaw >>>"
        # ">>> Stepper position >>>"
        # ">>> Encoders >>>"
        # ">>> Object detection >>>"
        # ">>> Ultrasonic Sensors Detect >>>"
        n143 = call "Elasped Timer.vi"("Action"=Elapsed_timer_control."Start") -> ("Time Out?!"=w2457:bool)  [unwired: 7 in, 3 out]
        n144 = Bundle By Name(cluster=w2460, "Time up flag"=w2457) -> (w2459:T11)
      }
    }
    "State Logic" <- w215
    n145 = local read "TASK ENABLE"() -> (w209:bool)
    n146 = Not(x=w209) -> (.not. x?=w208:bool)
    n147 = case shown="True" w216 {
      tunnel: w220 -> [w245 w280]
      tunnel: w224 -> [w241 w282]
      tunnel: [w245 w280] -> w229
      tunnel: [w241 w283] -> w228
      tunnel: w225 -> [_ w278]
      tunnel: w227 -> [_ w279]
      tunnel: w222 -> [w244 w285]
      tunnel: [w244 w285] -> w221
      tunnel: "STOP TASK" -> [_ w268]
      tunnel: w215 -> [w243 w284]
      tunnel: [w243 w281] -> w214
      tunnel: w211 -> [w242 w274]
      tunnel: [w242 w274] -> w210
      tunnel: w208 -> [_ w269]
      tunnel: [w240 w266] -> w207
      tunnel: w206 -> [w240 w265]
      tunnel: w202 -> [w239 w262]
      tunnel: [w239 w262] -> w201
      tunnel: w199 -> [w238 w258]
      tunnel: [w238 w258] -> w198
      tunnel: w196 -> [w237 w256]
      tunnel: [w237 w256] -> w195
      tunnel: w193 -> [w236 w254]
      tunnel: [w236 w254] -> w192
      tunnel: w191 -> [w235 w253]
      tunnel: [w235 w252] -> w190
      tunnel: [_ w250] -> w189
      tunnel: w187 -> [w234 w248]
      tunnel: [w234 w248] -> w186
      tunnel: w185 -> [w233 w247]
      tunnel: [w233 w246] -> w184
      frame False {
        # ">>> Motor control cluster >>>"
        # ">>> yStepper command>>>"
        # ">>> Motor control cluster >>>"
        # ">>> yStepper command>>>"
        # ">>> Motor control cluster >>>"
        # ">>> IR Sensors >>>"
        # ">>> IR Sensors >>>"
        # ">>> yStepper command>>>"
        # ">>> Time cluster >>>"
        # ">>> Yaw >>>"
        # ">>> Stepper position >>>"
        # ">>> Encoders >>>"
        # ">>> Object detection >>>"
        # ">>> Ultrasonic Sensors Detect >>>"
        # ">>> Time cluster >>>"
        # ">>> Yaw >>>"
        # ">>> Stepper position >>>"
        # ">>> Encoders >>>"
        # ">>> Object detection >>>"
        # ">>> Ultrasonic Sensors Detect >>>"
      }
      frame True {
        # ">>> Motor control cluster >>>"
        # ">>> yStepper command>>>"
        # ">>> IR Sensors >>>"
        # ">>> Motor control cluster >>>"
        # ">>State Logic Queue Reference >>"
        # ">>Timeout>>"
        # ">>> yStepper command>>>"
        # ">>> Time cluster >>>"
        # ">>> Object detection >>>"
        # ">>> Yaw >>>"
        # ">>> Ultrasonic Sensors Detect >>>"
        # ">>> Encoders >>>"
        # ">>> Stepper position >>>"
        # ">>State Logic  >>"
        # ">>True Stop Next State >>"
        # ">>Action Queue>>"
        # ">> Manual override >>"
        # ">>> Time cluster >>>"
        # ">>> Yaw >>>"
        # ">>> Stepper position >>>"
        # ">>> Encoders >>>"
        # ">>> Object detection >>>"
        # ">>> Ultrasonic Sensors Detect >>>"
        # ">>Action Queue>>"
        # ">>State Logic Queue Reference >>"
        n148 = Or(x=w268, y=w269) -> (x .or. y?=w267:bool)
        n149 = Unbundle By Name(w248) -> ("Left IR Sensor"=w249:dbl)
        "Left IR Sensor" <- w249
        n150 = Unbundle By Name(w254) -> ("Time up flag"=w255:bool)
        "Time up flag" <- w255
        n151 = Unbundle By Name(w256) -> ("Yaw"=w257:dbl, "Compass"=w251:dbl)
        n152 = Unbundle By Name(w258) -> ("y Stepper Position"=w260:u8, "z Stepper Position"=w259:u8)
        n153 = Unbundle By Name(w274) -> ("xDistance"=w271:dbl, "yDistance"=w272:dbl, "wDistance"=w273:dbl)
        n154 = Unbundle By Name(w262) -> ("Recognized Object"=w261:bool, "Object X coordinate"=w264:dbl, "Object Y coordinate"=w263:dbl)
        n155 = Unbundle By Name(w285) -> ("PING_A"=w277:u8, "PING_B"=w276:u8, "PING_C"=w275:u8, "PING_D"=w270:u8)
        n156 = case shown="34" w284 {
          tunnel: [w289 w300 w313 w323 w398 w412 w448 w501 w543 w590 w633 w687 w734 w774 w834 w879 w919 w967 w1009 w1061 w1098 w1149 w1192 w1235 w1264 w1271 w1319 w1360 w1411 w1456 w1496 w1544 w1596 w1634 w1682 w1724 w1776 w1813 w1864] -> w283
          tunnel: w282 -> [w289 w303 w314 w326 w400 w413 w457 w499 w547 w591 w639 w680 w737 w781 w824 w882 w925 w966 w1012 w1051 w1104 w1139 w1187 w1226 w1264 w1275 w1326 w1365 w1401 w1459 w1502 w1543 w1595 w1640 w1681 w1727 w1766 w1819 w1854]
          tunnel: [State_Type_Definitions,_for_0.26g_versions_and_later_2."Idle" ("Enum") State_Type_Definitions,_for_0.26g_versions_and_later_2."Idle" ("Enum") w309 w325 State_Type_Definitions,_for_0.26g_versions_and_later_2."Shutdown" ("Enum") w414 w455 w502 w544 w589 w634 w686 w735 w776 w833 w880 w926 w968 w1011 w1060 w1105 w1148 w1193 w1227 State_Type_Definitions,_for_0.26g_versions_and_later_2."Idle" ("Enum") w1272 w1320 w1361 w1410 w1457 w1503 w1545 w1597 w1641 w1683 w1726 w1775 w1820 w1863] -> w281
          tunnel: w280 -> [_ _ w312 w329 _ w419 w451 w498 w548 w598 w638 w684 w738 w780 w831 w877 w924 w964 w1013 w1058 w1103 w1146 w1190 w1234 _ w1279 w1325 w1368 w1408 w1454 w1501 w1541 w1593 w1639 w1679 w1728 w1773 w1818 w1861]
          tunnel: w279 -> [_ _ _ w328 _ w418 w450 w497 w549 w597 w637 w683 w731 w779 w830 w876 w923 w963 w1014 w1057 w1102 w1145 w1189 w1232 _ w1274 w1324 w1367 w1407 w1453 w1500 w1540 w1592 w1638 w1678 w1729 w1772 w1817 w1860]
          tunnel: w278 -> [_ _ w311 w324 _ w417 w449 w496 w550 w596 w636 w682 w730 w778 w832 w878 w922 w962 w1015 w1059 w1101 w1147 w1188 w1233 _ w1278 w1323 w1366 w1409 w1455 w1499 w1539 w1591 w1637 w1677 w1730 w1774 w1816 w1862]
          tunnel: w267 -> [_ _ _ _ _ w411 w456 w495 w551 w593 w632 w685 w736 w782 w825 w883 w920 w965 w1016 w1052 w1099 w1140 w1191 w1230 _ w1277 w1318 w1364 w1402 w1460 w1497 w1542 w1594 w1635 w1680 w1731 w1767 w1814 w1855]
          tunnel: w277 -> [_ _ _ _ _ _ _ _ _ _ _ _ _ _ _ _ _ _ _ _ _ _ _ _ _ _ _ _ _ _ _ _ _ _ _ _ _ _ _]
          tunnel: w276 -> [_ _ _ _ _ _ _ w494 _ _ _ w676 w719 w772 _ w869 _ _ _ _ _ _ _ _ _ _ _ _ _ w1446 _ _ _ _ _ _ _ _ _]
          tunnel: w275 -> [_ _ _ _ _ _ _ w493 _ _ _ w677 w720 w773 _ w870 _ _ _ _ _ _ _ _ _ _ _ _ _ w1447 _ _ _ _ _ _ _ _ _]
          tunnel: w273 -> [_ _ _ _ _ _ _ _ _ w595 _ _ _ _ _ _ _ _ _ _ _ _ _ _ _ _ _ _ _ _ _ _ _ _ _ _ _ _ _]
          tunnel: w272 -> [_ _ _ _ _ w410 _ _ w542 _ _ _ _ w777 _ _ _ _ _ _ _ _ _ _ _ _ _ _ _ _ _ _ _ _ _ _ _ _ _]
          tunnel: w271 -> [_ _ _ _ _ _ _ _ _ _ _ _ w725 _ _ _ _ _ _ _ _ _ _ _ _ _ _ _ _ _ _ _ w1582 _ _ _ _ _ _]
          tunnel: w270 -> [_ _ _ _ _ _ _ _ _ _ _ _ _ _ _ _ _ _ _ _ _ _ _ _ _ _ _ _ _ _ _ _ _ _ _ _ _ _ _]
          tunnel: [State_Type_Definitions,_for_0.26g_versions_and_later_2."Idle" ("Enum") State_Type_Definitions,_for_0.26g_versions_and_later_2."Idle" ("Enum") State_Type_Definitions,_for_0.26g_versions_and_later_2."Idle" ("Enum") State_Type_Definitions,_for_0.26g_versions_and_later_2."Idle" ("Enum") State_Type_Definitions,_for_0.26g_versions_and_later_2."Shutdown" ("Enum") w407 w454 w500 w545 w586 w631 w679 w733 w775 w835 w881 w918 w969 w1010 w1062 w1097 w1150 w1194 w1228 w1266 w1273 w1321 w1363 w1412 w1458 w1495 w1546 w1598 w1633 w1684 w1725 w1777 w1812 w1865] -> w266
          tunnel: w265 -> [_ _ w309 _ _ _ _ _ _ _ _ _ _ _ _ _ _ _ _ _ _ _ _ _ w1266 _ _ _ _ _ _ _ _ _ _ _ _ _ _]
          tunnel: w261 -> [_ _ _ _ _ _ _ _ _ _ _ _ _ _ _ _ _ _ _ _ _ _ _ w1229 _ _ _ _ _ _ _ _ _ _ _ _ _ _ _]
          tunnel: w264 -> [_ _ _ _ _ _ _ _ _ _ _ _ _ _ _ _ _ _ _ _ _ _ _ _ _ _ _ _ _ _ _ _ w1588 _ _ _ _ _ _]
          tunnel: w263 -> [_ _ _ _ _ _ _ _ _ _ _ _ _ _ _ _ _ _ w1005 _ _ _ _ _ _ _ _ _ _ _ _ _ _ _ _ w1720 _ _ _]
          tunnel: w260 -> [_ _ _ _ _ _ _ _ _ _ _ _ _ _ _ _ _ _ w1004 _ _ _ _ _ _ _ _ _ _ _ _ _ _ _ _ w1719 _ _ _]
          tunnel: w259 -> [_ _ _ _ _ _ w453 _ _ _ w629 _ _ _ w828 _ _ _ _ w1055 _ w1143 w1186 _ _ w1276 _ _ w1405 _ _ _ _ _ _ _ w1770 _ w1858]
          tunnel: w257 -> [_ _ _ _ _ _ _ _ _ _ _ _ _ _ _ _ _ _ _ _ _ _ _ _ _ _ _ _ _ _ _ _ _ _ _ _ _ _ _]
          tunnel: w255 -> [_ _ _ _ _ _ _ _ _ _ _ _ _ _ _ _ w916 w959 _ _ w1095 _ _ _ _ _ _ _ _ _ w1493 w1536 _ w1631 w1674 _ _ w1810 _]
          tunnel: w253 -> [w287 w298 w308 w321 w396 w406 w452 w492 w546 w585 w630 w678 w729 w771 w823 w874 w917 w960 w1007 w1050 w1096 w1138 w1183 w1225 w1267 w1270 w1322 w1362 w1400 w1451 w1494 w1537 w1589 w1632 w1675 w1722 w1765 w1811 w1853]
          tunnel: [w287 w297 w308 w321 w396 w406 w452 w492 w546 w585 w630 w678 w729 w771 w823 w874 w917 w960 w1006 w1050 w1096 w1138 w1183 w1225 w1267 w1270 w1322 w1362 w1400 w1451 w1494 w1537 w1589 w1632 w1675 w1721 w1765 w1811 w1853] -> w252
          tunnel: w251 -> [_ _ _ _ _ _ _ _ _ _ _ _ _ _ _ _ _ _ _ _ _ _ _ _ _ _ w1317 _ _ _ _ _ _ _ _ _ _ _ _]
          tunnel: [_ _ _ TRUE _ _ _ _ _ _ _ _ _ _ _ _ _ _ _ _ _ _ _ _ _ _ _ _ _ _ _ _ _ _ _ _ _ _ _] -> w250
          tunnel: w249 -> [_ _ _ _ _ _ _ _ _ _ _ _ _ _ _ _ _ _ _ _ _ _ _ _ _ _ _ _ _ _ _ _ _ _ _ _ _ _ _]
          tunnel: w247 -> [w286 w295 w307 w319 w395 w405 w447 w491 w539 w584 w626 w671 w718 w770 w822 w867 w915 w958 w1001 w1049 w1094 w1137 w1182 w1224 w1268 w1269 w1313 w1359 w1399 w1444 w1492 w1535 w1585 w1630 w1673 w1716 w1764 w1809 w1852]
          tunnel: [w286 w294 w307 w319 w395 w405 w447 w491 w539 w584 w626 w671 w718 w770 w822 w867 w915 w958 w1001 w1049 w1094 w1137 w1182 w1224 w1268 w1269 w1313 w1359 w1399 w1444 w1492 w1535 w1584 w1630 w1673 w1716 w1764 w1809 w1852] -> w246
          frame 0 {
            # ">>> yStepper command>>>"
          }
          frame 1 {
            # ">>> yStepper command>>>"
            n157 = for {
              shift-right: [w306] -> w300
              shift-left: w303 -> [w305]
              tunnel: string[] ["INIT", "RESET ARM", "RESET FLAGS", "RESET YAW", "NAVX CALIBRATE"] -> [w304] mode=indexing
              n158 = Enqueue Element(queue=w305, element=w304) -> (queue out=w306:refnum<queue>)  [unwired: 2 in, 2 out]
            }
            n159 = Bundle By Name(cluster=w298, "yStepper desired"=u8 0) -> (w297:T10)
            n160 = Bundle By Name(cluster=w295, "ySpeed"=0.0, "xSpeed"=0.0, "wSpeed"=0.0) -> (w294:T8)
          }
          frame 3 {
            # ">>> yStepper command>>>"
            n161 = Flush Queue(queue=w312, error in (no error)=w311) -> ()  [unwired: 3 out]
            n162 = for {
              shift-right: [w318] -> w313
              shift-left: w314 -> [w317]
              tunnel: string[] ["STOP", "RESET ENCODERS", "RESET YAW", "RESET ARM", "RESET FLAGS", "DISPOSE BUFFERS", "CAM CLOSE", "DISPOSE ALL BUFFERS"] -> [w316] mode=indexing
              n163 = Enqueue Element(queue=w317, element=w316) -> (queue out=w318:refnum<queue>)  [unwired: 2 in, 2 out]
            }
          }
          frame 4, Default {
            (unwired) TRUE ("Green LED")
            # ">>> yStepper command>>>"
            n164 = Dequeue Element(queue=w329, timeout in ms (-1)=w328, error in (no error)=w324) -> (element=w327:T7)  [unwired: 3 out]
            n165 = case shown="\"Start Task 4\"" w327 {
              tunnel: [w331 w338 w345 w352 w359 w366 w373 w375 w383 w389] -> w323
              tunnel: w326 -> [w332 w339 w346 w353 w360 w367 w373 w376 w382 w390]
              tunnel: [State_Type_Definitions."Task 1" ("Enum") State_Type_Definitions,_for_0.26g_versions_and_later_2."Task 2:Raise Arm" ("Enum") State_Type_Definitions,_for_0.26g_versions_and_later_2."Task 3" ("Enum") State_Type_Definitions,_for_0.26g_versions_and_later_2."Task 4_A" ("Enum") State_Type_Definitions."Task 5A: ARM CAM HEIGHT" ("Enum") State_Type_Definitions,_for_0.26g_versions_and_later_2."Task 6_A" ("Enum") State_Type_Definitions,_for_0.26g_versions_and_later_2."Idle" ("Enum") State_Type_Definitions,_for_0.26g_versions_and_later_2."Shutdown" ("Enum") State_Type_Definitions,_for_0.26g_versions_and_later_2."Task 9A: Raise Arm" ("Enum") State_Type_Definitions,_for_0.26g_versions_and_later_2."Task 8A: RAISE ARM" ("Enum")] -> w325
              frame "Start Task 1" {
                n166 = for {
                  shift-right: [w336] -> w331
                  shift-left: w332 -> [w335]
                  tunnel: string[] ["RESET ENCODERS", "RESET YAW", "FORWARD", "READ ENCODERS"] -> [w334] mode=indexing
                  n167 = Enqueue Element(queue=w335, element=w334) -> (queue out=w336:refnum<queue>)  [unwired: 2 in, 2 out]
                }
              }
              frame "Start Task 2" {
                n168 = for {
                  shift-right: [w343] -> w338
                  shift-left: w339 -> [w342]
                  tunnel: string[] ["RESET ENCODERS", "RESET YAW", "READ ULTRASONIC", "ARDUINO - ULTRASONIC"] -> [w341] mode=indexing
                  n169 = Enqueue Element(queue=w342, element=w341) -> (queue out=w343:refnum<queue>)  [unwired: 2 in, 2 out]
                }
              }
              frame "Start Task 3" {
                n170 = for {
                  shift-right: [w350] -> w345
                  shift-left: w346 -> [w349]
                  tunnel: string[] ["RESET ENCODERS", "READ ENCODERS", "R-ACW"] -> [w348] mode=indexing
                  n171 = Enqueue Element(queue=w349, element=w348) -> (queue out=w350:refnum<queue>)  [unwired: 2 in, 2 out]
                }
              }
              frame "Start Task 4" {
                n172 = for {
                  shift-right: [w357] -> w352
                  shift-left: w353 -> [w356]
                  tunnel: string[] ["RESET YAW", "RESET ENCODERS", "RESET ARM", "RESET FLAGS", "", ""] -> [w355] mode=indexing
                  n173 = Enqueue Element(queue=w356, element=w355) -> (queue out=w357:refnum<queue>)  [unwired: 2 in, 2 out]
                }
              }
              frame "Start Task 5" {
                n174 = for {
                  shift-right: [w364] -> w359
                  shift-left: w360 -> [w363]
                  tunnel: string[] ["RESET YAW", "RESET ENCODERS", "READ STEPPER VALUES", "Z STEPPER CAM HEIGHT", "", ""] -> [w362] mode=indexing
                  n175 = Enqueue Element(queue=w363, element=w362) -> (queue out=w364:refnum<queue>)  [unwired: 2 in, 2 out]
                }
              }
              frame "Start Task 6" {
                n176 = for {
                  shift-right: [w371] -> w366
                  shift-left: w367 -> [w370]
                  tunnel: string[] ["OPEN LOG CAM ", "", "", "", "", ""] -> [w369] mode=indexing
                  n177 = Enqueue Element(queue=w370, element=w369) -> (queue out=w371:refnum<queue>)  [unwired: 2 in, 2 out]
                }
              }
              frame "None", Default {
              }
              frame "Exit" {
                n178 = for {
                  shift-right: [w380] -> w375
                  shift-left: w376 -> [w379]
                  tunnel: string[] ["STOP", "RESET ENCODERS", "RESET YAW", "EXIT"] -> [w378] mode=indexing
                  n179 = Enqueue Element(queue=w379, element=w378) -> (queue out=w380:refnum<queue>)  [unwired: 2 in, 2 out]
                }
              }
              frame "Start Task 9" {
                n180 = for {
                  shift-right: [w387] -> w383
                  shift-left: w382 -> [w386]
                  tunnel: string[] ["RESET ENCODERS", "READ ENCODERS", "Z STEPPER CAM HEIGHT"] -> [w385] mode=indexing
                  n181 = Enqueue Element(queue=w386, element=w385) -> (queue out=w387:refnum<queue>)  [unwired: 2 in, 2 out]
                }
              }
              frame "Start Task 8 - BALL" {
                n182 = for {
                  shift-right: [w394] -> w389
                  shift-left: w390 -> [w393]
                  tunnel: string[] ["RESET YAW", "RESET ENCODERS", "RESET ARM", "RESET FLAGS"] -> [w392] mode=indexing
                  n183 = Enqueue Element(queue=w393, element=w392) -> (queue out=w394:refnum<queue>)  [unwired: 2 in, 2 out]
                }
              }
            }
          }
          frame 5 {
            # ">>> yStepper command>>>"
            n184 = for {
              shift-right: [w404] -> w398
              shift-left: w400 -> [w403]
              tunnel: string[] ["INIT", "RESET ENCODERS", "RESET FLAGS", "CAM CLOSE", "DISPOSE BUFFERS", "EXIT", ""] -> [w402] mode=indexing
              n185 = Enqueue Element(queue=w403, element=w402) -> (queue out=w404:refnum<queue>)  [unwired: 2 in, 2 out]
            }
          }
          frame 6 {
            # ">>> yStepper command>>>"
            # "Use 250"
            n186 = Dequeue Element(queue=w419, timeout in ms (-1)=w418, error in (no error)=w417) -> (element=w416:T7)  [unwired: 3 out]
            n187 = Greater?(x=w410, y=265.0) -> (0:w408:bool)
            n188 = Or(x=w408, y=w411) -> (x .or. y?=w415:bool)
            n189 = case shown="\"None\", Default" w416 {
              tunnel: w415 -> [w422 _]
              tunnel: [w426 State_Type_Definitions,_for_0.26g_versions_and_later_2."True Stop" ("Enum")] -> w414
              tunnel: w413 -> [w423 w441]
              tunnel: [w421 w440] -> w412
              tunnel: [State_Type_Definitions,_for_0.26g_versions_and_later_2."Idle" ("Enum") State_Type_Definitions,_for_0.26g_versions_and_later_2."Shutdown" ("Enum")] -> w407
              frame "None", Default {
                n190 = case shown="True" w422 {
                  tunnel: w423 -> [w429 w435]
                  tunnel: [w428 w433] -> w421
                  frame False {
                    n191 = for {
                      shift-right: [w431] -> w428
                      shift-left: w429 -> [w432]
                      tunnel: string[] ["READ ENCODERS", "READ NAVX", "FORWARD"] ("element") -> [w430] mode=indexing
                      n192 = Enqueue Element(queue=w432, element=w430) -> (queue out=w431:refnum<queue>)  [unwired: 2 in, 2 out]
                    }
                  }
                  frame True {
                    n193 = for {
                      shift-right: [w437] -> w433
                      shift-left: w435 -> [w438]
                      tunnel: string[] ["RESET YAW", "RESET ENCODERS", "STOP", ""] -> [w436] mode=indexing
                      n194 = Enqueue Element(queue=w438, element=w436) -> (queue out=w437:refnum<queue>)  [unwired: 2 in, 2 out]
                    }
                  }
                }
                n195 = Select(t=State_Type_Definitions,_for_0.26g_versions_and_later_2."True Stop" ("Enum"), s=w422, f=State_Type_Definitions."Task 1" ("Enum")) -> (s? t:f=w426:u16)
              }
              frame "Exit" {
                n196 = for {
                  shift-right: [w445] -> w440
                  shift-left: w441 -> [w446]
                  tunnel: string[] ["STOP", "RESET ENCODERS", "RESET YAW", ""] -> [w444] mode=indexing
                  n197 = Enqueue Element(queue=w446, element=w444) -> (queue out=w445:refnum<queue>)  [unwired: 2 in, 2 out]
                }
              }
            }
          }
          frame 8 {
            # ">> Stepper height reeached >>"
            # ">>> yStepper command>>>"
            # ">> Manual override >>"
            n198 = Dequeue Element(queue=w451, timeout in ms (-1)=w450, error in (no error)=w449) -> (element=w460:T7)  [unwired: 3 out]
            n199 = Equal?(x=w453, y=u8 60) -> (x = y?=w458:bool)
            n200 = case shown="\"None\", Default" w460 {
              tunnel: [w471 State_Type_Definitions,_for_0.26g_versions_and_later_2."True Stop" ("Enum")] -> w455
              tunnel: [w469 w486] -> w448
              tunnel: w457 -> [w468 _]
              tunnel: w456 -> [w462 _]
              tunnel: [State_Type_Definitions,_for_0.26g_versions_and_later_2."Idle" ("Enum") State_Type_Definitions,_for_0.26g_versions_and_later_2."Shutdown" ("Enum")] -> w454
              tunnel: w458 -> [w461 _]
              frame "None", Default {
                # ">> WIill proceed to part ii if not manual override >>"
                # ">>If ENABLE or Trigger is set to true>>"
                n201 = Or(x=w461, y=w462) -> (x .or. y?=w463:bool)
                n202 = case shown="True" w461 {
                  tunnel: [w474 w480] -> w469
                  tunnel: w468 -> [w473 w479]
                  frame False {
                    n203 = for {
                      shift-right: [w476] -> w474
                      shift-left: w473 -> [w477]
                      tunnel: string[] ["Z STEPPER CAM HEIGHT", "READ STEPPER VALUES"] ("element") -> [w475] mode=indexing
                      n204 = Enqueue Element(queue=w477, element=w475) -> (queue out=w476:refnum<queue>)  [unwired: 2 in, 2 out]
                    }
                  }
                  frame True {
                    n205 = for {
                      shift-right: [w482] -> w480
                      shift-left: w479 -> [w483]
                      tunnel: string[] ["ARDUINO - ULTRASONIC", "READ ULTRASONIC", "", "", "", ""] -> [w481] mode=indexing
                      n206 = Enqueue Element(queue=w483, element=w481) -> (queue out=w482:refnum<queue>)  [unwired: 2 in, 2 out]
                    }
                  }
                }
                n207 = Select(t=State_Type_Definitions,_for_0.26g_versions_and_later_2."True Stop" ("Enum"), s=w462, f=State_Type_Definitions,_for_0.26g_versions_and_later_2."Task 2:Sensor Mode" ("Enum")) -> (s? t:f=w465:T6)
                n208 = Select(t=w465, s=w463, f=State_Type_Definitions,_for_0.26g_versions_and_later_2."Task 2:Raise Arm" ("Enum")) -> (s? t:f=w471:T6)
              }
              frame "Exit" {
                n209 = for {
                  shift-right: [w489] -> w486
                  shift-left: _ -> [w490]
                  tunnel: string[] ["STOP", "RESET ENCODERS", "RESET YAW", ""] -> [w488] mode=indexing
                  n210 = Enqueue Element(queue=w490, element=w488) -> (queue out=w489:refnum<queue>)  [unwired: 2 in, 2 out]
                }
              }
            }
          }
          frame 9 {
            w506 = u8 20 ("y")
            # ">>> yStepper command>>>"
            # ">>Object detected>>"
            n211 = Dequeue Element(queue=w498, timeout in ms (-1)=w497, error in (no error)=w496) -> (element=w507:T7)  [unwired: 3 out]
            n212 = Less?(x=w494, y=w506) -> (x < y?=w505:bool)
            n213 = Less?(x=w493, y=w506) -> (x < y?=w504:bool)
            n214 = Or(x=w505, y=w504) -> (x .or. y?=w503:bool)
            "Obstacle detected" <- w503
            n215 = case shown="\"None\", Default" w507 {
              tunnel: w503 -> [w510 _]
              tunnel: [w517 State_Type_Definitions,_for_0.26g_versions_and_later_2."True Stop" ("Enum")] -> w502
              tunnel: w495 -> [w509 _]
              tunnel: w499 -> [w516 w533]
              tunnel: [w515 w534] -> w501
              tunnel: [State_Type_Definitions,_for_0.26g_versions_and_later_2."Idle" ("Enum") State_Type_Definitions,_for_0.26g_versions_and_later_2."Shutdown" ("Enum")] -> w500
              frame "None", Default {
                n216 = case shown="True" w510 {
                  tunnel: w516 -> [w520 w527]
                  tunnel: [w521 w526] -> w515
                  frame False {
                    n217 = for {
                      tunnel: string[] ["READ ULTRASONIC", "STOP"] ("element") -> [w522] mode=indexing
                      shift-right: [w524] -> w521
                      shift-left: w520 -> [w523]
                      n218 = Enqueue Element(queue=w523, element=w522) -> (queue out=w524:refnum<queue>)  [unwired: 2 in, 2 out]
                    }
                  }
                  frame True {
                    n219 = for {
                      shift-right: [w529] -> w526
                      shift-left: w527 -> [w530]
                      tunnel: string[] ["RESET ENCODERS", "READ NAVX", "READ ENCODERS"] -> [w528] mode=indexing
                      n220 = Enqueue Element(queue=w530, element=w528) -> (queue out=w529:refnum<queue>)  [unwired: 2 in, 2 out]
                    }
                  }
                }
                n221 = Or(x=w510, y=w509) -> (x .or. y?=w508:bool)
                n222 = Select(t=State_Type_Definitions,_for_0.26g_versions_and_later_2."True Stop" ("Enum"), s=w509, f=State_Type_Definitions,_for_0.26g_versions_and_later_2."Task 2:Reverse Mode" ("Enum")) -> (s? t:f=w511:T6)
                n223 = Select(t=w511, s=w508, f=State_Type_Definitions,_for_0.26g_versions_and_later_2."Task 2:Sensor Mode" ("Enum")) -> (s? t:f=w517:T6)
              }
              frame "Exit" {
                n224 = for {
                  shift-right: [w537] -> w534
                  shift-left: w533 -> [w538]
                  tunnel: string[] ["STOP", "RESET ENCODERS", "RESET YAW", "ARDUINO MODE 0"] -> [w536] mode=indexing
                  n225 = Enqueue Element(queue=w538, element=w536) -> (queue out=w537:refnum<queue>)  [unwired: 2 in, 2 out]
                }
              }
            }
          }
          frame 10 {
            # ">>> yStepper command>>>"
            n226 = Dequeue Element(queue=w548, timeout in ms (-1)=w549, error in (no error)=w550) -> (element=w552:T7)  [unwired: 3 out]
            n227 = Less?(x=w542, y=-50.0) -> (x < y?=w540:bool)
            n228 = case shown="\"None\", Default" w552 {
              tunnel: [w562 State_Type_Definitions,_for_0.26g_versions_and_later_2."True Stop" ("Enum")] -> w544
              tunnel: w551 -> [w555 _]
              tunnel: w547 -> [w561 w578]
              tunnel: [w560 w579] -> w543
              tunnel: [State_Type_Definitions,_for_0.26g_versions_and_later_2."Idle" ("Enum") State_Type_Definitions,_for_0.26g_versions_and_later_2."Shutdown" ("Enum")] -> w545
              tunnel: w540 -> [w553 _]
              frame "None", Default {
                n229 = case shown="False" w553 {
                  tunnel: w561 -> [w565 w572]
                  tunnel: [w566 w571] -> w560
                  frame False {
                    n230 = for {
                      tunnel: string[] ["READ ENCODERS", "REVERSE", "READ NAVX"] ("element") -> [w567] mode=indexing
                      shift-right: [w569] -> w566
                      shift-left: w565 -> [w568]
                      n231 = Enqueue Element(queue=w568, element=w567) -> (queue out=w569:refnum<queue>)  [unwired: 2 in, 2 out]
                    }
                  }
                  frame True {
                    n232 = for {
                      shift-right: [w574] -> w571
                      shift-left: w572 -> [w575]
                      tunnel: string[] ["STOP", "ARDUINO - ULTRASONIC", "READ ULTRASONIC", "RESET ENCODERS"] -> [w573] mode=indexing
                      n233 = Enqueue Element(queue=w575, element=w573) -> (queue out=w574:refnum<queue>)  [unwired: 2 in, 2 out]
                    }
                  }
                }
                n234 = Or(x=w553, y=w555) -> (x .or. y?=w554:bool)
                n235 = Select(t=State_Type_Definitions,_for_0.26g_versions_and_later_2."True Stop" ("Enum"), s=w555, f=State_Type_Definitions,_for_0.26g_versions_and_later_2."Task 2:Sensor Mode" ("Enum")) -> (s? t:f=w556:T6)
                n236 = Select(t=w556, s=w554, f=State_Type_Definitions,_for_0.26g_versions_and_later_2."Task 2:Reverse Mode" ("Enum")) -> (s? t:f=w562:T6)
              }
              frame "Exit" {
                n237 = for {
                  shift-right: [w582] -> w579
                  shift-left: w578 -> [w583]
                  tunnel: string[] ["STOP", "RESET ENCODERS", "RESET YAW", "ARDUINO MODE 0"] -> [w581] mode=indexing
                  n238 = Enqueue Element(queue=w583, element=w581) -> (queue out=w582:refnum<queue>)  [unwired: 2 in, 2 out]
                }
              }
            }
          }
          frame 11 {
            # ">>> yStepper command>>>"
            n239 = Dequeue Element(queue=w598, timeout in ms (-1)=w597, error in (no error)=w596) -> (element=w587:T7)  [unwired: 3 out]
            n240 = Greater?(x=w595, y=160.0) -> (0:w592:bool)
            n241 = Or(x=w592, y=w593) -> (x .or. y?=w588:bool)
            n242 = case shown="\"None\", Default" w587 {
              tunnel: w588 -> [w601 _]
              tunnel: [w605 State_Type_Definitions,_for_0.26g_versions_and_later_2."True Stop" ("Enum")] -> w589
              tunnel: w591 -> [w602 w621]
              tunnel: [w600 w620] -> w590
              tunnel: [State_Type_Definitions,_for_0.26g_versions_and_later_2."Idle" ("Enum") State_Type_Definitions,_for_0.26g_versions_and_later_2."Shutdown" ("Enum")] -> w586
              frame "None", Default {
                n243 = case shown="False" w601 {
                  tunnel: w602 -> [w608 w614]
                  tunnel: [w607 w612] -> w600
                  frame False {
                    n244 = for {
                      shift-right: [w610] -> w607
                      shift-left: w608 -> [w611]
                      tunnel: string[] ["READ ENCODERS", "R-CW"] ("element") -> [w609] mode=indexing
                      n245 = Enqueue Element(queue=w611, element=w609) -> (queue out=w610:refnum<queue>)  [unwired: 2 in, 2 out]
                    }
                  }
                  frame True {
                    n246 = for {
                      shift-right: [w616] -> w612
                      shift-left: w614 -> [w617]
                      tunnel: string[] ["RESET YAW", "RESET ENCODERS", "STOP", "ARDUINO MODE 0"] -> [w615] mode=indexing
                      n247 = Enqueue Element(queue=w617, element=w615) -> (queue out=w616:refnum<queue>)  [unwired: 2 in, 2 out]
                    }
                  }
                }
                n248 = Select(t=State_Type_Definitions,_for_0.26g_versions_and_later_2."True Stop" ("Enum"), s=w601, f=State_Type_Definitions,_for_0.26g_versions_and_later_2."Task 3" ("Enum")) -> (s? t:f=w605:T6)
              }
              frame "Exit" {
                n249 = for {
                  shift-right: [w624] -> w620
                  shift-left: w621 -> [w625]
                  tunnel: string[] ["STOP", "RESET ENCODERS", "RESET YAW", ""] -> [w623] mode=indexing
                  n250 = Enqueue Element(queue=w625, element=w623) -> (queue out=w624:refnum<queue>)  [unwired: 2 in, 2 out]
                }
              }
            }
          }
          frame 12 {
            # ">> Stepper height reeached >>"
            # ">>> yStepper command>>>"
            # ">> Manual override >>"
            n251 = Dequeue Element(queue=w638, timeout in ms (-1)=w637, error in (no error)=w636) -> (element=w635:T7)  [unwired: 3 out]
            n252 = Equal?(x=w629, y=u8 60) -> (x = y?=w627:bool)
            n253 = case shown="\"Exit\"" w635 {
              tunnel: [w650 State_Type_Definitions,_for_0.26g_versions_and_later_2."True Stop" ("Enum")] -> w634
              tunnel: [w648 w666] -> w633
              tunnel: w639 -> [w647 w663]
              tunnel: w632 -> [w641 _]
              tunnel: [State_Type_Definitions,_for_0.26g_versions_and_later_2."Idle" ("Enum") State_Type_Definitions,_for_0.26g_versions_and_later_2."Shutdown" ("Enum")] -> w631
              tunnel: w627 -> [w640 _]
              frame "None", Default {
                # ">> WIill proceed to part ii if not manual override >>"
                # ">>If ENABLE or Trigger is set to true>>"
                n254 = Or(x=w640, y=w641) -> (x .or. y?=w642:bool)
                n255 = case shown="False" w640 {
                  tunnel: [w653 w659] -> w648
                  tunnel: w647 -> [w652 w658]
                  frame False {
                    n256 = for {
                      shift-right: [w655] -> w653
                      shift-left: w652 -> [w656]
                      tunnel: string[] ["Z STEPPER CAM HEIGHT", "READ STEPPER VALUES"] ("element") -> [w654] mode=indexing
                      n257 = Enqueue Element(queue=w656, element=w654) -> (queue out=w655:refnum<queue>)  [unwired: 2 in, 2 out]
                    }
                  }
                  frame True {
                    n258 = for {
                      shift-right: [w661] -> w659
                      shift-left: w658 -> [w662]
                      tunnel: string[] ["ARDUINO - ULTRASONIC", "READ ULTRASONIC", "FORWARD", "", "", ""] -> [w660] mode=indexing
                      n259 = Enqueue Element(queue=w662, element=w660) -> (queue out=w661:refnum<queue>)  [unwired: 2 in, 2 out]
                    }
                  }
                }
                n260 = Select(t=State_Type_Definitions,_for_0.26g_versions_and_later_2."True Stop" ("Enum"), s=w641, f=State_Type_Definitions,_for_0.26g_versions_and_later_2."Task 4_B" ("Enum")) -> (s? t:f=w644:T6)
                n261 = Select(t=w644, s=w642, f=State_Type_Definitions,_for_0.26g_versions_and_later_2."Task 4_A" ("Enum")) -> (s? t:f=w650:T6)
              }
              frame "Exit" {
                n262 = for {
                  shift-right: [w669] -> w666
                  shift-left: w663 -> [w670]
                  tunnel: string[] ["STOP", "RESET ENCODERS", "RESET YAW", ""] -> [w668] mode=indexing
                  n263 = Enqueue Element(queue=w670, element=w668) -> (queue out=w669:refnum<queue>)  [unwired: 2 in, 2 out]
                }
              }
            }
          }
          frame 13 {
            w675 = u8 20
            # ">> Path blocked >>"
            # ">>> yStepper command>>>"
            # ">> Manual override >>"
            n264 = Dequeue Element(queue=w684, timeout in ms (-1)=w683, error in (no error)=w682) -> (element=w681:T7)  [unwired: 3 out]
            n265 = Less?(x=w677, y=w675) -> (x < y?=w672:bool)
            n266 = Less?(x=w676, y=w675) -> (x < y?=w673:bool)
            n267 = And(x=w673, y=w672) -> (x .and. y?=w674:bool)
            n268 = case shown="\"None\", Default" w681 {
              tunnel: [w698 State_Type_Definitions,_for_0.26g_versions_and_later_2."True Stop" ("Enum")] -> w686
              tunnel: [w696 w713] -> w687
              tunnel: w680 -> [w695 _]
              tunnel: w685 -> [w689 _]
              tunnel: [State_Type_Definitions,_for_0.26g_versions_and_later_2."Idle" ("Enum") State_Type_Definitions,_for_0.26g_versions_and_later_2."Shutdown" ("Enum")] -> w679
              tunnel: w674 -> [w688 _]
              frame "None", Default {
                # ">> Manual override forces program to true stop >>"
                # ">>If ENABLE or Trigger is set to true>>"
                n269 = Or(x=w688, y=w689) -> (x .or. y?=w694:bool)
                n270 = case shown="True" w688 {
                  tunnel: [w701 w706] -> w696
                  tunnel: w695 -> [w700 w705]
                  frame False {
                    n271 = for {
                      shift-right: [w703] -> w701
                      shift-left: w700 -> [w704]
                      tunnel: string[] ["FORWARD", "READ ULTRASONIC", "READ NAVX"] ("element") -> [w702] mode=indexing
                      n272 = Enqueue Element(queue=w704, element=w702) -> (queue out=w703:refnum<queue>)  [unwired: 2 in, 2 out]
                    }
                  }
                  frame True {
                    n273 = for {
                      shift-right: [w709] -> w706
                      shift-left: w705 -> [w710]
                      tunnel: string[] ["STOP", "RESET YAW", "RESET ENCODERS", "RESET FLAGS"] -> [w708] mode=indexing
                      n274 = Enqueue Element(queue=w710, element=w708) -> (queue out=w709:refnum<queue>)  [unwired: 2 in, 2 out]
                    }
                  }
                }
                n275 = Select(t=State_Type_Definitions,_for_0.26g_versions_and_later_2."True Stop" ("Enum"), s=w689, f=State_Type_Definitions,_for_0.26g_versions_and_later_2."Task 4_C" ("Enum")) -> (s? t:f=w691:T6)
                n276 = Select(t=w691, s=w694, f=State_Type_Definitions,_for_0.26g_versions_and_later_2."Task 4_B" ("Enum")) -> (s? t:f=w698:T6)
              }
              frame "Exit" {
                n277 = for {
                  shift-right: [w716] -> w713
                  shift-left: _ -> [w717]
                  tunnel: string[] ["STOP", "RESET ENCODERS", "RESET YAW", ""] -> [w715] mode=indexing
                  n278 = Enqueue Element(queue=w717, element=w715) -> (queue out=w716:refnum<queue>)  [unwired: 2 in, 2 out]
                }
              }
            }
          }
          frame 14 {
            w728 = u8 20
            # ">> xDistance travelled>>"
            # ">> Path NOT blocked >>"
            # ">>> yStepper command>>>"
            # ">> Manual override >>"
            n279 = Dequeue Element(queue=w738, timeout in ms (-1)=w731, error in (no error)=w730) -> (element=w732:T7)  [unwired: 3 out]
            n280 = Greater?(x=w720, y=w728) -> (0:w726:bool)
            n281 = Greater?(x=w725, y=80.0) -> (0:w723:bool)
            n282 = Greater?(x=w719, y=w728) -> (0:w727:bool)
            n283 = And(x=w727, y=w726) -> (x .and. y?=w722:bool)
            n284 = And(x=w723, y=w722) -> (x .and. y?=w721:bool)
            n285 = case shown="\"Exit\"" w732 {
              tunnel: [w749 State_Type_Definitions,_for_0.26g_versions_and_later_2."True Stop" ("Enum")] -> w735
              tunnel: [w747 w765] -> w734
              tunnel: w737 -> [w746 w762]
              tunnel: w736 -> [w740 _]
              tunnel: [State_Type_Definitions,_for_0.26g_versions_and_later_2."Idle" ("t") State_Type_Definitions,_for_0.26g_versions_and_later_2."Shutdown" ("Enum")] -> w733
              tunnel: w721 -> [w739 _]
              frame "None", Default {
                # ">> Manual override forces program to true stop >>"
                # ">>If ENABLE or Trigger is set to true>>"
                n286 = Or(x=w739, y=w740) -> (x .or. y?=w745:bool)
                n287 = case shown="False" w739 {
                  tunnel: [w752 w757] -> w747
                  tunnel: w746 -> [w750 w756]
                  frame False {
                    n288 = for {
                      shift-right: [w754] -> w752
                      shift-left: w750 -> [w755]
                      tunnel: string[] ["RIGHT", "READ NAVX", "READ ENCODERS", "READ ULTRASONIC"] ("element") -> [w753] mode=indexing
                      n289 = Enqueue Element(queue=w755, element=w753) -> (queue out=w754:refnum<queue>)  [unwired: 2 in, 2 out]
                    }
                  }
                  frame True {
                    n290 = for {
                      shift-right: [w760] -> w757
                      shift-left: w756 -> [w761]
                      tunnel: string[] ["STOP", "RESET YAW", "RESET ENCODERS", "ARDUINO - ULTRASONIC"] -> [w759] mode=indexing
                      n291 = Enqueue Element(queue=w761, element=w759) -> (queue out=w760:refnum<queue>)  [unwired: 2 in, 2 out]
                    }
                  }
                }
                n292 = Select(t=State_Type_Definitions,_for_0.26g_versions_and_later_2."True Stop" ("Enum"), s=w740, f=State_Type_Definitions,_for_0.26g_versions_and_later_2."Task 4_D" ("Enum")) -> (s? t:f=w741:T6)
                n293 = Select(t=w741, s=w745, f=State_Type_Definitions,_for_0.26g_versions_and_later_2."Task 4_C" ("Enum")) -> (s? t:f=w749:T6)
              }
              frame "Exit" {
                n294 = for {
                  shift-right: [w768] -> w765
                  shift-left: w762 -> [w769]
                  tunnel: string[] ["STOP", "RESET ENCODERS", "RESET YAW", ""] -> [w767] mode=indexing
                  n295 = Enqueue Element(queue=w769, element=w767) -> (queue out=w768:refnum<queue>)  [unwired: 2 in, 2 out]
                }
              }
            }
          }
          frame 15 {
            w789 = u8 20
            # ">> yDistance travelled>>"
            # ">> Path blocked >>"
            # ">>> yStepper command>>>"
            # ">> Manual override >>"
            n296 = Dequeue Element(queue=w780, timeout in ms (-1)=w779, error in (no error)=w778) -> (element=w790:T7)  [unwired: 3 out]
            n297 = Less?(x=w773, y=w789) -> (x < y?=w787:bool)
            n298 = Greater?(x=w777, y=200.0) -> (0:w785:bool)
            n299 = Less?(x=w772, y=w789) -> (x < y?=w788:bool)
            n300 = And(x=w788, y=w787) -> (x .and. y?=w784:bool)
            n301 = Or(x=w785, y=w784) -> (x .or. y?=w783:bool)
            n302 = case shown="\"None\", Default" w790 {
              tunnel: [w801 State_Type_Definitions,_for_0.26g_versions_and_later_2."True Stop" ("Enum")] -> w776
              tunnel: [w799 w817] -> w774
              tunnel: w781 -> [w798 w814]
              tunnel: w782 -> [w792 _]
              tunnel: [State_Type_Definitions,_for_0.26g_versions_and_later_2."Idle" ("t") State_Type_Definitions,_for_0.26g_versions_and_later_2."Shutdown" ("Enum")] -> w775
              tunnel: w783 -> [w791 _]
              frame "None", Default {
                # ">> Manual override forces program to true stop >>"
                # ">>If ENABLE or Trigger is set to true>>"
                n303 = Or(x=w791, y=w792) -> (x .or. y?=w797:bool)
                n304 = case shown="True" w791 {
                  tunnel: [w804 w809] -> w799
                  tunnel: w798 -> [w802 w808]
                  frame False {
                    n305 = for {
                      shift-right: [w806] -> w804
                      shift-left: w802 -> [w807]
                      tunnel: string[] ["FORWARD", "READ NAVX", "READ ENCODERS", "READ ULTRASONIC"] ("element") -> [w805] mode=indexing
                      n306 = Enqueue Element(queue=w807, element=w805) -> (queue out=w806:refnum<queue>)  [unwired: 2 in, 2 out]
                    }
                  }
                  frame True {
                    n307 = for {
                      shift-right: [w812] -> w809
                      shift-left: w808 -> [w813]
                      tunnel: string[] ["STOP", "RESET YAW", "RESET ENCODERS", "RESET FLAGS"] -> [w811] mode=indexing
                      n308 = Enqueue Element(queue=w813, element=w811) -> (queue out=w812:refnum<queue>)  [unwired: 2 in, 2 out]
                    }
                  }
                }
                n309 = Select(t=State_Type_Definitions,_for_0.26g_versions_and_later_2."True Stop" ("Enum"), s=w792, f=State_Type_Definitions,_for_0.26g_versions_and_later_2."True Stop" ("Enum")) -> (s? t:f=w793:T6)
                n310 = Select(t=w793, s=w797, f=State_Type_Definitions,_for_0.26g_versions_and_later_2."Task 4_D" ("Enum")) -> (s? t:f=w801:T6)
              }
              frame "Exit" {
                n311 = for {
                  shift-right: [w820] -> w817
                  shift-left: w814 -> [w821]
                  tunnel: string[] ["STOP", "RESET ENCODERS", "RESET YAW", ""] -> [w819] mode=indexing
                  n312 = Enqueue Element(queue=w821, element=w819) -> (queue out=w820:refnum<queue>)  [unwired: 2 in, 2 out]
                }
              }
            }
          }
          frame 15 {
            # ">>> yStepper command>>>"
            # ">> Manual override >>"
            n313 = Dequeue Element(queue=w831, timeout in ms (-1)=w830, error in (no error)=w832) -> (element=w829:T7)  [unwired: 3 out]
            n314 = Equal?(x=w828, y=u8 60) -> (x = y?=w826:bool)
            n315 = case shown="\"None\", Default" w829 {
              tunnel: [w842 State_Type_Definitions,_for_0.26g_versions_and_later_2."True Stop" ("Enum")] -> w833
              tunnel: [w845 w862] -> w834
              tunnel: [State_Type_Definitions,_for_0.26g_versions_and_later_2."Idle" ("Enum") State_Type_Definitions,_for_0.26g_versions_and_later_2."Shutdown" ("Enum")] -> w835
              tunnel: w826 -> [w841 _]
              tunnel: w825 -> [w840 _]
              tunnel: w824 -> [w836 w859]
              frame "None", Default {
                # "Stays in Task 5_A until stepper reaches desired \nheight"
                # "T: Go back to idle, F: Continue with task\""
                # ">> Manual override >>"
                n316 = case shown="True" w841 {
                  tunnel: [w849 w855] -> w845
                  tunnel: w836 -> [w847 w853]
                  frame False {
                    n317 = for {
                      tunnel: string[] ["Z STEPPER CAM HEIGHT", "READ STEPPER VALUES"] ("element") -> [w850] mode=indexing
                      shift-right: [w852] -> w849
                      shift-left: w847 -> [w851]
                      n318 = Enqueue Element(queue=w851, element=w850) -> (queue out=w852:refnum<queue>)  [unwired: 2 in, 2 out]
                    }
                  }
                  frame True {
                    n319 = for {
                      shift-right: [w857] -> w855
                      shift-left: w853 -> [w858]
                      tunnel: string[] ["ARDUINO - ULTRASONIC", "READ ULTRASONIC", ""] -> [w856] mode=indexing
                      n320 = Enqueue Element(queue=w858, element=w856) -> (queue out=w857:refnum<queue>)  [unwired: 2 in, 2 out]
                    }
                  }
                }
                n321 = Or(x=w841, y=w840) -> (x .or. y?=w843:bool)
                n322 = Select(t=State_Type_Definitions,_for_0.26g_versions_and_later_2."True Stop" ("Enum"), s=w840, f=State_Type_Definitions."Task 5B: MOVE TO BOX" ("Enum")) -> (s? t:f=w837:u16)
                n323 = Select(t=w837, s=w843, f=State_Type_Definitions."Task 5A: ARM CAM HEIGHT" ("Enum")) -> (s? t:f=w842:u16)
              }
              frame "Exit" {
                n324 = for {
                  shift-right: [w865] -> w862
                  shift-left: w859 -> [w866]
                  tunnel: string[] ["STOP", "RESET ENCODERS", "RESET YAW", "ARDUINO MODE 0"] -> [w864] mode=indexing
                  n325 = Enqueue Element(queue=w866, element=w864) -> (queue out=w865:refnum<queue>)  [unwired: 2 in, 2 out]
                }
              }
            }
          }
          frame 16 {
            w873 = u8 20 ("y")
            # ">>> yStepper command>>>"
            n326 = Less?(x=w870, y=w873) -> (x < y?=w871:bool)
            n327 = Dequeue Element(queue=w877, timeout in ms (-1)=w876, error in (no error)=w878) -> (element=w875:T7)  [unwired: 3 out]
            n328 = Less?(x=w869, y=w873) -> (x < y?=w872:bool)
            n329 = And(x=w872, y=w871) -> (x .and. y?=w868:bool)
            n330 = case shown="\"None\", Default" w875 {
              tunnel: [w890 State_Type_Definitions,_for_0.26g_versions_and_later_2."True Stop" ("Enum")] -> w880
              tunnel: [w893 w910] -> w879
              tunnel: [State_Type_Definitions,_for_0.26g_versions_and_later_2."Idle" ("Enum") State_Type_Definitions,_for_0.26g_versions_and_later_2."Shutdown" ("Enum")] -> w881
              tunnel: w883 -> [w889 _]
              tunnel: w882 -> [w885 w907]
              tunnel: w868 -> [w884 _]
              frame "None", Default {
                # "Stays in Task 5_B to capture image over 5 seconds"
                # "T: Go back to idle, F: Continue with task\""
                # ">> Manual override >>"
                n331 = case shown="True" w884 {
                  tunnel: [w897 w903] -> w893
                  tunnel: w885 -> [w895 w901]
                  frame False {
                    n332 = for {
                      tunnel: string[] ["FORWARD", "READ ULTRASONIC", "READ NAVX"] ("element") -> [w898] mode=indexing
                      shift-right: [w900] -> w897
                      shift-left: w895 -> [w899]
                      n333 = Enqueue Element(queue=w899, element=w898) -> (queue out=w900:refnum<queue>)  [unwired: 2 in, 2 out]
                    }
                  }
                  frame True {
                    n334 = for {
                      shift-right: [w905] -> w903
                      shift-left: w901 -> [w906]
                      tunnel: string[] ["STOP", "RESET ENCODERS", "OPEN LOG CAM", "SET TIMER 5"] -> [w904] mode=indexing
                      n335 = Enqueue Element(queue=w906, element=w904) -> (queue out=w905:refnum<queue>)  [unwired: 2 in, 2 out]
                    }
                  }
                }
                n336 = Or(x=w884, y=w889) -> (x .or. y?=w891:bool)
                n337 = Select(t=State_Type_Definitions,_for_0.26g_versions_and_later_2."True Stop" ("Enum"), s=w889, f=State_Type_Definitions."Task 5C: CAM BURST" ("Enum")) -> (s? t:f=w886:u16)
                n338 = Select(t=w886, s=w891, f=State_Type_Definitions."Task 5B: MOVE TO BOX" ("Enum")) -> (s? t:f=w890:u16)
              }
              frame "Exit" {
                n339 = for {
                  shift-right: [w913] -> w910
                  shift-left: w907 -> [w914]
                  tunnel: string[] ["STOP", "RESET ENCODERS", "RESET YAW", "ARDUINO MODE 0"] -> [w912] mode=indexing
                  n340 = Enqueue Element(queue=w914, element=w912) -> (queue out=w913:refnum<queue>)  [unwired: 2 in, 2 out]
                }
              }
            }
          }
          frame 17 {
            # ">>> Motor control cluster >>>"
            # ">>> yStepper command>>>"
            # ">> Manual override >>"
            n341 = Dequeue Element(queue=w924, timeout in ms (-1)=w923, error in (no error)=w922) -> (element=w921:T7)  [unwired: 3 out]
            n342 = case shown="\"None\", Default" w921 {
              tunnel: [w933 State_Type_Definitions,_for_0.26g_versions_and_later_2."True Stop" ("Enum")] -> w926
              tunnel: [w936 w953] -> w919
              tunnel: [State_Type_Definitions,_for_0.26g_versions_and_later_2."Idle" ("Enum") State_Type_Definitions,_for_0.26g_versions_and_later_2."Shutdown" ("Enum")] -> w918
              tunnel: w920 -> [w927 _]
              tunnel: w925 -> [w932 w950]
              tunnel: w916 -> [w931 _]
              frame "None", Default {
                # ">> Is time up? >>"
                # "Determines if object is in range to pick up"
                # ">> Manual override >>"
                n343 = case shown="False" w931 {
                  tunnel: [w940 w946] -> w936
                  tunnel: w932 -> [w938 w944]
                  frame False {
                    n344 = for {
                      tunnel: string[] ["CAM ACQ", "START TIMER"] ("element") -> [w941] mode=indexing
                      shift-right: [w943] -> w940
                      shift-left: w938 -> [w942]
                      n345 = Enqueue Element(queue=w942, element=w941) -> (queue out=w943:refnum<queue>)  [unwired: 2 in, 2 out]
                    }
                  }
                  frame True {
                    n346 = for {
                      shift-right: [w948] -> w946
                      shift-left: w944 -> [w949]
                      tunnel: string[] ["CAM CLOSE", "PROCESS IMAGE", "SET TIMER 5"] -> [w947] mode=indexing
                      n347 = Enqueue Element(queue=w949, element=w947) -> (queue out=w948:refnum<queue>)  [unwired: 2 in, 2 out]
                    }
                  }
                }
                n348 = Or(x=w931, y=w927) -> (x .or. y?=w934:bool)
                n349 = Select(t=State_Type_Definitions,_for_0.26g_versions_and_later_2."True Stop" ("Enum"), s=w927, f=State_Type_Definitions."Task 5D: PROCESS IMAGE" ("Enum")) -> (s? t:f=w929:u16)
                n350 = Select(t=w929, s=w934, f=State_Type_Definitions."Task 5C: CAM BURST" ("Enum")) -> (s? t:f=w933:u16)
              }
              frame "Exit" {
                n351 = for {
                  shift-right: [w956] -> w953
                  shift-left: w950 -> [w957]
                  tunnel: string[] ["STOP", "RESET ENCODERS", "RESET YAW", "ARDUINO MODE 0"] -> [w955] mode=indexing
                  n352 = Enqueue Element(queue=w957, element=w955) -> (queue out=w956:refnum<queue>)  [unwired: 2 in, 2 out]
                }
              }
            }
          }
          frame 18 {
            # ">>> yStepper command>>>"
            n353 = Dequeue Element(queue=w964, timeout in ms (-1)=w963, error in (no error)=w962) -> (element=w961:T7)  [unwired: 3 out]
            n354 = case shown="\"None\", Default" w961 {
              tunnel: [w976 State_Type_Definitions,_for_0.26g_versions_and_later_2."True Stop" ("Enum")] -> w968
              tunnel: [w979 w996] -> w967
              tunnel: [State_Type_Definitions,_for_0.26g_versions_and_later_2."Idle" ("Enum") State_Type_Definitions,_for_0.26g_versions_and_later_2."Shutdown" ("Enum")] -> w969
              tunnel: w965 -> [w975 _]
              tunnel: w966 -> [w971 w993]
              tunnel: w959 -> [w970 _]
              frame "None", Default {
                # ">> T: Breaks out of state loop; F: Stays in loop>>"
                # ">> Manual override >>"
                # ">> Checks if time is up>>"
                # "Stays in Task 5D until the object is detected"
                # "T: Go back to idle, F: Continue with task\""
                # ">> Manual override >>"
                n355 = case shown="True" w970 {
                  tunnel: [w983 w989] -> w979
                  tunnel: w971 -> [w981 w987]
                  frame False {
                    n356 = for {
                      tunnel: string[] ["START TIMER", "PROCESS IMAGE", ""] ("element") -> [w984] mode=indexing
                      shift-right: [w986] -> w983
                      shift-left: w981 -> [w985]
                      n357 = Enqueue Element(queue=w985, element=w984) -> (queue out=w986:refnum<queue>)  [unwired: 2 in, 2 out]
                    }
                  }
                  frame True {
                    n358 = for {
                      shift-right: [w991] -> w989
                      shift-left: w987 -> [w992]
                      tunnel: string[] ["CAM CLOSE", "", ""] -> [w990] mode=indexing
                      n359 = Enqueue Element(queue=w992, element=w990) -> (queue out=w991:refnum<queue>)  [unwired: 2 in, 2 out]
                    }
                  }
                }
                n360 = Or(x=w970, y=w975) -> (x .or. y?=w977:bool)
                n361 = Select(t=State_Type_Definitions,_for_0.26g_versions_and_later_2."True Stop" ("Enum"), s=w975, f=State_Type_Definitions,_for_0.26g_versions_and_later_2."Task 5E: POSITION ARM" ("Enum")) -> (s? t:f=w972:T6)
                n362 = Select(t=w972, s=w977, f=State_Type_Definitions."Task 5D: PROCESS IMAGE" ("Enum")) -> (s? t:f=w976:u16)
              }
              frame "Exit" {
                n363 = for {
                  shift-right: [w999] -> w996
                  shift-left: w993 -> [w1000]
                  tunnel: string[] ["STOP", "RESET ENCODERS", "RESET YAW", "ARDUINO MODE 0"] -> [w998] mode=indexing
                  n364 = Enqueue Element(queue=w1000, element=w998) -> (queue out=w999:refnum<queue>)  [unwired: 2 in, 2 out]
                }
              }
            }
          }
          frame 20 {
            # ">>> yStepper command>>>"
            n365 = Dequeue Element(queue=w1013, timeout in ms (-1)=w1014, error in (no error)=w1015) -> (element=w1017:T7)  [unwired: 3 out]
            n366 = formula code="if (pos < 100)\ny = 41;\n\nelse if (pos >= 100 && pos <= 140)\ny = 30;\n\nelse if (pos >= 141 && pos <= 170)\ny = 25;\n\nelse if (pos >= 171 &&pos <= 180) \ny = 20;\n\nelse if (pos >= 181&& pos <= 200)\ny = 15;\n\nelse if (pos >= 201 && pos <= 230)\ny = 10;\n\nelse if (pos >= 231 && pos <= 320)\ny = 8;\n\nelse if (pos > 320)\ny = 0;"("pos"=w1005) -> ("y"=w1008:dbl)
            n367 = To Unsigned Byte Integer(number=w1008) -> (unsigned 8bit integer=w1003:u8)
            n368 = Equal?(x=w1004, y=w1003) -> (x = y?=w1002:bool)
            n369 = case shown="\"None\", Default" w1017 {
              tunnel: [w1024 State_Type_Definitions,_for_0.26g_versions_and_later_2."True Stop" ("Enum")] -> w1011
              tunnel: [w1027 w1044] -> w1009
              tunnel: [State_Type_Definitions,_for_0.26g_versions_and_later_2."Idle" ("Enum") State_Type_Definitions,_for_0.26g_versions_and_later_2."Shutdown" ("Enum")] -> w1010
              tunnel: w1016 -> [w1023 _]
              tunnel: w1012 -> [w1019 w1041]
              tunnel: w1002 -> [w1018 _]
              frame "None", Default {
                # ">> T: Breaks out of state loop; F: Stays in loop>>"
                # ">> Manual override >>"
                # ">> Checks if time is up>>"
                # "Stays in Task 5D until the object is detected"
                # "T: Go back to idle, F: Continue with task\""
                # ">> Manual override >>"
                n370 = case shown="False" w1018 {
                  tunnel: [w1031 w1037] -> w1027
                  tunnel: w1019 -> [w1029 w1035]
                  frame False {
                    n371 = for {
                      tunnel: string[] ["READ STEPPER VALUES", "Y STEPPER CONTROL", ""] ("element") -> [w1032] mode=indexing
                      shift-right: [w1034] -> w1031
                      shift-left: w1029 -> [w1033]
                      n372 = Enqueue Element(queue=w1033, element=w1032) -> (queue out=w1034:refnum<queue>)  [unwired: 2 in, 2 out]
                    }
                  }
                  frame True {
                    n373 = for {
                      shift-right: [w1039] -> w1037
                      shift-left: w1035 -> [w1040]
                      tunnel: string[] ["CAM CLOSE", "DISPOSE BUFFERS", ""] -> [w1038] mode=indexing
                      n374 = Enqueue Element(queue=w1040, element=w1038) -> (queue out=w1039:refnum<queue>)  [unwired: 2 in, 2 out]
                    }
                  }
                }
                n375 = Or(x=w1018, y=w1023) -> (x .or. y?=w1025:bool)
                n376 = Select(t=State_Type_Definitions,_for_0.26g_versions_and_later_2."True Stop" ("Enum"), s=w1023, f=State_Type_Definitions,_for_0.26g_versions_and_later_2."Task 5F: ARM GRAB HEIGHT" ("Enum")) -> (s? t:f=w1020:T6)
                n377 = Select(t=w1020, s=w1025, f=State_Type_Definitions,_for_0.26g_versions_and_later_2."Task 5E: POSITION ARM" ("Enum")) -> (s? t:f=w1024:T6)
              }
              frame "Exit" {
                n378 = for {
                  shift-right: [w1047] -> w1044
                  shift-left: w1041 -> [w1048]
                  tunnel: string[] ["STOP", "RESET ENCODERS", "RESET YAW", "ARDUINO MODE 0"] -> [w1046] mode=indexing
                  n379 = Enqueue Element(queue=w1048, element=w1046) -> (queue out=w1047:refnum<queue>)  [unwired: 2 in, 2 out]
                }
              }
            }
            n380 = Bundle By Name(cluster=w1007, "yStepper desired"=w1003) -> (w1006:T10)
          }
          frame 21 {
            # ">>> Motor control cluster >>>"
            # ">>> yStepper command>>>"
            # ">> Manual override >>"
            n381 = Dequeue Element(queue=w1058, timeout in ms (-1)=w1057, error in (no error)=w1059) -> (element=w1056:T7)  [unwired: 3 out]
            n382 = Equal?(x=w1055, y=u8 1) -> (x = y?=w1053:bool)
            n383 = case shown="\"None\", Default" w1056 {
              tunnel: [w1069 State_Type_Definitions,_for_0.26g_versions_and_later_2."True Stop" ("Enum")] -> w1060
              tunnel: [w1072 w1089] -> w1061
              tunnel: [State_Type_Definitions,_for_0.26g_versions_and_later_2."Idle" ("Enum") State_Type_Definitions,_for_0.26g_versions_and_later_2."Shutdown" ("Enum")] -> w1062
              tunnel: w1053 -> [w1068 _]
              tunnel: w1052 -> [w1067 _]
              tunnel: w1051 -> [w1063 w1086]
              frame "None", Default {
                # "Stays in Task 5F until stepper reaches desired \nheight"
                # "T: Go back to idle, F: Continue with task\""
                # ">> Manual override >>"
                n384 = case shown="True" w1068 {
                  tunnel: [w1076 w1082] -> w1072
                  tunnel: w1063 -> [w1074 w1080]
                  frame False {
                    n385 = for {
                      tunnel: string[] ["Z STEPPER GRAB HEIGHT", "READ STEPPER VALUES"] ("element") -> [w1077] mode=indexing
                      shift-right: [w1079] -> w1076
                      shift-left: w1074 -> [w1078]
                      n386 = Enqueue Element(queue=w1078, element=w1077) -> (queue out=w1079:refnum<queue>)  [unwired: 2 in, 2 out]
                    }
                  }
                  frame True {
                    n387 = for {
                      shift-right: [w1084] -> w1082
                      shift-left: w1080 -> [w1085]
                      tunnel: string[] ["SET TIMER 5", "CLOSE CLAW", ""] -> [w1083] mode=indexing
                      n388 = Enqueue Element(queue=w1085, element=w1083) -> (queue out=w1084:refnum<queue>)  [unwired: 2 in, 2 out]
                    }
                  }
                }
                n389 = Or(x=w1068, y=w1067) -> (x .or. y?=w1070:bool)
                n390 = Select(t=State_Type_Definitions,_for_0.26g_versions_and_later_2."True Stop" ("Enum"), s=w1067, f=State_Type_Definitions,_for_0.26g_versions_and_later_2."Task 5G: CLOSE CLAW" ("Enum")) -> (s? t:f=w1064:T6)
                n391 = Select(t=w1064, s=w1070, f=State_Type_Definitions,_for_0.26g_versions_and_later_2."Task 5F: ARM GRAB HEIGHT" ("Enum")) -> (s? t:f=w1069:T6)
              }
              frame "Exit" {
                n392 = for {
                  shift-right: [w1092] -> w1089
                  shift-left: w1086 -> [w1093]
                  tunnel: string[] ["STOP", "RESET ENCODERS", "RESET YAW", "ARDUINO MODE 0"] -> [w1091] mode=indexing
                  n393 = Enqueue Element(queue=w1093, element=w1091) -> (queue out=w1092:refnum<queue>)  [unwired: 2 in, 2 out]
                }
              }
            }
          }
          frame 22 {
            # ">>> yStepper command>>>"
            # ">> Manual override >>"
            n394 = Dequeue Element(queue=w1103, timeout in ms (-1)=w1102, error in (no error)=w1101) -> (element=w1100:T7)  [unwired: 3 out]
            n395 = case shown="\"None\", Default" w1100 {
              tunnel: [w1112 State_Type_Definitions,_for_0.26g_versions_and_later_2."True Stop" ("Enum")] -> w1105
              tunnel: [w1115 w1132] -> w1098
              tunnel: [State_Type_Definitions,_for_0.26g_versions_and_later_2."Idle" ("Enum") State_Type_Definitions,_for_0.26g_versions_and_later_2."Shutdown" ("Enum")] -> w1097
              tunnel: w1099 -> [w1106 _]
              tunnel: w1104 -> [w1111 w1129]
              tunnel: w1095 -> [w1110 _]
              frame "None", Default {
                # ">> Is time up? >>"
                # "Determines if object is in range to pick up"
                # ">> Manual override >>"
                n396 = case shown="True" w1110 {
                  tunnel: [w1119 w1125] -> w1115
                  tunnel: w1111 -> [w1117 w1123]
                  frame False {
                    n397 = for {
                      tunnel: string[] ["CLOSE CLAW", "START TIMER"] ("element") -> [w1120] mode=indexing
                      shift-right: [w1122] -> w1119
                      shift-left: w1117 -> [w1121]
                      n398 = Enqueue Element(queue=w1121, element=w1120) -> (queue out=w1122:refnum<queue>)  [unwired: 2 in, 2 out]
                    }
                  }
                  frame True {
                    n399 = for {
                      shift-right: [w1127] -> w1125
                      shift-left: w1123 -> [w1128]
                      tunnel: string[] ["READ STEPPER VALUES", "", ""] -> [w1126] mode=indexing
                      n400 = Enqueue Element(queue=w1128, element=w1126) -> (queue out=w1127:refnum<queue>)  [unwired: 2 in, 2 out]
                    }
                  }
                }
                n401 = Or(x=w1110, y=w1106) -> (x .or. y?=w1113:bool)
                n402 = Select(t=State_Type_Definitions,_for_0.26g_versions_and_later_2."True Stop" ("Enum"), s=w1106, f=State_Type_Definitions,_for_0.26g_versions_and_later_2."Task 5H: RAISE ARM" ("Enum")) -> (s? t:f=w1108:T6)
                n403 = Select(t=w1108, s=w1113, f=State_Type_Definitions,_for_0.26g_versions_and_later_2."Task 5G: CLOSE CLAW" ("Enum")) -> (s? t:f=w1112:T6)
              }
              frame "Exit" {
                n404 = for {
                  shift-right: [w1135] -> w1132
                  shift-left: w1129 -> [w1136]
                  tunnel: string[] ["STOP", "RESET ENCODERS", "RESET YAW", "ARDUINO MODE 0"] -> [w1134] mode=indexing
                  n405 = Enqueue Element(queue=w1136, element=w1134) -> (queue out=w1135:refnum<queue>)  [unwired: 2 in, 2 out]
                }
              }
            }
          }
          frame 23 {
            # ">>> yStepper command>>>"
            # ">> Manual override >>"
            n406 = Dequeue Element(queue=w1146, timeout in ms (-1)=w1145, error in (no error)=w1147) -> (element=w1144:T7)  [unwired: 3 out]
            n407 = Equal?(x=w1143, y=u8 60) -> (x = y?=w1141:bool)
            n408 = case shown="\"None\", Default" w1144 {
              tunnel: [w1157 State_Type_Definitions,_for_0.26g_versions_and_later_2."True Stop" ("Enum")] -> w1148
              tunnel: [w1160 w1177] -> w1149
              tunnel: [State_Type_Definitions,_for_0.26g_versions_and_later_2."Idle" ("Enum") State_Type_Definitions,_for_0.26g_versions_and_later_2."Shutdown" ("Enum")] -> w1150
              tunnel: w1141 -> [w1156 _]
              tunnel: w1140 -> [w1155 _]
              tunnel: w1139 -> [w1151 w1174]
              frame "None", Default {
                # "Stays in Task 5_A until stepper reaches desired \nheight"
                # "T: Go back to idle, F: Continue with task\""
                # ">> Manual override >>"
                n409 = case shown="False" w1156 {
                  tunnel: [w1164 w1170] -> w1160
                  tunnel: w1151 -> [w1162 w1168]
                  frame False {
                    n410 = for {
                      tunnel: string[] ["Z STEPPER CAM HEIGHT", "READ STEPPER VALUES"] ("element") -> [w1165] mode=indexing
                      shift-right: [w1167] -> w1164
                      shift-left: w1162 -> [w1166]
                      n411 = Enqueue Element(queue=w1166, element=w1165) -> (queue out=w1167:refnum<queue>)  [unwired: 2 in, 2 out]
                    }
                  }
                  frame True {
                    n412 = for {
                      shift-right: [w1172] -> w1170
                      shift-left: w1168 -> [w1173]
                      tunnel: string[] ["ARDUINO - ULTRASONIC", "READ ULTRASONIC", ""] -> [w1171] mode=indexing
                      n413 = Enqueue Element(queue=w1173, element=w1171) -> (queue out=w1172:refnum<queue>)  [unwired: 2 in, 2 out]
                    }
                  }
                }
                n414 = Or(x=w1156, y=w1155) -> (x .or. y?=w1158:bool)
                n415 = Select(t=State_Type_Definitions,_for_0.26g_versions_and_later_2."True Stop" ("Enum"), s=w1155, f=State_Type_Definitions,_for_0.26g_versions_and_later_2."True Stop" ("Enum")) -> (s? t:f=w1152:T6)
                n416 = Select(t=w1152, s=w1158, f=State_Type_Definitions,_for_0.26g_versions_and_later_2."Task 5H: RAISE ARM" ("Enum")) -> (s? t:f=w1157:T6)
              }
              frame "Exit" {
                n417 = for {
                  shift-right: [w1180] -> w1177
                  shift-left: w1174 -> [w1181]
                  tunnel: string[] ["STOP", "RESET ENCODERS", "RESET YAW", "ARDUINO MODE 0"] -> [w1179] mode=indexing
                  n418 = Enqueue Element(queue=w1181, element=w1179) -> (queue out=w1180:refnum<queue>)  [unwired: 2 in, 2 out]
                }
              }
            }
          }
          frame 24 {
            # ">>> yStepper command>>>"
            n419 = Dequeue Element(queue=w1190, timeout in ms (-1)=w1189, error in (no error)=w1188) -> (element=w1195:T7)  [unwired: 3 out]
            n420 = Equal?(x=w1186, y=u8 60) -> (x = y?=w1185:bool)
            n421 = case shown="\"None\", Default" w1195 {
              tunnel: [w1202 State_Type_Definitions,_for_0.26g_versions_and_later_2."True Stop" ("Enum")] -> w1193
              tunnel: [w1201 w1219] -> w1192
              tunnel: [State_Type_Definitions,_for_0.26g_versions_and_later_2."Idle" ("Enum") State_Type_Definitions,_for_0.26g_versions_and_later_2."Shutdown" ("Enum")] -> w1194
              tunnel: w1191 -> [w1197 _]
              tunnel: w1187 -> [w1199 _]
              tunnel: w1185 -> [w1196 _]
              frame "None", Default {
                n422 = case shown="False" w1196 {
                  tunnel: [w1207 w1213] -> w1201
                  tunnel: w1199 -> [w1205 w1211]
                  frame False {
                    n423 = for {
                      tunnel: string[] ["Z STEPPER CAM HEIGHT", "READ STEPPER VALUES"] ("element") -> [w1208] mode=indexing
                      shift-right: [w1210] -> w1207
                      shift-left: w1205 -> [w1209]
                      n424 = Enqueue Element(queue=w1209, element=w1208) -> (queue out=w1210:refnum<queue>)  [unwired: 2 in, 2 out]
                    }
                  }
                  frame True {
                    n425 = for {
                      shift-right: [w1215] -> w1213
                      shift-left: w1211 -> [w1216]
                      tunnel: string[] ["CAM ACQ", "OPEN LOG CAM"] -> [w1214] mode=indexing
                      n426 = Enqueue Element(queue=w1216, element=w1214) -> (queue out=w1215:refnum<queue>)  [unwired: 2 in, 2 out]
                    }
                  }
                }
                n427 = Or(x=w1196, y=w1197) -> (x .or. y?=w1198:bool)
                n428 = Select(t=State_Type_Definitions,_for_0.26g_versions_and_later_2."Task 6_B" ("Enum"), s=w1198, f=State_Type_Definitions,_for_0.26g_versions_and_later_2."Task 6_A" ("Enum")) -> (s? t:f=w1202:T6)
              }
              frame "Exit" {
                n429 = for {
                  shift-right: [w1222] -> w1219
                  shift-left: _ -> [w1223]
                  tunnel: string[] ["STOP", "RESET ENCODERS", "RESET YAW", "ARDUINO MODE 0"] -> [w1221] mode=indexing
                  n430 = Enqueue Element(queue=w1223, element=w1221) -> (queue out=w1222:refnum<queue>)  [unwired: 2 in, 2 out]
                }
              }
            }
          }
          frame 25 {
            # ">>> yStepper command>>>"
            n431 = Dequeue Element(queue=w1234, timeout in ms (-1)=w1232, error in (no error)=w1233) -> (element=w1231:T7)  [unwired: 3 out]
            n432 = case shown="\"None\", Default" w1231 {
              tunnel: [w1241 State_Type_Definitions,_for_0.26g_versions_and_later_2."True Stop" ("Enum")] -> w1227
              tunnel: [w1240 w1259] -> w1235
              tunnel: [State_Type_Definitions,_for_0.26g_versions_and_later_2."Idle" ("Enum") State_Type_Definitions,_for_0.26g_versions_and_later_2."Shutdown" ("Enum")] -> w1228
              tunnel: w1230 -> [w1236 _]
              tunnel: w1229 -> [w1238 _]
              tunnel: w1226 -> [w1237 w1256]
              frame "None", Default {
                # ">> Manual override >>"
                n433 = case shown="True" w1238 {
                  tunnel: [w1246 w1252] -> w1240
                  tunnel: w1237 -> [w1245 w1250]
                  frame False {
                    n434 = for {
                      shift-right: [w1249] -> w1246
                      shift-left: w1245 -> [w1248]
                      tunnel: string[] ["CAM ACQ", "PROCESS IMAGE", "OPEN CLAW"] -> [w1247] mode=indexing
                      n435 = Enqueue Element(queue=w1248, element=w1247) -> (queue out=w1249:refnum<queue>)  [unwired: 2 in, 2 out]
                    }
                  }
                  frame True {
                    n436 = for {
                      shift-right: [w1254] -> w1252
                      shift-left: w1250 -> [w1255]
                      tunnel: string[] ["CAM ACQ", "PROCESS IMAGE", "CLOSE CLAW"] -> [w1253] mode=indexing
                      n437 = Enqueue Element(queue=w1255, element=w1253) -> (queue out=w1254:refnum<queue>)  [unwired: 2 in, 2 out]
                    }
                  }
                }
                n438 = Select(t=State_Type_Definitions,_for_0.26g_versions_and_later_2."True Stop" ("Enum"), s=w1236, f=State_Type_Definitions,_for_0.26g_versions_and_later_2."Task 6_B" ("Enum")) -> (s? t:f=w1241:T6)
              }
              frame "Exit" {
                # ">> State after true stop >>"
                # ">> Goes to true stop >>"
                n439 = for {
                  shift-right: [w1262] -> w1259
                  shift-left: w1256 -> [w1263]
                  tunnel: string[] ["STOP", "RESET ENCODERS", "RESET YAW", ""] -> [w1261] mode=indexing
                  n440 = Enqueue Element(queue=w1263, element=w1261) -> (queue out=w1262:refnum<queue>)  [unwired: 2 in, 2 out]
                }
              }
            }
          }
          frame 26 {
          }
          frame 38 {
            # ">> Stepper height reeached >>"
            # ">>> yStepper command>>>"
            # ">> Manual override >>"
            n441 = Dequeue Element(queue=w1279, timeout in ms (-1)=w1274, error in (no error)=w1278) -> (element=w1282:T7)  [unwired: 3 out]
            n442 = Equal?(x=w1276, y=u8 60) -> (x = y?=w1280:bool)
            n443 = case shown="\"None\", Default" w1282 {
              tunnel: [w1293 State_Type_Definitions,_for_0.26g_versions_and_later_2."True Stop" ("Enum")] -> w1272
              tunnel: [w1291 w1308] -> w1271
              tunnel: w1275 -> [w1290 _]
              tunnel: w1277 -> [w1284 _]
              tunnel: [State_Type_Definitions,_for_0.26g_versions_and_later_2."Idle" ("Enum") State_Type_Definitions,_for_0.26g_versions_and_later_2."Shutdown" ("Enum")] -> w1273
              tunnel: w1280 -> [w1283 _]
              frame "None", Default {
                # ">> WIill proceed to part ii if not manual override >>"
                # ">>If ENABLE or Trigger is set to true>>"
                n444 = Or(x=w1283, y=w1284) -> (x .or. y?=w1285:bool)
                n445 = case shown="True" w1283 {
                  tunnel: [w1296 w1302] -> w1291
                  tunnel: w1290 -> [w1295 w1301]
                  frame False {
                    n446 = for {
                      shift-right: [w1298] -> w1296
                      shift-left: w1295 -> [w1299]
                      tunnel: string[] ["Z STEPPER CAM HEIGHT", "READ STEPPER VALUES"] ("element") -> [w1297] mode=indexing
                      n447 = Enqueue Element(queue=w1299, element=w1297) -> (queue out=w1298:refnum<queue>)  [unwired: 2 in, 2 out]
                    }
                  }
                  frame True {
                    n448 = for {
                      shift-right: [w1304] -> w1302
                      shift-left: w1301 -> [w1305]
                      tunnel: string[] ["ARDUINO - ULTRASONIC", "READ ULTRASONIC", "", "", "", ""] -> [w1303] mode=indexing
                      n449 = Enqueue Element(queue=w1305, element=w1303) -> (queue out=w1304:refnum<queue>)  [unwired: 2 in, 2 out]
                    }
                  }
                }
                n450 = Select(t=State_Type_Definitions,_for_0.26g_versions_and_later_2."True Stop" ("Enum"), s=w1284, f=State_Type_Definitions,_for_0.26g_versions_and_later_2."Task 9B: Rotate to Angle" ("Enum")) -> (s? t:f=w1287:T6)
                n451 = Select(t=w1287, s=w1285, f=State_Type_Definitions,_for_0.26g_versions_and_later_2."Task 9A: Raise Arm" ("Enum")) -> (s? t:f=w1293:T6)
              }
              frame "Exit" {
                n452 = for {
                  shift-right: [w1311] -> w1308
                  shift-left: _ -> [w1312]
                  tunnel: string[] ["STOP", "RESET ENCODERS", "RESET YAW", ""] -> [w1310] mode=indexing
                  n453 = Enqueue Element(queue=w1312, element=w1310) -> (queue out=w1311:refnum<queue>)  [unwired: 2 in, 2 out]
                }
              }
            }
          }
          frame 39 {
            # ">>> yStepper command>>>"
            n454 = Dequeue Element(queue=w1325, timeout in ms (-1)=w1324, error in (no error)=w1323) -> (element=w1327:T7)  [unwired: 3 out]
            n455 = In Range and Coerce(upper limit=305.0, x=w1317, lower limit=295.0) -> (In Range?=w1314:bool)  [unwired: 1 out]
            n456 = case shown="\"None\", Default" w1327 {
              tunnel: w1318 -> [w1330 _]
              tunnel: [w1338 State_Type_Definitions,_for_0.26g_versions_and_later_2."True Stop" ("Enum")] -> w1320
              tunnel: w1326 -> [w1336 w1354]
              tunnel: [w1335 w1353] -> w1319
              tunnel: [State_Type_Definitions,_for_0.26g_versions_and_later_2."Idle" ("Enum") State_Type_Definitions,_for_0.26g_versions_and_later_2."Shutdown" ("Enum")] -> w1321
              tunnel: w1314 -> [w1328 _]
              frame "None", Default {
                n457 = Or(x=w1328, y=w1330) -> (x .or. y?=w1329:bool)
                n458 = case shown="True" w1328 {
                  tunnel: w1336 -> [w1341 w1347]
                  tunnel: [w1340 w1345] -> w1335
                  frame False {
                    n459 = for {
                      shift-right: [w1343] -> w1340
                      shift-left: w1341 -> [w1344]
                      tunnel: string[] ["READ NAVX", "R-ACW"] ("element") -> [w1342] mode=indexing
                      n460 = Enqueue Element(queue=w1344, element=w1342) -> (queue out=w1343:refnum<queue>)  [unwired: 2 in, 2 out]
                    }
                  }
                  frame True {
                    n461 = for {
                      shift-right: [w1349] -> w1345
                      shift-left: w1347 -> [w1350]
                      tunnel: string[] ["STOP", "RESET ENCODERS", "RESET YAW", ""] -> [w1348] mode=indexing
                      n462 = Enqueue Element(queue=w1350, element=w1348) -> (queue out=w1349:refnum<queue>)  [unwired: 2 in, 2 out]
                    }
                  }
                }
                n463 = Select(t=State_Type_Definitions,_for_0.26g_versions_and_later_2."True Stop" ("Enum"), s=w1330, f=State_Type_Definitions."Task 9C: Rotation alignmnet") -> (s? t:f=w1332:u16)
                n464 = Select(t=w1332, s=w1329, f=State_Type_Definitions,_for_0.26g_versions_and_later_2."Task 9B: Rotate to Angle" ("Enum")) -> (s? t:f=w1338:u16)
              }
              frame "Exit" {
                n465 = for {
                  shift-right: [w1357] -> w1353
                  shift-left: w1354 -> [w1358]
                  tunnel: string[] ["STOP", "RESET ENCODERS", "RESET YAW", ""] -> [w1356] mode=indexing
                  n466 = Enqueue Element(queue=w1358, element=w1356) -> (queue out=w1357:refnum<queue>)  [unwired: 2 in, 2 out]
                }
              }
            }
          }
          frame 39 {
            # ">>> yStepper command>>>"
            n467 = Dequeue Element(queue=w1368, timeout in ms (-1)=w1367, error in (no error)=w1366) -> (element=w1369:T7)  [unwired: 3 out]
            n468 = case shown="\"None\", Default" w1369 {
              tunnel: w1364 -> [w1370 _]
              tunnel: [w1378 State_Type_Definitions,_for_0.26g_versions_and_later_2."True Stop" ("Enum")] -> w1361
              tunnel: w1365 -> [w1376 w1394]
              tunnel: [w1375 w1393] -> w1360
              tunnel: [State_Type_Definitions,_for_0.26g_versions_and_later_2."Idle" ("Enum") State_Type_Definitions,_for_0.26g_versions_and_later_2."Shutdown" ("Enum")] -> w1363
              frame "None", Default {
                n469 = case shown="True" w1370 {
                  tunnel: w1376 -> [w1381 w1387]
                  tunnel: [w1380 w1385] -> w1375
                  frame False {
                    n470 = for {
                      shift-right: [w1383] -> w1380
                      shift-left: w1381 -> [w1384]
                      tunnel: string[] ["READ IR", "FORWARD - IR ASSIST"] ("element") -> [w1382] mode=indexing
                      n471 = Enqueue Element(queue=w1384, element=w1382) -> (queue out=w1383:refnum<queue>)  [unwired: 2 in, 2 out]
                    }
                  }
                  frame True {
                    n472 = for {
                      shift-right: [w1389] -> w1385
                      shift-left: w1387 -> [w1390]
                      tunnel: string[] ["STOP", "RESET ENCODERS", "RESET YAW", ""] -> [w1388] mode=indexing
                      n473 = Enqueue Element(queue=w1390, element=w1388) -> (queue out=w1389:refnum<queue>)  [unwired: 2 in, 2 out]
                    }
                  }
                }
                n474 = Select(t=State_Type_Definitions,_for_0.26g_versions_and_later_2."True Stop" ("Enum"), s=w1370, f=State_Type_Definitions,_for_0.26g_versions_and_later_2."True Stop") -> (s? t:f=w1372:T6)
                n475 = Select(t=w1372, s=w1370, f=State_Type_Definitions."Task 9C: Rotation alignmnet" ("Enum")) -> (s? t:f=w1378:u16)
              }
              frame "Exit" {
                n476 = for {
                  shift-right: [w1397] -> w1393
                  shift-left: w1394 -> [w1398]
                  tunnel: string[] ["STOP", "RESET ENCODERS", "RESET YAW", ""] -> [w1396] mode=indexing
                  n477 = Enqueue Element(queue=w1398, element=w1396) -> (queue out=w1397:refnum<queue>)  [unwired: 2 in, 2 out]
                }
              }
            }
          }
          frame 27 {
            # ">>> yStepper command>>>"
            # ">> Manual override >>"
            n478 = Dequeue Element(queue=w1408, timeout in ms (-1)=w1407, error in (no error)=w1409) -> (element=w1406:T7)  [unwired: 3 out]
            n479 = Equal?(x=w1405, y=u8 60) -> (x = y?=w1403:bool)
            n480 = case shown="\"None\", Default" w1406 {
              tunnel: [w1419 State_Type_Definitions,_for_0.26g_versions_and_later_2."True Stop" ("Enum")] -> w1410
              tunnel: [w1422 w1439] -> w1411
              tunnel: [State_Type_Definitions,_for_0.26g_versions_and_later_2."Idle" ("Enum") State_Type_Definitions,_for_0.26g_versions_and_later_2."Shutdown" ("Enum")] -> w1412
              tunnel: w1403 -> [w1418 _]
              tunnel: w1402 -> [w1417 _]
              tunnel: w1401 -> [w1413 w1436]
              frame "None", Default {
                # "Stays in Task 5_A until stepper reaches desired \nheight"
                # "T: Go back to idle, F: Continue with task\""
                # ">> Manual override >>"
                n481 = case shown="True" w1418 {
                  tunnel: [w1426 w1432] -> w1422
                  tunnel: w1413 -> [w1424 w1430]
                  frame False {
                    n482 = for {
                      tunnel: string[] ["Z STEPPER CAM HEIGHT", "READ STEPPER VALUES"] ("element") -> [w1427] mode=indexing
                      shift-right: [w1429] -> w1426
                      shift-left: w1424 -> [w1428]
                      n483 = Enqueue Element(queue=w1428, element=w1427) -> (queue out=w1429:refnum<queue>)  [unwired: 2 in, 2 out]
                    }
                  }
                  frame True {
                    n484 = for {
                      shift-right: [w1434] -> w1432
                      shift-left: w1430 -> [w1435]
                      tunnel: string[] ["ARDUINO - ULTRASONIC", "READ ULTRASONIC", ""] -> [w1433] mode=indexing
                      n485 = Enqueue Element(queue=w1435, element=w1433) -> (queue out=w1434:refnum<queue>)  [unwired: 2 in, 2 out]
                    }
                  }
                }
                n486 = Or(x=w1418, y=w1417) -> (x .or. y?=w1420:bool)
                n487 = Select(t=State_Type_Definitions,_for_0.26g_versions_and_later_2."True Stop" ("Enum"), s=w1417, f=State_Type_Definitions,_for_0.26g_versions_and_later_2."Task 8B: MOVE TO BOX" ("Enum")) -> (s? t:f=w1414:T6)
                n488 = Select(t=w1414, s=w1420, f=State_Type_Definitions,_for_0.26g_versions_and_later_2."Task 8A: RAISE ARM" ("Enum")) -> (s? t:f=w1419:T6)
              }
              frame "Exit" {
                n489 = for {
                  shift-right: [w1442] -> w1439
                  shift-left: w1436 -> [w1443]
                  tunnel: string[] ["STOP", "RESET ENCODERS", "RESET YAW", "ARDUINO MODE 0"] -> [w1441] mode=indexing
                  n490 = Enqueue Element(queue=w1443, element=w1441) -> (queue out=w1442:refnum<queue>)  [unwired: 2 in, 2 out]
                }
              }
            }
          }
          frame 28 {
            w1450 = u8 20 ("y")
            # ">>> yStepper command>>>"
            n491 = Less?(x=w1447, y=w1450) -> (x < y?=w1448:bool)
            n492 = Dequeue Element(queue=w1454, timeout in ms (-1)=w1453, error in (no error)=w1455) -> (element=w1452:T7)  [unwired: 3 out]
            n493 = Less?(x=w1446, y=w1450) -> (x < y?=w1449:bool)
            n494 = And(x=w1449, y=w1448) -> (x .and. y?=w1445:bool)
            n495 = case shown="\"None\", Default" w1452 {
              tunnel: [w1467 State_Type_Definitions,_for_0.26g_versions_and_later_2."True Stop" ("Enum")] -> w1457
              tunnel: [w1470 w1487] -> w1456
              tunnel: [State_Type_Definitions,_for_0.26g_versions_and_later_2."Idle" ("Enum") State_Type_Definitions,_for_0.26g_versions_and_later_2."Shutdown" ("Enum")] -> w1458
              tunnel: w1460 -> [w1466 _]
              tunnel: w1459 -> [w1462 w1484]
              tunnel: w1445 -> [w1461 _]
              frame "None", Default {
                # "Stays in Task 5_B to capture image over 5 seconds"
                # "T: Go back to idle, F: Continue with task\""
                # ">> Manual override >>"
                n496 = case shown="False" w1461 {
                  tunnel: [w1474 w1480] -> w1470
                  tunnel: w1462 -> [w1472 w1478]
                  frame False {
                    n497 = for {
                      tunnel: string[] ["FORWARD", "READ ULTRASONIC", "READ NAVX"] ("element") -> [w1475] mode=indexing
                      shift-right: [w1477] -> w1474
                      shift-left: w1472 -> [w1476]
                      n498 = Enqueue Element(queue=w1476, element=w1475) -> (queue out=w1477:refnum<queue>)  [unwired: 2 in, 2 out]
                    }
                  }
                  frame True {
                    n499 = for {
                      shift-right: [w1482] -> w1480
                      shift-left: w1478 -> [w1483]
                      tunnel: string[] ["STOP", "RESET ENCODERS", "OPEN LOG CAM", "SET TIMER 2"] -> [w1481] mode=indexing
                      n500 = Enqueue Element(queue=w1483, element=w1481) -> (queue out=w1482:refnum<queue>)  [unwired: 2 in, 2 out]
                    }
                  }
                }
                n501 = Or(x=w1461, y=w1466) -> (x .or. y?=w1468:bool)
                n502 = Select(t=State_Type_Definitions,_for_0.26g_versions_and_later_2."True Stop" ("Enum"), s=w1466, f=State_Type_Definitions,_for_0.26g_versions_and_later_2."Task 8C: CAM BURST" ("Enum")) -> (s? t:f=w1463:T6)
                n503 = Select(t=w1463, s=w1468, f=State_Type_Definitions,_for_0.26g_versions_and_later_2."Task 8B: MOVE TO BOX" ("Enum")) -> (s? t:f=w1467:T6)
              }
              frame "Exit" {
                n504 = for {
                  shift-right: [w1490] -> w1487
                  shift-left: w1484 -> [w1491]
                  tunnel: string[] ["STOP", "RESET ENCODERS", "RESET YAW", "ARDUINO MODE 0"] -> [w1489] mode=indexing
                  n505 = Enqueue Element(queue=w1491, element=w1489) -> (queue out=w1490:refnum<queue>)  [unwired: 2 in, 2 out]
                }
              }
            }
          }
          frame 29 {
            # ">>> Motor control cluster >>>"
            # ">>> yStepper command>>>"
            # ">> Manual override >>"
            n506 = Dequeue Element(queue=w1501, timeout in ms (-1)=w1500, error in (no error)=w1499) -> (element=w1498:T7)  [unwired: 3 out]
            n507 = case shown="\"None\", Default" w1498 {
              tunnel: [w1510 State_Type_Definitions,_for_0.26g_versions_and_later_2."True Stop" ("Enum")] -> w1503
              tunnel: [w1513 w1530] -> w1496
              tunnel: [State_Type_Definitions,_for_0.26g_versions_and_later_2."Idle" ("Enum") State_Type_Definitions,_for_0.26g_versions_and_later_2."Shutdown" ("Enum")] -> w1495
              tunnel: w1497 -> [w1504 _]
              tunnel: w1502 -> [w1509 w1527]
              tunnel: w1493 -> [w1508 _]
              frame "None", Default {
                # ">> Is time up? >>"
                # "Determines if object is in range to pick up"
                # ">> Manual override >>"
                n508 = case shown="True" w1508 {
                  tunnel: [w1517 w1523] -> w1513
                  tunnel: w1509 -> [w1515 w1521]
                  frame False {
                    n509 = for {
                      tunnel: string[] ["CAM ACQ", "START TIMER"] ("element") -> [w1518] mode=indexing
                      shift-right: [w1520] -> w1517
                      shift-left: w1515 -> [w1519]
                      n510 = Enqueue Element(queue=w1519, element=w1518) -> (queue out=w1520:refnum<queue>)  [unwired: 2 in, 2 out]
                    }
                  }
                  frame True {
                    n511 = for {
                      shift-right: [w1525] -> w1523
                      shift-left: w1521 -> [w1526]
                      tunnel: string[] ["CAM CLOSE", "PROCESS IMAGE", "SET TIMER 5"] -> [w1524] mode=indexing
                      n512 = Enqueue Element(queue=w1526, element=w1524) -> (queue out=w1525:refnum<queue>)  [unwired: 2 in, 2 out]
                    }
                  }
                }
                n513 = Or(x=w1508, y=w1504) -> (x .or. y?=w1511:bool)
                n514 = Select(t=State_Type_Definitions,_for_0.26g_versions_and_later_2."True Stop" ("Enum"), s=w1504, f=State_Type_Definitions,_for_0.26g_versions_and_later_2."Task 8D: PROCESS IMAGE" ("Enum")) -> (s? t:f=w1506:T6)
                n515 = Select(t=w1506, s=w1511, f=State_Type_Definitions,_for_0.26g_versions_and_later_2."Task 8C: CAM BURST" ("Enum")) -> (s? t:f=w1510:T6)
              }
              frame "Exit" {
                n516 = for {
                  shift-right: [w1533] -> w1530
                  shift-left: w1527 -> [w1534]
                  tunnel: string[] ["STOP", "RESET ENCODERS", "RESET YAW", "ARDUINO MODE 0"] -> [w1532] mode=indexing
                  n517 = Enqueue Element(queue=w1534, element=w1532) -> (queue out=w1533:refnum<queue>)  [unwired: 2 in, 2 out]
                }
              }
            }
          }
          frame 30 {
            # ">>> yStepper command>>>"
            n518 = Dequeue Element(queue=w1541, timeout in ms (-1)=w1540, error in (no error)=w1539) -> (element=w1538:T7)  [unwired: 3 out]
            n519 = case shown="\"None\", Default" w1538 {
              tunnel: [w1553 State_Type_Definitions,_for_0.26g_versions_and_later_2."True Stop" ("Enum")] -> w1545
              tunnel: [w1556 w1573] -> w1544
              tunnel: [State_Type_Definitions,_for_0.26g_versions_and_later_2."Idle" ("Enum") State_Type_Definitions,_for_0.26g_versions_and_later_2."Shutdown" ("Enum")] -> w1546
              tunnel: w1542 -> [w1552 _]
              tunnel: w1543 -> [w1548 w1570]
              tunnel: w1536 -> [w1547 _]
              frame "None", Default {
                # ">> T: Breaks out of state loop; F: Stays in loop>>"
                # ">> Manual override >>"
                # ">> Checks if time is up>>"
                # "Stays in Task 5D until the object is detected"
                # "T: Go back to idle, F: Continue with task\""
                # ">> Manual override >>"
                n520 = case shown="False" w1547 {
                  tunnel: [w1560 w1566] -> w1556
                  tunnel: w1548 -> [w1558 w1564]
                  frame False {
                    n521 = for {
                      tunnel: string[] ["START TIMER", "PROCESS IMAGE", ""] ("element") -> [w1561] mode=indexing
                      shift-right: [w1563] -> w1560
                      shift-left: w1558 -> [w1562]
                      n522 = Enqueue Element(queue=w1562, element=w1561) -> (queue out=w1563:refnum<queue>)  [unwired: 2 in, 2 out]
                    }
                  }
                  frame True {
                    n523 = for {
                      shift-right: [w1568] -> w1566
                      shift-left: w1564 -> [w1569]
                      tunnel: string[] ["RESET ENCODERS", "", ""] -> [w1567] mode=indexing
                      n524 = Enqueue Element(queue=w1569, element=w1567) -> (queue out=w1568:refnum<queue>)  [unwired: 2 in, 2 out]
                    }
                  }
                }
                n525 = Or(x=w1547, y=w1552) -> (x .or. y?=w1554:bool)
                n526 = Select(t=State_Type_Definitions,_for_0.26g_versions_and_later_2."True Stop" ("Enum"), s=w1552, f=State_Type_Definitions,_for_0.26g_versions_and_later_2."Task 8E: ROBOT ADJUST" ("Enum")) -> (s? t:f=w1549:T6)
                n527 = Select(t=w1549, s=w1554, f=State_Type_Definitions,_for_0.26g_versions_and_later_2."Task 8D: PROCESS IMAGE" ("Enum")) -> (s? t:f=w1553:T6)
              }
              frame "Exit" {
                n528 = for {
                  shift-right: [w1576] -> w1573
                  shift-left: w1570 -> [w1577]
                  tunnel: string[] ["STOP", "RESET ENCODERS", "RESET YAW", "ARDUINO MODE 0"] -> [w1575] mode=indexing
                  n529 = Enqueue Element(queue=w1577, element=w1575) -> (queue out=w1576:refnum<queue>)  [unwired: 2 in, 2 out]
                }
              }
            }
          }
          frame 31 {
            # ">>> Motor control cluster >>>"
            # ">>> yStepper command>>>"
            n530 = Dequeue Element(queue=w1593, timeout in ms (-1)=w1592, error in (no error)=w1591) -> (element=w1590:T7)  [unwired: 3 out]
            n531 = Subtract(x=w1588, y=300.0) -> (x-y=w1586:dbl)
            "x-y" <- w1586
            n532 = formula code="if (error < -80 && error >-300){\ndistance = -20;\nxSpeed = -30;\n}\n\nelse if (error <= 61&&error >= -80){\ndistance = -15;\nxSpeed = -30;\n}\n\nelse if (error <= -26 && error >= -60){\ndistance = -10;\nxSpeed = -30;\n}\n\nelse if (error >= -25 && error <= 25){\ndistance = 0;\nxSpeed = 0;\n}\n\nelse if (error >= 51 && error <= 80){\ndistance = 10;\nxSpeed = 30;\n}\n\nelse if (error >= 81 && error <= 100){\ndistance = 15;\nxSpeed = 30;\n}\n\nelse if (error >= 101 && error <= 120){\ndistance = 20;\nxSpeed = 30;\n}\n\nelse if (error >= 121 && error <= 150){\ndistance = 25;\nxSpeed = 30;\n}\n\nelse if (error < 250){\ndistance = 30;\nxSpeed = 30;\n}\n\nelse{\ndistance = 0;\nxSpeed = 0;\n}"("error"=w1586) -> ("distance"=w1581:dbl, "xSpeed"=w1583:dbl)
            n533 = formula code="if (target > 0){\nif (current  >= target)\noutput = 1;\n}\n\nelse if (target == 0){\nif (current == target)\noutput = 1;\n}\n\nelse if (target < 0){\nif (current <= target)\noutput = 1;\n}\n\nelse\noutput = 0;"("target"=w1581, "current"=w1582) -> ("output"=w1580:dbl)
            n534 = Bundle By Name(cluster=w1585, "xSpeed"=w1583) -> (w1584:T8)
            n535 = Equal?(x=w1580, y=1.0) -> (x = y?=w1578:bool)
            n536 = case shown="\"None\", Default" w1590 {
              tunnel: [w1605 State_Type_Definitions,_for_0.26g_versions_and_later_2."True Stop" ("Enum")] -> w1597
              tunnel: [w1608 w1625] -> w1596
              tunnel: [State_Type_Definitions,_for_0.26g_versions_and_later_2."Idle" ("Enum") State_Type_Definitions,_for_0.26g_versions_and_later_2."Shutdown" ("Enum")] -> w1598
              tunnel: w1594 -> [w1604 _]
              tunnel: w1595 -> [w1600 w1622]
              tunnel: w1578 -> [w1599 _]
              frame "None", Default {
                # ">> T: Breaks out of state loop; F: Stays in loop>>"
                # ">> Manual override >>"
                # ">> Checks if time is up>>"
                # "Stays in Task 5D until the object is detected"
                # "T: Go back to idle, F: Continue with task\""
                # ">> Manual override >>"
                n537 = case shown="True" w1599 {
                  tunnel: [w1612 w1618] -> w1608
                  tunnel: w1600 -> [w1610 w1616]
                  frame False {
                    n538 = for {
                      tunnel: string[] ["X AXIS - SLOW", "READ ENCODERS", "READ YAW"] ("element") -> [w1613] mode=indexing
                      shift-right: [w1615] -> w1612
                      shift-left: w1610 -> [w1614]
                      n539 = Enqueue Element(queue=w1614, element=w1613) -> (queue out=w1615:refnum<queue>)  [unwired: 2 in, 2 out]
                    }
                  }
                  frame True {
                    n540 = for {
                      shift-right: [w1620] -> w1618
                      shift-left: w1616 -> [w1621]
                      tunnel: string[] ["SET TIMER 2", "STOP", "READ STEPPER VALUES", ""] -> [w1619] mode=indexing
                      n541 = Enqueue Element(queue=w1621, element=w1619) -> (queue out=w1620:refnum<queue>)  [unwired: 2 in, 2 out]
                    }
                  }
                }
                n542 = Or(x=w1599, y=w1604) -> (x .or. y?=w1606:bool)
                n543 = Select(t=State_Type_Definitions,_for_0.26g_versions_and_later_2."True Stop" ("Enum"), s=w1604, f=State_Type_Definitions,_for_0.26g_versions_and_later_2."Task 8H: ARM ADJUST" ("Enum")) -> (s? t:f=w1601:T6)
                n544 = Select(t=w1601, s=w1606, f=State_Type_Definitions,_for_0.26g_versions_and_later_2."Task 8E: ROBOT ADJUST" ("Enum")) -> (s? t:f=w1605:T6)
              }
              frame "Exit" {
                n545 = for {
                  shift-right: [w1628] -> w1625
                  shift-left: w1622 -> [w1629]
                  tunnel: string[] ["STOP", "RESET ENCODERS", "RESET YAW", "ARDUINO MODE 0"] -> [w1627] mode=indexing
                  n546 = Enqueue Element(queue=w1629, element=w1627) -> (queue out=w1628:refnum<queue>)  [unwired: 2 in, 2 out]
                }
              }
            }
          }
          frame 32 {
            # ">>> Motor control cluster >>>"
            # ">>> yStepper command>>>"
            # ">> Manual override >>"
            n547 = Dequeue Element(queue=w1639, timeout in ms (-1)=w1638, error in (no error)=w1637) -> (element=w1636:T7)  [unwired: 3 out]
            n548 = case shown="\"None\", Default" w1636 {
              tunnel: [w1648 State_Type_Definitions,_for_0.26g_versions_and_later_2."True Stop" ("Enum")] -> w1641
              tunnel: [w1651 w1668] -> w1634
              tunnel: [State_Type_Definitions,_for_0.26g_versions_and_later_2."Idle" ("Enum") State_Type_Definitions,_for_0.26g_versions_and_later_2."Shutdown" ("Enum")] -> w1633
              tunnel: w1635 -> [w1642 _]
              tunnel: w1640 -> [w1647 w1665]
              tunnel: w1631 -> [w1646 _]
              frame "None", Default {
                # ">> Is time up? >>"
                # "Determines if object is in range to pick up"
                # ">> Manual override >>"
                n549 = case shown="True" w1646 {
                  tunnel: [w1655 w1661] -> w1651
                  tunnel: w1647 -> [w1653 w1659]
                  frame False {
                    n550 = for {
                      tunnel: string[] ["CAM ACQ", "START TIMER"] ("element") -> [w1656] mode=indexing
                      shift-right: [w1658] -> w1655
                      shift-left: w1653 -> [w1657]
                      n551 = Enqueue Element(queue=w1657, element=w1656) -> (queue out=w1658:refnum<queue>)  [unwired: 2 in, 2 out]
                    }
                  }
                  frame True {
                    n552 = for {
                      shift-right: [w1663] -> w1661
                      shift-left: w1659 -> [w1664]
                      tunnel: string[] ["CAM CLOSE", "PROCESS IMAGE", "SET TIMER 3"] -> [w1662] mode=indexing
                      n553 = Enqueue Element(queue=w1664, element=w1662) -> (queue out=w1663:refnum<queue>)  [unwired: 2 in, 2 out]
                    }
                  }
                }
                n554 = Or(x=w1646, y=w1642) -> (x .or. y?=w1649:bool)
                n555 = Select(t=State_Type_Definitions,_for_0.26g_versions_and_later_2."True Stop" ("Enum"), s=w1642, f=State_Type_Definitions,_for_0.26g_versions_and_later_2."Task 8G: PROCESS IMAGE 2" ("Enum")) -> (s? t:f=w1644:T6)
                n556 = Select(t=w1644, s=w1649, f=State_Type_Definitions,_for_0.26g_versions_and_later_2."Task 8F: CAM BURST 2" ("Enum")) -> (s? t:f=w1648:T6)
              }
              frame "Exit" {
                n557 = for {
                  shift-right: [w1671] -> w1668
                  shift-left: w1665 -> [w1672]
                  tunnel: string[] ["STOP", "RESET ENCODERS", "RESET YAW", "ARDUINO MODE 0"] -> [w1670] mode=indexing
                  n558 = Enqueue Element(queue=w1672, element=w1670) -> (queue out=w1671:refnum<queue>)  [unwired: 2 in, 2 out]
                }
              }
            }
          }
          frame 33 {
            # ">>> yStepper command>>>"
            n559 = Dequeue Element(queue=w1679, timeout in ms (-1)=w1678, error in (no error)=w1677) -> (element=w1676:T7)  [unwired: 3 out]
            n560 = case shown="\"None\", Default" w1676 {
              tunnel: [w1691 State_Type_Definitions,_for_0.26g_versions_and_later_2."True Stop" ("Enum")] -> w1683
              tunnel: [w1694 w1711] -> w1682
              tunnel: [State_Type_Definitions,_for_0.26g_versions_and_later_2."Idle" ("Enum") State_Type_Definitions,_for_0.26g_versions_and_later_2."Shutdown" ("Enum")] -> w1684
              tunnel: w1680 -> [w1690 _]
              tunnel: w1681 -> [w1686 w1708]
              tunnel: w1674 -> [w1685 _]
              frame "None", Default {
                # ">> T: Breaks out of state loop; F: Stays in loop>>"
                # ">> Manual override >>"
                # ">> Checks if time is up>>"
                # "Stays in Task 5D until the object is detected"
                # "T: Go back to idle, F: Continue with task\""
                # ">> Manual override >>"
                n561 = case shown="True" w1685 {
                  tunnel: [w1698 w1704] -> w1694
                  tunnel: w1686 -> [w1696 w1702]
                  frame False {
                    n562 = for {
                      tunnel: string[] ["START TIMER", "PROCESS IMAGE", ""] ("element") -> [w1699] mode=indexing
                      shift-right: [w1701] -> w1698
                      shift-left: w1696 -> [w1700]
                      n563 = Enqueue Element(queue=w1700, element=w1699) -> (queue out=w1701:refnum<queue>)  [unwired: 2 in, 2 out]
                    }
                  }
                  frame True {
                    n564 = for {
                      shift-right: [w1706] -> w1704
                      shift-left: w1702 -> [w1707]
                      tunnel: string[] ["READ STEPPER VALUES", "Y STEPPER CONTROL", ""] -> [w1705] mode=indexing
                      n565 = Enqueue Element(queue=w1707, element=w1705) -> (queue out=w1706:refnum<queue>)  [unwired: 2 in, 2 out]
                    }
                  }
                }
                n566 = Or(x=w1685, y=w1690) -> (x .or. y?=w1692:bool)
                n567 = Select(t=State_Type_Definitions,_for_0.26g_versions_and_later_2."True Stop" ("Enum"), s=w1690, f=State_Type_Definitions,_for_0.26g_versions_and_later_2."Task 8H: ARM ADJUST" ("Enum")) -> (s? t:f=w1687:T6)
                n568 = Select(t=w1687, s=w1692, f=State_Type_Definitions,_for_0.26g_versions_and_later_2."Task 8G: PROCESS IMAGE 2" ("Enum")) -> (s? t:f=w1691:T6)
              }
              frame "Exit" {
                n569 = for {
                  shift-right: [w1714] -> w1711
                  shift-left: w1708 -> [w1715]
                  tunnel: string[] ["STOP", "RESET ENCODERS", "RESET YAW", "ARDUINO MODE 0"] -> [w1713] mode=indexing
                  n570 = Enqueue Element(queue=w1715, element=w1713) -> (queue out=w1714:refnum<queue>)  [unwired: 2 in, 2 out]
                }
              }
            }
          }
          frame 34 {
            # ">>> yStepper command>>>"
            n571 = Dequeue Element(queue=w1728, timeout in ms (-1)=w1729, error in (no error)=w1730) -> (element=w1732:T7)  [unwired: 3 out]
            n572 = formula code="if (pos <= 81)\ny = 40;\n\nelse if (pos >= 81 &&pos <= 120)\ny = 35;\n\nelse if (pos >= 121 && pos <= 140)\ny = 28;\n\nelse if (pos >= 141 && pos <= 170)\ny = 25;\n\nelse if (pos >= 171 &&pos <= 180) \ny = 20;\n\nelse if (pos >= 181&& pos <= 200)\ny = 15;\n\nelse if (pos >= 201 && pos <= 230)\ny = 10;\n\nelse if (pos >= 231 && pos <= 320)\ny = 8;\n\nelse if (pos > 320)\ny = 0;"("pos"=w1720) -> ("y"=w1723:dbl)
            n573 = To Unsigned Byte Integer(number=w1723) -> (unsigned 8bit integer=w1718:u8)
            n574 = Equal?(x=w1719, y=w1718) -> (x = y?=w1717:bool)
            n575 = case shown="\"None\", Default" w1732 {
              tunnel: [w1739 State_Type_Definitions,_for_0.26g_versions_and_later_2."True Stop" ("Enum")] -> w1726
              tunnel: [w1742 w1759] -> w1724
              tunnel: [State_Type_Definitions,_for_0.26g_versions_and_later_2."Idle" ("Enum") State_Type_Definitions,_for_0.26g_versions_and_later_2."Shutdown" ("Enum")] -> w1725
              tunnel: w1731 -> [w1738 _]
              tunnel: w1727 -> [w1734 w1756]
              tunnel: w1717 -> [w1733 _]
              frame "None", Default {
                # ">> T: Breaks out of state loop; F: Stays in loop>>"
                # ">> Manual override >>"
                # ">> Checks if time is up>>"
                # "Stays in Task 5D until the object is detected"
                # "T: Go back to idle, F: Continue with task\""
                # ">> Manual override >>"
                n576 = case shown="True" w1733 {
                  tunnel: [w1746 w1752] -> w1742
                  tunnel: w1734 -> [w1744 w1750]
                  frame False {
                    n577 = for {
                      tunnel: string[] ["READ STEPPER VALUES", "Y STEPPER CONTROL", ""] ("element") -> [w1747] mode=indexing
                      shift-right: [w1749] -> w1746
                      shift-left: w1744 -> [w1748]
                      n578 = Enqueue Element(queue=w1748, element=w1747) -> (queue out=w1749:refnum<queue>)  [unwired: 2 in, 2 out]
                    }
                  }
                  frame True {
                    n579 = for {
                      shift-right: [w1754] -> w1752
                      shift-left: w1750 -> [w1755]
                      tunnel: string[] ["DISPOSE BUFFERS", "READ STEPPER VALUES", ""] -> [w1753] mode=indexing
                      n580 = Enqueue Element(queue=w1755, element=w1753) -> (queue out=w1754:refnum<queue>)  [unwired: 2 in, 2 out]
                    }
                  }
                }
                n581 = Or(x=w1733, y=w1738) -> (x .or. y?=w1740:bool)
                n582 = Select(t=State_Type_Definitions,_for_0.26g_versions_and_later_2."True Stop" ("Enum"), s=w1738, f=State_Type_Definitions,_for_0.26g_versions_and_later_2."Task 8I: ARM GRAB HEIGHT" ("Enum")) -> (s? t:f=w1735:T6)
                n583 = Select(t=w1735, s=w1740, f=State_Type_Definitions,_for_0.26g_versions_and_later_2."Task 8H: ARM ADJUST" ("Enum")) -> (s? t:f=w1739:T6)
              }
              frame "Exit" {
                n584 = for {
                  shift-right: [w1762] -> w1759
                  shift-left: w1756 -> [w1763]
                  tunnel: string[] ["STOP", "RESET ENCODERS", "RESET YAW", "ARDUINO MODE 0"] -> [w1761] mode=indexing
                  n585 = Enqueue Element(queue=w1763, element=w1761) -> (queue out=w1762:refnum<queue>)  [unwired: 2 in, 2 out]
                }
              }
            }
            n586 = Bundle By Name(cluster=w1722, "yStepper desired"=w1718) -> (w1721:T10)
          }
          frame 35 {
            # ">>> Motor control cluster >>>"
            # ">>> yStepper command>>>"
            # ">> Manual override >>"
            n587 = Dequeue Element(queue=w1773, timeout in ms (-1)=w1772, error in (no error)=w1774) -> (element=w1771:T7)  [unwired: 3 out]
            n588 = Equal?(x=w1770, y=u8 1) -> (x = y?=w1768:bool)
            n589 = case shown="\"None\", Default" w1771 {
              tunnel: [w1784 State_Type_Definitions,_for_0.26g_versions_and_later_2."True Stop" ("Enum")] -> w1775
              tunnel: [w1787 w1804] -> w1776
              tunnel: [State_Type_Definitions,_for_0.26g_versions_and_later_2."Idle" ("Enum") State_Type_Definitions,_for_0.26g_versions_and_later_2."Shutdown" ("Enum")] -> w1777
              tunnel: w1768 -> [w1783 _]
              tunnel: w1767 -> [w1782 _]
              tunnel: w1766 -> [w1778 w1801]
              frame "None", Default {
                # "Stays in Task 5F until stepper reaches desired \nheight"
                # "T: Go back to idle, F: Continue with task\""
                # ">> Manual override >>"
                n590 = case shown="True" w1783 {
                  tunnel: [w1791 w1797] -> w1787
                  tunnel: w1778 -> [w1789 w1795]
                  frame False {
                    n591 = for {
                      tunnel: string[] ["Z STEPPER GRAB HEIGHT", "READ STEPPER VALUES"] ("element") -> [w1792] mode=indexing
                      shift-right: [w1794] -> w1791
                      shift-left: w1789 -> [w1793]
                      n592 = Enqueue Element(queue=w1793, element=w1792) -> (queue out=w1794:refnum<queue>)  [unwired: 2 in, 2 out]
                    }
                  }
                  frame True {
                    n593 = for {
                      shift-right: [w1799] -> w1797
                      shift-left: w1795 -> [w1800]
                      tunnel: string[] ["SET TIMER 2", "CLOSE CLAW", ""] -> [w1798] mode=indexing
                      n594 = Enqueue Element(queue=w1800, element=w1798) -> (queue out=w1799:refnum<queue>)  [unwired: 2 in, 2 out]
                    }
                  }
                }
                n595 = Or(x=w1783, y=w1782) -> (x .or. y?=w1785:bool)
                n596 = Select(t=State_Type_Definitions,_for_0.26g_versions_and_later_2."True Stop" ("Enum"), s=w1782, f=State_Type_Definitions,_for_0.26g_versions_and_later_2."Task 8J: CLOSE CLAW" ("Enum")) -> (s? t:f=w1779:T6)
                n597 = Select(t=w1779, s=w1785, f=State_Type_Definitions,_for_0.26g_versions_and_later_2."Task 8I: ARM GRAB HEIGHT" ("Enum")) -> (s? t:f=w1784:T6)
              }
              frame "Exit" {
                n598 = for {
                  shift-right: [w1807] -> w1804
                  shift-left: w1801 -> [w1808]
                  tunnel: string[] ["STOP", "RESET ENCODERS", "RESET YAW", "ARDUINO MODE 0"] -> [w1806] mode=indexing
                  n599 = Enqueue Element(queue=w1808, element=w1806) -> (queue out=w1807:refnum<queue>)  [unwired: 2 in, 2 out]
                }
              }
            }
          }
          frame 36 {
            # ">>> yStepper command>>>"
            # ">> Manual override >>"
            n600 = Dequeue Element(queue=w1818, timeout in ms (-1)=w1817, error in (no error)=w1816) -> (element=w1815:T7)  [unwired: 3 out]
            n601 = case shown="\"None\", Default" w1815 {
              tunnel: [w1827 State_Type_Definitions,_for_0.26g_versions_and_later_2."True Stop" ("Enum")] -> w1820
              tunnel: [w1830 w1847] -> w1813
              tunnel: [State_Type_Definitions,_for_0.26g_versions_and_later_2."Idle" ("Enum") State_Type_Definitions,_for_0.26g_versions_and_later_2."Shutdown" ("Enum")] -> w1812
              tunnel: w1814 -> [w1821 _]
              tunnel: w1819 -> [w1826 w1844]
              tunnel: w1810 -> [w1825 _]
              frame "None", Default {
                # ">> Is time up? >>"
                # "Determines if object is in range to pick up"
                # ">> Manual override >>"
                n602 = case shown="True" w1825 {
                  tunnel: [w1834 w1840] -> w1830
                  tunnel: w1826 -> [w1832 w1838]
                  frame False {
                    n603 = for {
                      tunnel: string[] ["CLOSE CLAW", "START TIMER"] ("element") -> [w1835] mode=indexing
                      shift-right: [w1837] -> w1834
                      shift-left: w1832 -> [w1836]
                      n604 = Enqueue Element(queue=w1836, element=w1835) -> (queue out=w1837:refnum<queue>)  [unwired: 2 in, 2 out]
                    }
                  }
                  frame True {
                    n605 = for {
                      shift-right: [w1842] -> w1840
                      shift-left: w1838 -> [w1843]
                      tunnel: string[] ["READ STEPPER VALUES", "", ""] -> [w1841] mode=indexing
                      n606 = Enqueue Element(queue=w1843, element=w1841) -> (queue out=w1842:refnum<queue>)  [unwired: 2 in, 2 out]
                    }
                  }
                }
                n607 = Or(x=w1825, y=w1821) -> (x .or. y?=w1828:bool)
                n608 = Select(t=State_Type_Definitions,_for_0.26g_versions_and_later_2."True Stop" ("Enum"), s=w1821, f=State_Type_Definitions,_for_0.26g_versions_and_later_2."Task 8K: RAISE MY SWORD" ("Enum")) -> (s? t:f=w1823:T6)
                n609 = Select(t=w1823, s=w1828, f=State_Type_Definitions,_for_0.26g_versions_and_later_2."Task 8J: CLOSE CLAW" ("Enum")) -> (s? t:f=w1827:T6)
              }
              frame "Exit" {
                n610 = for {
                  shift-right: [w1850] -> w1847
                  shift-left: w1844 -> [w1851]
                  tunnel: string[] ["STOP", "RESET ENCODERS", "RESET YAW", "ARDUINO MODE 0"] -> [w1849] mode=indexing
                  n611 = Enqueue Element(queue=w1851, element=w1849) -> (queue out=w1850:refnum<queue>)  [unwired: 2 in, 2 out]
                }
              }
            }
          }
          frame 37 {
            # ">>> yStepper command>>>"
            # ">> Manual override >>"
            n612 = Dequeue Element(queue=w1861, timeout in ms (-1)=w1860, error in (no error)=w1862) -> (element=w1859:T7)  [unwired: 3 out]
            n613 = Equal?(x=w1858, y=u8 60) -> (x = y?=w1856:bool)
            n614 = case shown="\"None\", Default" w1859 {
              tunnel: [w1872 State_Type_Definitions,_for_0.26g_versions_and_later_2."True Stop" ("Enum")] -> w1863
              tunnel: [w1875 w1892] -> w1864
              tunnel: [State_Type_Definitions,_for_0.26g_versions_and_later_2."Idle" ("Enum") State_Type_Definitions,_for_0.26g_versions_and_later_2."Shutdown" ("Enum")] -> w1865
              tunnel: w1856 -> [w1871 _]
              tunnel: w1855 -> [w1870 _]
              tunnel: w1854 -> [w1866 w1889]
              frame "None", Default {
                # "Stays in Task 5_A until stepper reaches desired \nheight"
                # "T: Go back to idle, F: Continue with task\""
                # ">> Manual override >>"
                n615 = case shown="True" w1871 {
                  tunnel: [w1879 w1885] -> w1875
                  tunnel: w1866 -> [w1877 w1883]
                  frame False {
                    n616 = for {
                      tunnel: string[] ["Z STEPPER CAM HEIGHT", "READ STEPPER VALUES"] ("element") -> [w1880] mode=indexing
                      shift-right: [w1882] -> w1879
                      shift-left: w1877 -> [w1881]
                      n617 = Enqueue Element(queue=w1881, element=w1880) -> (queue out=w1882:refnum<queue>)  [unwired: 2 in, 2 out]
                    }
                  }
                  frame True {
                    n618 = for {
                      shift-right: [w1887] -> w1885
                      shift-left: w1883 -> [w1888]
                      tunnel: string[] ["CAM CLOSE", "DISPOSE BUFFERS", ""] -> [w1886] mode=indexing
                      n619 = Enqueue Element(queue=w1888, element=w1886) -> (queue out=w1887:refnum<queue>)  [unwired: 2 in, 2 out]
                    }
                  }
                }
                n620 = Or(x=w1871, y=w1870) -> (x .or. y?=w1873:bool)
                n621 = Select(t=State_Type_Definitions,_for_0.26g_versions_and_later_2."True Stop" ("Enum"), s=w1870, f=State_Type_Definitions,_for_0.26g_versions_and_later_2."True Stop" ("Enum")) -> (s? t:f=w1867:T6)
                n622 = Select(t=w1867, s=w1873, f=State_Type_Definitions,_for_0.26g_versions_and_later_2."Task 8K: RAISE MY SWORD" ("Enum")) -> (s? t:f=w1872:T6)
              }
              frame "Exit" {
                n623 = for {
                  shift-right: [w1895] -> w1892
                  shift-left: w1889 -> [w1896]
                  tunnel: string[] ["STOP", "RESET ENCODERS", "RESET YAW", "ARDUINO MODE 0"] -> [w1894] mode=indexing
                  n624 = Enqueue Element(queue=w1896, element=w1894) -> (queue out=w1895:refnum<queue>)  [unwired: 2 in, 2 out]
                }
              }
            }
          }
        }
      }
    }
    n625 = local write "Green LED"(w189) -> ()
  }
  n626 = while {
    tunnel: w48 -> [w2476]
    tunnel: w47 -> [w2473]
    stop <- w2470 stop-if-true
    # "Status Loop for Action Queues"
    n627 = Get Queue Status(queue=w2476, return elements? (F)=TRUE) -> (error out=w2472:errorcluster, # elements in queue=→"Action Queue Items":i32, elements=→"Action Queues items":string[])  [unwired: 1 in, 5 out]
    n628 = Get Queue Status(queue=w2473, return elements? (F)=TRUE) -> (# pending remove=→"State Logic Queue Items":i32, error out=w2471:errorcluster, elements=→"elements":T7[])  [unwired: 1 in, 5 out]
    n629 = Merge Errors(w2472, w2471) -> (w2470:errorcluster)
    n630 = Wait (ms)(milliseconds to wait=u32 500) -> ()  [unwired: 1 out]
  }
  n631 = call <vilib>:"DIO Close.vi"("error in (no error)"=w24, "DIO Info In"=w27) -> ()  [unwired: 9 in, 1 out]
  n632 = call <vilib>:"DIO Close.vi"("error in (no error)"=w34, "DIO Info In"=w36) -> ()  [unwired: 9 in, 1 out]
  n633 = call <vilib>:"NavX Close.vi"("error in (no error)"=w8, "NavX Info In"=w7) -> ()  [unwired: 9 in, 1 out]
  n634 = call <vilib>:"DIO Close.vi"("error in (no error)"=w29, "DIO Info In"=w31) -> ()  [unwired: 9 in, 1 out]
  n635 = call <vilib>:"DIO Close.vi"("error in (no error)"=w15, "DIO Info In"=w16) -> ()  [unwired: 9 in, 1 out]
  n636 = call <vilib>:"DIO Close.vi"("error in (no error)"=w10, "DIO Info In"=w11) -> ()  [unwired: 9 in, 1 out]
  n637 = while {
    stop <- w2480 stop-if-true
    n638 = call <vilib>:"RT Get CPU Loads.vi"() -> ("CPU loads"=→"CPU loads":T5[])  [unwired: 10 in, 1 out]
    n639 = Wait (ms)(milliseconds to wait=u32 100) -> ()  [unwired: 1 out]
    n640 = call "FGV Bool.vi"("Init/Read/Write State"=States_for_Action_Engine."Read") -> ("Output node"=w2480:bool)  [unwired: 2 in, 1 out]
  }
  n641 = while {
    stop <- w2484 stop-if-true
    n642 = call "MOTOR CONTROL WITH PID AE.vi"("AE Mode"=MOTOR_CONTROL_WITH_PID_AE_DATA_MODE_TYPE_DEF."Read from AE") -> ("Speed & distance"=→"Speed & distance":T1)  [unwired: 3 in]
    n643 = call "FGV Bool.vi"("Init/Read/Write State"=States_for_Action_Engine."Read") -> ("Output node"=w2484:bool)  [unwired: 2 in, 1 out]
    n644 = Wait (ms)(milliseconds to wait=u32 5) -> ()  [unwired: 1 out]
  }
  n645 = Merge Errors "Merge Errors"(w64, w63) -> (w46:errorcluster)
  n646 = Merge Errors(w50, w46) -> (w45:errorcluster)
  n647 = Destroy User Event(user event=w67, error in=w45) -> ()  [unwired: 1 out]
  n648 = Destroy User Event(user event=w68, error in=w45) -> ()  [unwired: 1 out]
  n649 = Unregister For Events(event registration refnum=w59, error in=w45) -> ()  [unwired: 1 out]
  n650 = Release Queue(queue=w41, error in (no error)=w45) -> (error out=→"error out":errorcluster)  [unwired: 1 in, 2 out]
  n651 = Release Queue(queue=w58, error in (no error)=w45) -> ()  [unwired: 1 in, 3 out]
